vi "PVCamApp.vi"() -> ()   [LabVIEW 2019]
uses:
  <vilib>/Utility/miscctls.llb/LVMouseTypeDef.ctl
  Dependencies/PVCamNET.dll
  <vilib>/Analysis/coordinate.llb/2D Cartesian Coordinate Rotation (Scalar).vi
  SubVis/PVCamGlobalVariables.vi
  <vilib>/Instr/_visa.llb/VISA Configure Serial Port (Instr).vi
  Program Files/MetroCon-3.2/RepSend/R11CommLib-x64.dll
  <vilib>/Analysis/NI_AALPro.lvlib
panel:
  in  "FramesToCapture":u16=188
  in  "value":u16=700
  out "Map":picture
  out "Mouse":T1={"Mouse Position"={"X"=-1, "Y"=-1}, "Mouse Modifiers"={"Button Down"=FALSE, "Shift Mod"=FALSE, "Menu Mod"=FALSE, "Option Mod"=FALSE}}
  in  "ScreenMove":bool
  out "Angle":dbl=5.764762550937391
  out "Ratio":dbl=0.06396544799868786
  out "Shift2":dbl=-46.0
  out "Shift1":dbl=3014.0
  in  "Match":bool
  in  "map2":bool
  in  "map1":bool
  in  "Get2":bool
  in  "Get1":bool
  out "StageY2":i32=-305
  out "StageX2":i32=3018
  out "StageY1":i32=287
  out "StageX1":i32=-2846
  out "MapY2":i32=226
  out "MapX2":i32=590
  out "MapY1":i32=226
  out "MapX1":i32=213
  out "new picture":picture
  in  "StopX":bool
  in  "Path":path=path "C:/Users/Dell/Desktop/Map1.jpg"
  in  "LoadMap":bool
  in  "Stop":bool=TRUE
  out "Current PositionY":string="-2147431906" caption="Current PositionY:"
  out "Current PositionX":string="2147391745" caption="Current PositionX:"
  out "Choice 2":i32
  out "Choice":i32
  in  "Delete":bool
  in  "homeZ":bool
  in  "Goto":bool
  in  "Update":bool
  in  "ADDItem":bool
  in  "Multicolumn Listbox":i32[](listbox)=[0]
  in  "JogX-":bool
  in  "JogX+":bool
  out "Z motor connect":bool=TRUE
  out "XY motors connect":bool=TRUE
  out "appended path":path=path "C:/Users/Dell/Desktop/SIMImaging -电动平移台 -V4/PVCamNET_Collection1621317453_1973.tiff"
  in  "Numeric 2":i32=100
  out "Current PositionZ:":string="5661"
  in  "GoZ":bool
  in  "Relative MoveZ":string="3" caption="Relative Move:"
  in  "GoZ 2":bool
  in  "ZeroZ":bool
  out "Laser":bool[](array[boolean])=[FALSE, FALSE, TRUE]
  out "XBinning 3":u16
  out "YBinning 3":u16
  out "Exposure 2":u32
  out "millisecond timer value 3":u32=21169637
  out "XBinning 2":u16=1
  out "YBinning 2":u16=1
  in  "Camera Control":T2(tab)=enum."SIM Imaging"
  out "Dropped Frame":dbl
  out "Buffer Index":dbl
  in  "Scrollbar":i32(c297)=32
  in  "Exposure Time":dbl
  in  "Binning":string(combo)
  in  "X":u16
  in  "Width":u16
  in  "Y":u16
  in  "Height":u16
  in  "Full CCD":bool
  in  "Single Capture":bool
  in  "Live start":bool
  in  "Live stop":bool
  in  "Live status":bool
  in  "Get ROI":bool
  in  "Save Image to TIFF":bool
  out "Capturing":bool
  in  "Exposure Resolution":string(combo)
  out "8 Bit Histogram":i32[](graph)
  in  "Histogram On/Off":bool=TRUE
  out "?":string
  in  "Readout ports and speed":string(combo)
  in  "Gain":string(combo)
  in  "Sensor clearing mode":string(combo)
  in  "Clear Cycles":dbl
  in  "Trigger Out Behaviour":string(combo)
  in  "Trigger In Behaviour":string(combo)
  out "SLM connected":bool
  out "Order Count":u16=15
  out "Laser":bool=TRUE
  in  "L405nm":bool
  in  "L561nm":bool
  in  "Slide561":dbl(slide)=6.046511627906977 scale=0.0..100.0
  in  "Slide488":dbl(slide)=6.511627906976744 scale=0.0..100.0
  in  "Slide405":dbl(slide)=46.51162790697674 scale=0.0..100.0
  in  "VISA resource name":refnum<visa-resource-name>="COM5"
  in  "baud rate (9600)":u32=57600
  in  "L488nm":bool
  in  "GoY":bool
  in  "Relative MoveY":string="300" caption="Relative Move:"
  in  "GoX":bool
  in  "Relative MoveX":string="300" caption="Relative Move:"
  in  "GoX 2":bool
  in  "GoY 2":bool
  in  "VISA resource":refnum<visa-resource-name>="COM3"
  in  "baud rate (115200)":u32=115200
  out "LaserStage":bool=TRUE
  in  "ZeroX":bool
  in  "homeX":bool
  in  "homeY":bool
  in  "ZeroY":bool
  in  "ImagingMode":enum32{"WideField", "SIM"}(radio)=enum."SIM"
  in  "561nm":bool=TRUE
  in  "488nm":bool
  in  "405nm":bool
  in  "Delay time(ms)":i16=200
  in  "Z number":i16=2
  in  "Z step(counts)":string="0"
  out "time":dbl=7265.0
  in  "Laser Channel":u16(ring)=2 items=["405nm", "488nm", "561nm"]
  in  "AutoImaging":bool
  in  "milliseconds to wait":u32
  out "millisecond timer value":u32=21169637
  out "millisecond timer value 2":u32=21176902
  in  "Single Capture SLM":bool
  in  "after wait time":dbl=150.0 format="%#_13g"
  in  "before wait time":u32
  in  "folder":string="13"
  out "Numeric":i32
  out "Current Z":i32=2
  in  "Batch":enum32{"Single", "Batch"}(radio)
  out "LabVIEW app version":string
  out "PVCamNET version":string
  out "Trigger Mode":i32=1792
  out "Exposure":u32
  out "YBinning":u16
  out "XBinning":u16
  out "CC Min":u32
  out "CC Max":u32=65535
  out "Exp. out":i32
  out "Clearing modes":i32
  out "Full CCD Y":i32
  out "Full CCD Height":i32
  out "Full CCD Width":i32
  out "Full CCD X":i32
  out "Y Binning":u32=1
  out "X Binning":u32=1
  in  "Init":bool
  in  "Camera status":bool
  in  "Close Camera":bool
  in  "Open Camera":bool
  in  "Select Camera":string(combo)
  in  "Uninit":bool
  in  "PVCam indicator":bool
  out "PVCam version":string
  # "Z motor"
  # "Power(%)"
  # "Channel"
  # "X motor"
  # "Y motor"
  # "Laser Channel"
  # "250nm/step"
types:
  T1 = typedef "LVMouseTypeDef.ctl" = cluster{"Mouse Position":cluster{"X":i32, "Y":i32}, "Mouse Modifiers":cluster{"Button Down":bool, "Shift Mod":bool, "Menu Mod":bool, "Option Mod":bool}}
  T2 = enum32{"Basic", "Advanced", "SLM Control", "Laser Control", "Stage", "SIM Imaging"}
  T3 = typedef "LVPoint32TypeDef.ctl" = cluster{"Horizontal":i32, "Vertical":i32}
  T4 = typedef "LVRowAndColumnTypeDef.ctl" = cluster{"Row":i32, "Column":i32}
  T5 = typedef "imagedata.ctl" = cluster{"image type":i32, "image depth":i32, "image":u8[], "mask":u8[], "colors":u32[], "Rectangle":cluster{"left":i16, "top":i16, "right":i16, "bottom":i16}}
  T6 = cluster{"Buffer Index":refnum<vi>, "Dropped Frame":refnum<vi>, "Scrollbar":refnum<vi>}
  T7 = cluster{"Width":i16, "Style":enum32{"Solid", "Dash", "Dot", "DashDot", "DashDotDot"}}
  T8 = typedef "LVBoundsTypeDef.ctl" = cluster{"Width":u32, "Height":u32}
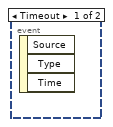
[diagram p2: hidden frame]
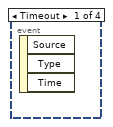
[diagram p3: hidden frame]
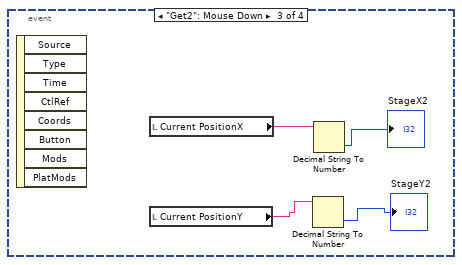
[diagram p4: hidden frame]
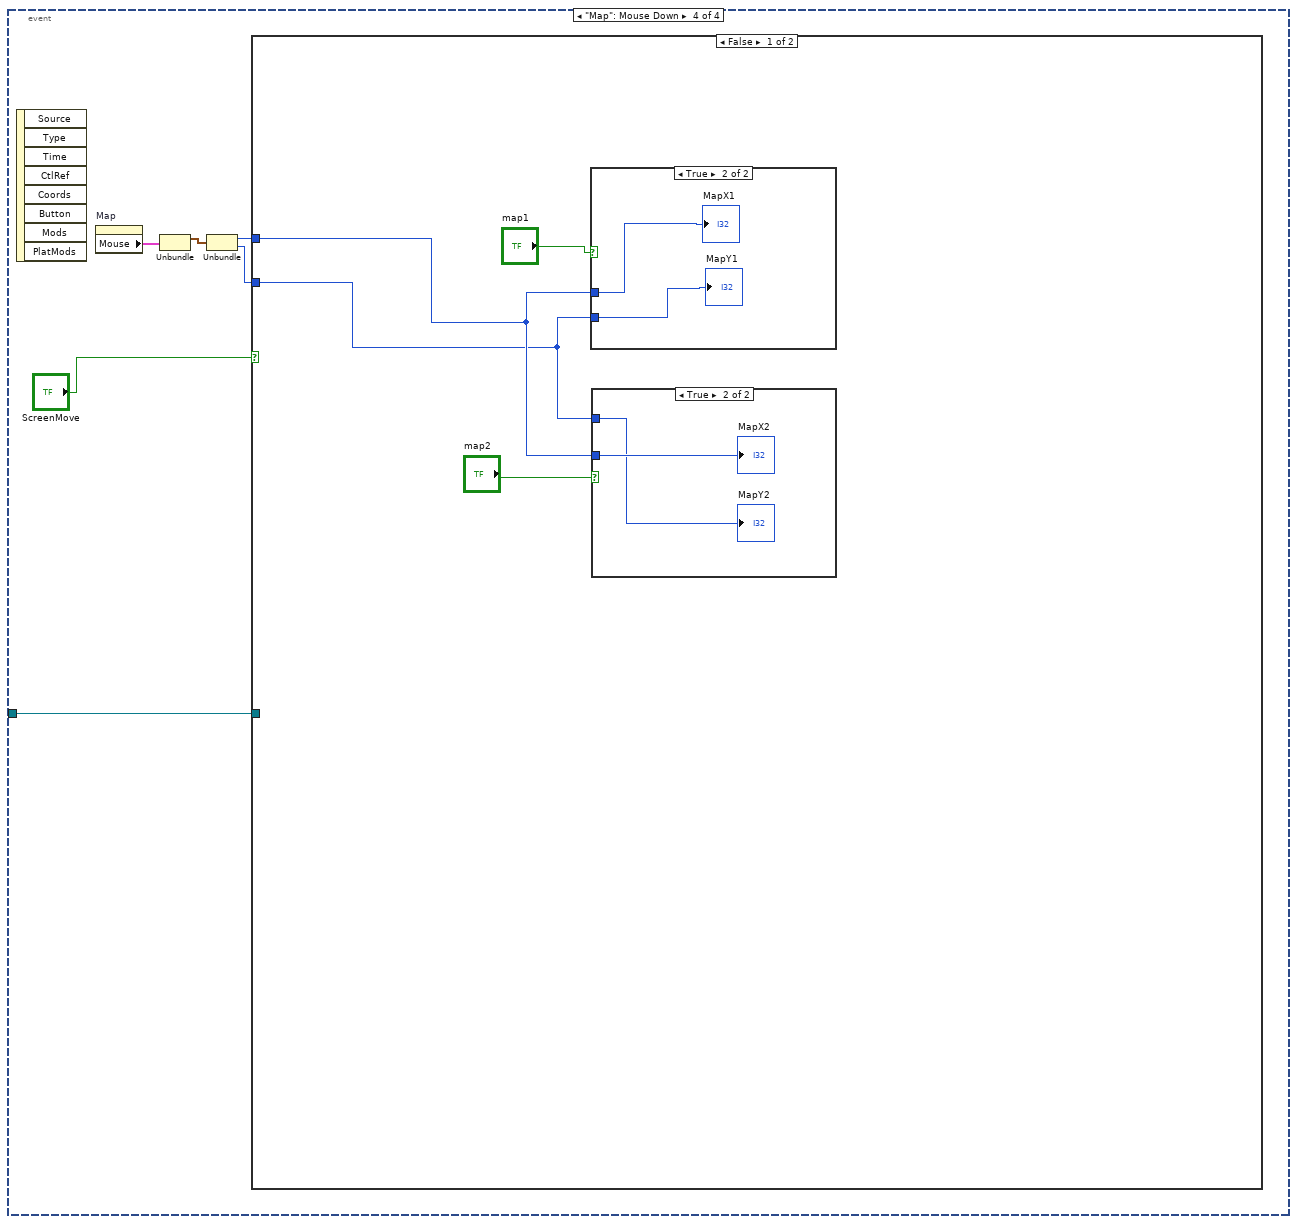
[diagram p5: hidden frame]
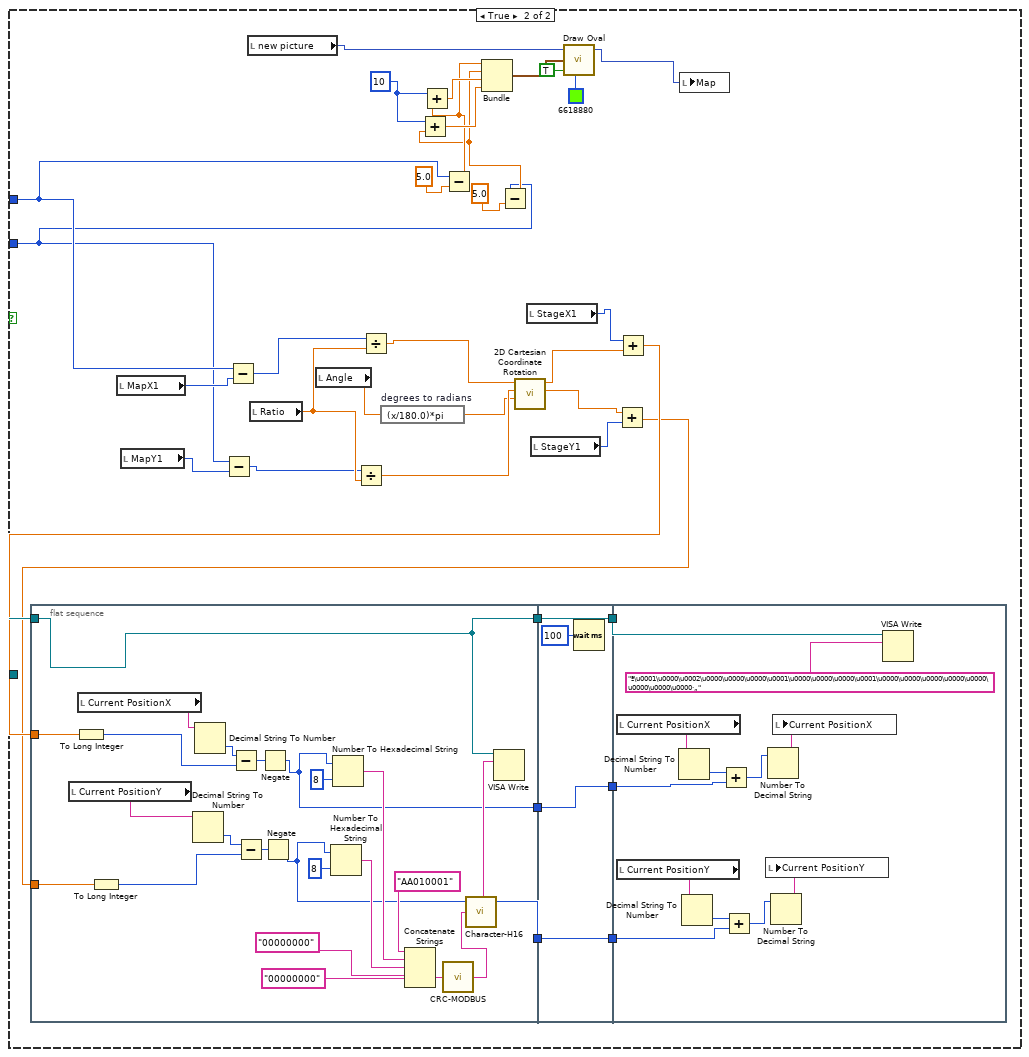
[diagram p8: hidden frame]
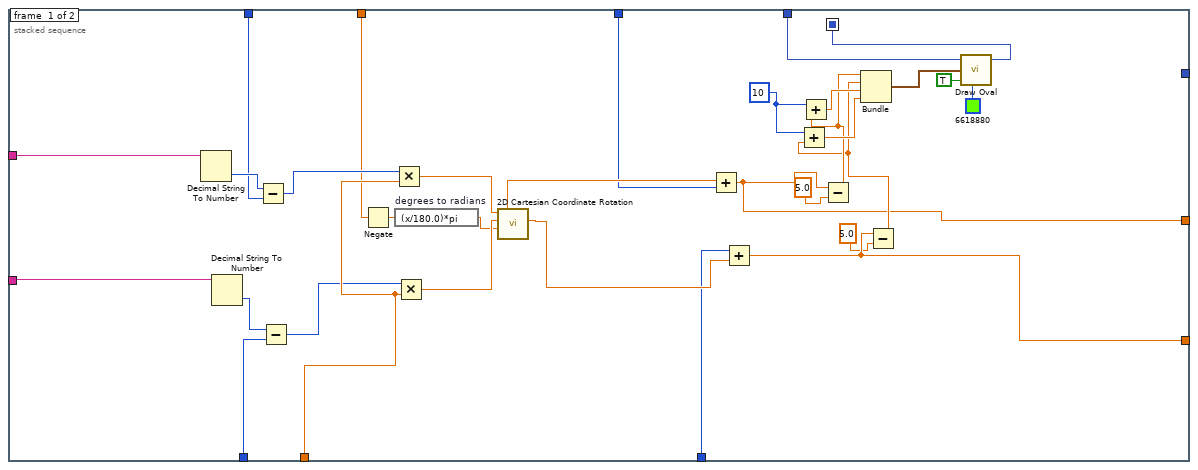
[diagram p9: hidden frame]
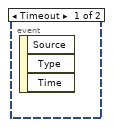
[diagram p10: hidden frame]
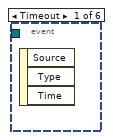
[diagram p11: hidden frame]
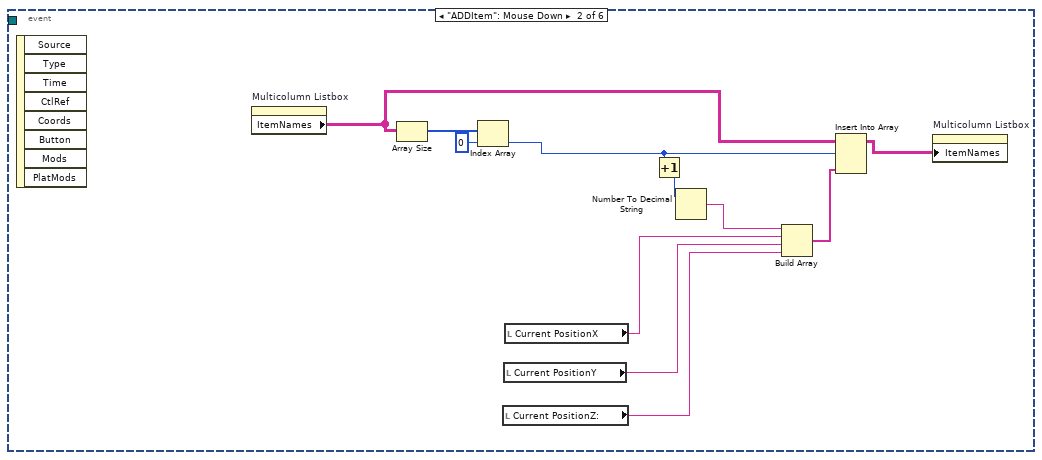
[diagram p12: hidden frame]
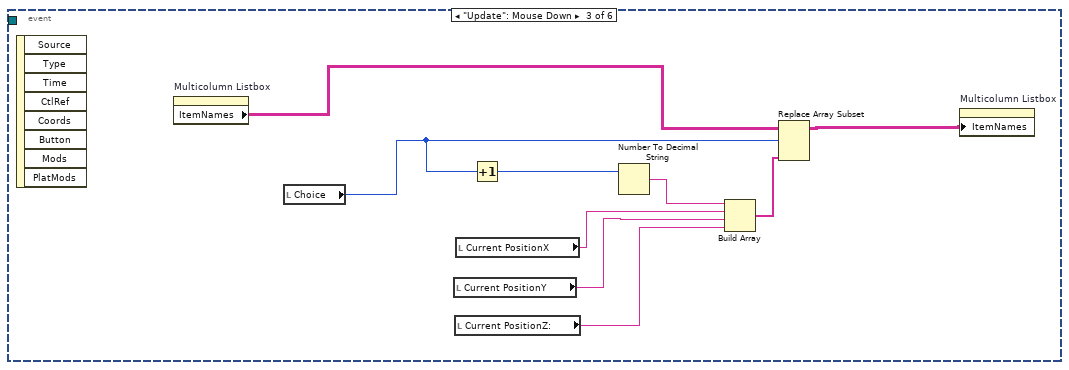
[diagram p13: hidden frame]
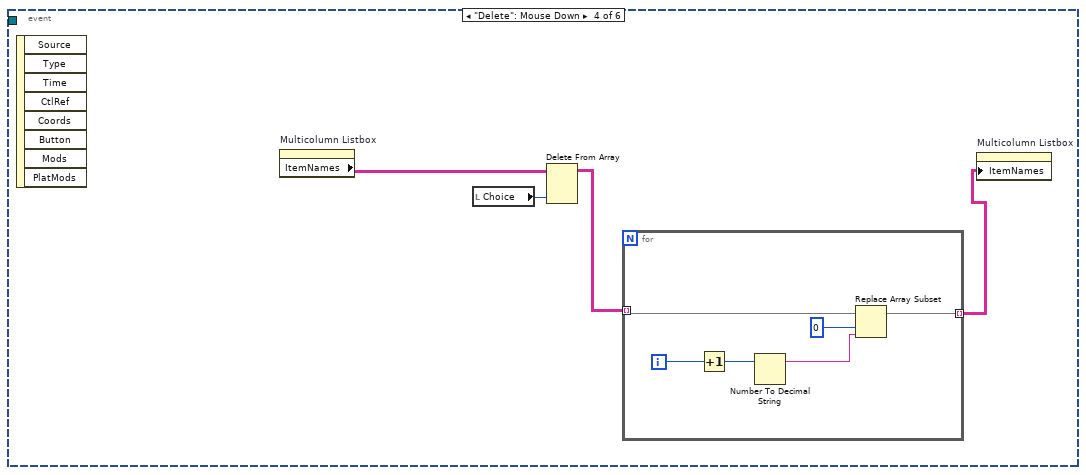
[diagram p14: hidden frame]
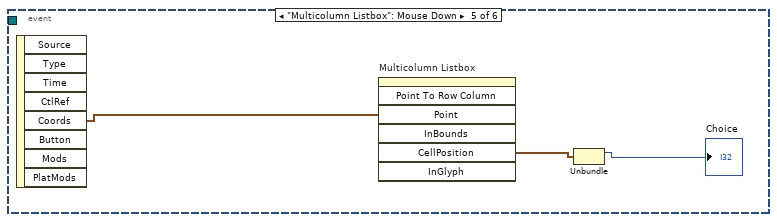
[diagram p15: hidden frame]
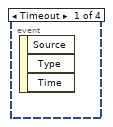
[diagram p16: hidden frame]
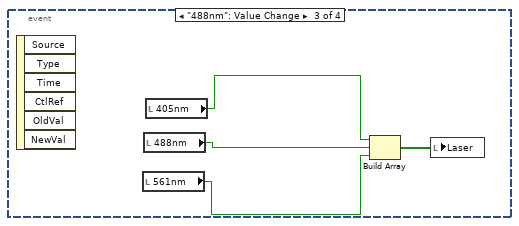
[diagram p17: hidden frame]
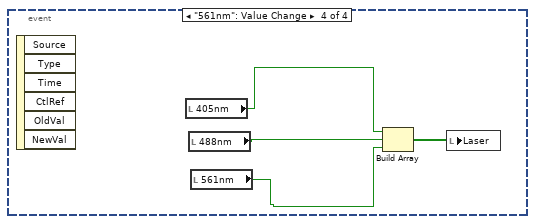
[diagram p18: hidden frame]
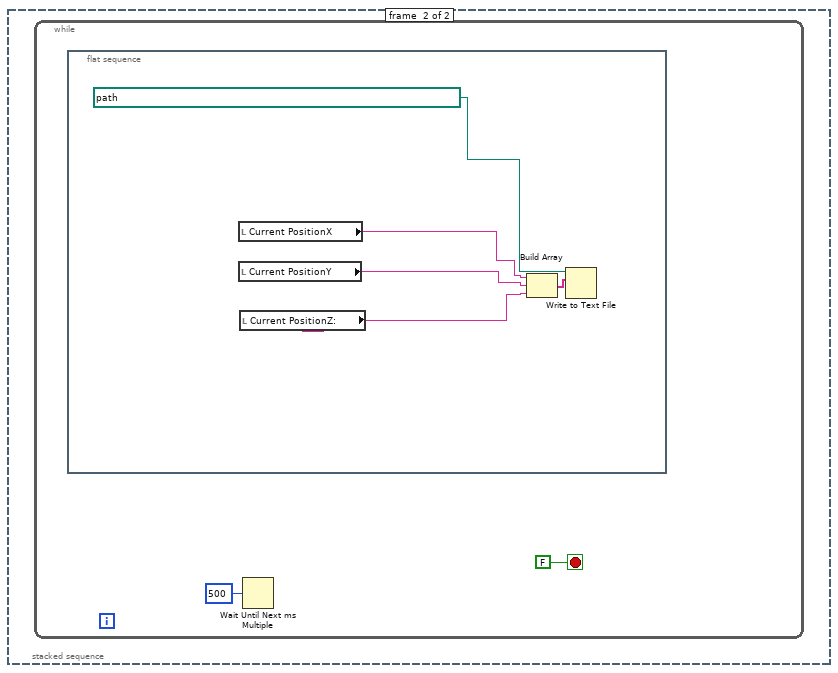
[diagram p19: hidden frame]
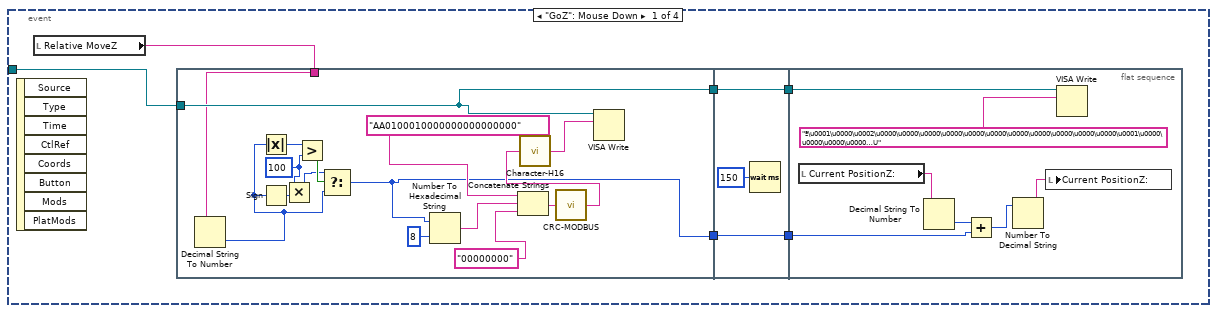
[diagram p20: hidden frame]
diagram:
  w23 = FALSE ("Histogram On/Off")
  w27 = FALSE ("Visible")
  # "camera"
  # "PVCamApp version"
  # "Debug"
  n1 = property class="Library"() -> ("Instance"=w14:refnum<k24>)  [unwired: 2 in, 2 out]
  n2 = invoke class="Library" method="LoadCameras"(reference=w14) -> (reference out=w13:refnum<k24>)  [unwired: 2 in, 2 out]
  n3 = call-poly "VISA Configure Serial Port"("VISA resource name"="VISA resource name", "baud rate (9600)"="baud rate (9600)", "data bits (8)"=u16 8) -> ("VISA resource name out"=w12:refnum<visa-resource-name>, "error out"=w18:errorcluster)  [unwired: 11 in]
  n4 = call <vilib>:"Simple Error Handler.vi"("error in (no error)"=w18) -> ("error?"=w19:bool)  [unwired: 4 in, 4 out]
  n5 = Not(x=w19) -> (.not. x?=→"Laser":bool)
  n6 = call-poly "VISA Configure Serial Port"("VISA resource name"="VISA resource", "baud rate (9600)"="baud rate (115200)", "data bits (8)"=u16 8) -> ("VISA resource name out"=w1:refnum<visa-resource-name>, "error out"=w5:errorcluster)  [unwired: 11 in]
  n7 = call <vilib>:"Simple Error Handler.vi"("error in (no error)"=w5) -> ("error?"=w6:bool)  [unwired: 4 in, 4 out]
  n8 = Not(x=w6) -> (.not. x?=→"LaserStage":bool)
  n9 = flat-sequence {
    tunnel: w12 -> [w30]
    frame #0 {
      n10 = while {
        tunnel: w30 -> [w32]
        stop <- FALSE stop-if-true
        n11 = event shown="[1] \"L488nm\": Value Change" {
          selector: _ -> [_ _ _ _ _ _]
          dyn-events: _ -> [_ _ _ _ _ _]
          timeout: _ -> [_ _ _ _ _ _]
          tunnel: w32 -> [w34 w42 w56 w69 w84 w99]
          event "L405nm": Value Change {
            n12 = event-data() -> ()  [unwired: 1 in, 6 out]
            n13 = local read "L405nm"() -> (w33:bool)
            n14 = Boolean To (0,1)(Boolean=w33) -> (0, 1=w40:i16)
            n15 = Number To Decimal String(number=w40) -> (decimal integer string=w38:string)  [unwired: 1 in]
            n16 = Concatenate Strings("L1O" ("write buffer"), w38, "E" ("write buffer"), "\r") -> (w35:string)
            n17 = VISA Write(VISA resource name=w34, write buffer=w35) -> ()  [unwired: 1 in, 3 out]
          }
          event "L488nm": Value Change {
            n18 = event-data() -> ()  [unwired: 1 in, 6 out]
            n19 = local read "L488nm"() -> (w41:bool)
            n20 = Boolean To (0,1)(Boolean=w41) -> (0, 1=w48:i16)
            n21 = Number To Decimal String(number=w48) -> (decimal integer string=w46:string)  [unwired: 1 in]
            n22 = Concatenate Strings("L2O" ("write buffer"), w46, "E" ("write buffer"), "\r") -> (w43:string)
            n23 = VISA Write(VISA resource name=w42, write buffer=w43) -> ()  [unwired: 1 in, 3 out]
          }
          event "L561nm": Value Change {
            n24 = event-data() -> ()  [unwired: 1 in, 6 out]
            n25 = local read "L561nm"() -> (w49:bool)
            n26 = Boolean To (0,1)(Boolean=w49) -> (0, 1=w55:i16)
            n27 = Number To Decimal String(number=w55) -> (decimal integer string=w53:string)  [unwired: 1 in]
            n28 = Concatenate Strings("L3O" ("write buffer"), w53, "E" ("write buffer"), "\r") -> (w50:string)
            n29 = VISA Write(VISA resource name=w56, write buffer=w50) -> ()  [unwired: 1 in, 3 out]
          }
          event "Slide405": Value Change {
            w63 = -14.0
            n30 = event-data() -> ()  [unwired: 1 in, 6 out]
            n31 = Subtract(x=16.2, y=w63) -> (x-y=w65:dbl)
            n32 = Multiply(x="Slide405", y=w65) -> (x*y=w60:dbl)
            n33 = Divide(x=w60, y=100.0) -> (x/y=w58:dbl)
            n34 = Add(x=w58, y=w63) -> (x+y=w61:dbl)
            n35 = Number To Fractional String(number=w61, precision (6)=i16 2) -> (F-format string=w66:string)  [unwired: 2 in]
            n36 = Concatenate Strings("L1D" ("write buffer"), w66, "E" ("write buffer"), "\r") -> (w71:string)
            n37 = VISA Write(VISA resource name=w69, write buffer=w71) -> ()  [unwired: 1 in, 3 out]
          }
          event "Slide488": Value Change {
            w79 = -15.0
            n38 = event-data() -> ()  [unwired: 1 in, 6 out]
            n39 = Subtract(x=17.3, y=w79) -> (x-y=w80:dbl)
            n40 = Multiply(x="Slide488", y=w80) -> (x*y=w76:dbl)
            n41 = Divide(x=w76, y=100.0) -> (x/y=w74:dbl)
            n42 = Add(x=w74, y=w79) -> (x+y=w77:dbl)
            n43 = Number To Fractional String(number=w77, precision (6)=i16 2) -> (F-format string=w81:string)  [unwired: 2 in]
            n44 = Concatenate Strings("L2D" ("write buffer"), w81, "E" ("write buffer"), "\r") -> (w86:string)
            n45 = VISA Write(VISA resource name=w84, write buffer=w86) -> ()  [unwired: 1 in, 3 out]
          }
          event "Slide561": Value Change {
            w94 = -15.0
            n46 = event-data() -> ()  [unwired: 1 in, 6 out]
            n47 = Subtract(x=19.3, y=w94) -> (x-y=w95:dbl)
            n48 = Multiply(x="Slide561", y=w95) -> (x*y=w91:dbl)
            n49 = Divide(x=w91, y=100.0) -> (x/y=w89:dbl)
            n50 = Add(x=w89, y=w94) -> (x+y=w92:dbl)
            n51 = Number To Fractional String(number=w92, precision (6)=i16 2) -> (F-format string=w96:string)  [unwired: 2 in]
            n52 = Concatenate Strings("L3D" ("write buffer"), w96, "E" ("write buffer"), "\r") -> (w101:string)
            n53 = VISA Write(VISA resource name=w99, write buffer=w101) -> ()  [unwired: 1 in, 3 out]
          }
        }
      }
    }
  }
  n54 = control-ref of="Clear Cycles"() -> ()  [unwired: 1 out]
  n55 = while {
    tunnel: w1 -> [w102]
    stop <- FALSE stop-if-true
    n56 = stacked-sequence {
      tunnel: w102 -> [w104]
      frame #0 {
        n57 = event shown="[3] \"homeX\": Mouse Down" {
          selector: _ -> [_ _ _ _]
          dyn-events: _ -> [_ _ _ _]
          timeout: _ -> [_ _ _ _]
          tunnel: w104 -> [w109 w142 _ w187]
          event "GoX": Mouse Down {
            n58 = event-data() -> ()  [unwired: 1 in, 8 out]
            n59 = local read "Relative MoveX"() -> (w110:string)
            n60 = flat-sequence {
              tunnel: w109 -> [w122]
              tunnel: [w122] -> w108
              tunnel: w110 -> [w121]
              tunnel: [w111] -> w105
              tunnel: w108 -> [w130]
              tunnel: [w130] -> w107
              tunnel: [w128] -> w106
              tunnel: w105 -> [w128]
              tunnel: w107 -> [w137]
              tunnel: w106 -> [w131]
              frame #0 {
                w115 = i16 800 ("width (-)")
                n61 = Decimal String To Number(string=w121) -> (number=w113:i32)  [unwired: 2 in, 1 out]
                n62 = Absolute Value(x=w113) -> (abs(x)=w118:i32)
                n63 = Sign(1:w113) -> (0:w114:i32)
                n64 = Multiply(x=w115, y=w114) -> (x*y=w116:i32)
                n65 = Greater?(x=w118, y=w115) -> (0:w117:bool)
                n66 = Select(t=w116, s=w117, f=w113) -> (s? t:f=w112:i32)
                n67 = Negate(x=w112) -> (-x=w111:i32)
                n68 = Number To Hexadecimal String(1:i16 8 ("width (-)"), 2:w111) -> (0:w125:string)
                n69 = Concatenate Strings("AA010001" ("write buffer"), w125, "000000000000000000000000" ("write buffer")) -> (w123:string)
                n70 = call "CRC-MODBUS.vi"("数据"=w123) -> ("数据+CRC"=w120:string)
                n71 = call "Character-H16.vi"("string"=w120) -> ("string 2"=w119:string)
                n72 = VISA Write(VISA resource name=w122, write buffer=w119) -> ()  [unwired: 1 in, 3 out]
              }
              frame #1 {
                n73 = Wait (ms)(milliseconds to wait=u32 150) -> ()  [unwired: 1 out]
              }
              frame #2 {
                n74 = local read "Current PositionX"() -> (w132:string)
                n75 = Decimal String To Number(string=w132) -> (number=w133:i32)  [unwired: 2 in, 1 out]
                n76 = Add(x=w133, y=w131) -> (x+y=w135:i32)
                n77 = VISA Write(VISA resource name=w137, write buffer="ª\u0001\u0000\u0002\u0000\u0000\u0000\u0001\u0000\u0000\u0000\u0000\u0000\u0000\u0000\u0000\u0000\u0000\u0000\u0000º\u0014") -> ()  [unwired: 1 in, 3 out]
                n78 = Number To Decimal String(number=w135) -> (decimal integer string=w134:string)  [unwired: 1 in]
                n79 = local write "Current PositionX"(w134) -> ()
              }
              frame #3 {
              }
            }
          }
          event "GoX 2": Mouse Down {
            n80 = event-data() -> ()  [unwired: 1 in, 8 out]
            n81 = local read "Relative MoveX"() -> (w143:string)
            n82 = flat-sequence {
              tunnel: w142 -> [w154]
              tunnel: [w154] -> w141
              tunnel: w143 -> [w153]
              tunnel: [w144] -> w139
              tunnel: w141 -> [w162]
              tunnel: [w162] -> w140
              tunnel: w139 -> [w160]
              tunnel: [w160] -> w138
              tunnel: w140 -> [w169]
              tunnel: w138 -> [w163]
              frame #0 {
                w147 = i16 800 ("width (-)")
                n83 = Decimal String To Number(string=w153) -> (number=w145:i32)  [unwired: 2 in, 1 out]
                n84 = Absolute Value(x=w145) -> (abs(x)=w150:i32)
                n85 = Sign(1:w145) -> (0:w146:i32)
                n86 = Multiply(x=w147, y=w146) -> (x*y=w148:i32)
                n87 = Greater?(x=w150, y=w147) -> (0:w149:bool)
                n88 = Select(t=w148, s=w149, f=w145) -> (s? t:f=w144:i32)
                n89 = Number To Hexadecimal String(1:i16 8 ("width (-)"), 2:w144) -> (0:w157:string)
                n90 = Concatenate Strings("AA010001" ("write buffer"), w157, "000000000000000000000000" ("write buffer")) -> (w155:string)
                n91 = call "CRC-MODBUS.vi"("数据"=w155) -> ("数据+CRC"=w152:string)
                n92 = call "Character-H16.vi"("string"=w152) -> ("string 2"=w151:string)
                n93 = VISA Write(VISA resource name=w154, write buffer=w151) -> ()  [unwired: 1 in, 3 out]
              }
              frame #1 {
                n94 = Wait (ms)(milliseconds to wait=u32 150) -> ()  [unwired: 1 out]
              }
              frame #2 {
                n95 = local read "Current PositionX"() -> (w166:string)
                n96 = Decimal String To Number(string=w166) -> (number=w165:i32)  [unwired: 2 in, 1 out]
                n97 = Add(x=w165, y=w163) -> (x+y=w164:i32)
                n98 = VISA Write(VISA resource name=w169, write buffer="ª\u0001\u0000\u0002\u0000\u0000\u0000\u0001\u0000\u0000\u0000\u0000\u0000\u0000\u0000\u0000\u0000\u0000\u0000\u0000º\u0014") -> ()  [unwired: 1 in, 3 out]
                n99 = Number To Decimal String(number=w164) -> (decimal integer string=w167:string)  [unwired: 1 in]
                n100 = local write "Current PositionX"(w167) -> ()
              }
            }
          }
          event "ZeroX": Mouse Down {
            n101 = event-data() -> ()  [unwired: 1 in, 8 out]
            n102 = flat-sequence {
              tunnel: [w184] -> w183
              frame #0 {
                n103 = local read "Current PositionX"() -> (w184:string)
              }
              frame #1 {
                n104 = Wait (ms)(milliseconds to wait=u32 150) -> ()  [unwired: 1 out]
              }
              frame #2 {
                n105 = local write "Current PositionX"("0") -> ()
              }
            }
            n106 = property on="Multicolumn Listbox" class="MCListbox (strict)"() -> ("ItemNames"=w174:string[][])  [unwired: 2 in, 2 out]
            n107 = Index Array(array=w174, index (col)=1 ("index")) -> (element=w178:string[])  [unwired: 1 in]
            n108 = Decimal String To Number(string=w178) -> (number=w177:i32[])  [unwired: 2 in, 1 out]
            n109 = Decimal String To Number(string=w183) -> (number=w176:i32)  [unwired: 2 in, 1 out]
            n110 = Subtract(x=w177, y=w176) -> (x-y=w175:i32[])
            n111 = local read "StageX2"() -> (w180:i32)
            n112 = local read "StageX1"() -> (w182:i32)
            n113 = Number To Decimal String(number=w175) -> (decimal integer string=w172:string[])  [unwired: 1 in]
            n114 = Subtract(x=w180, y=w176) -> (x-y=w179:i32)
            n115 = Subtract(x=w182, y=w176) -> (x-y=w181:i32)
            n116 = Replace Array Subset(array=w174, new element=w172, index (col)=1 ("index")) -> (w170:string[][])  [unwired: 1 in]
            n117 = local write "StageX1"(w181) -> ()
            n118 = local write "StageX2"(w179) -> ()
            n119 = property on="Multicolumn Listbox" class="MCListbox (strict)"("ItemNames"=w170) -> ()  [unwired: 2 in, 2 out]
          }
          event "homeX": Mouse Down {
            n120 = event-data() -> ()  [unwired: 1 in, 8 out]
            n121 = local read "Current PositionX"() -> (w188:string)
            n122 = flat-sequence {
              tunnel: w187 -> [w198]
              tunnel: [w198] -> w192
              tunnel: [w193] -> w191
              tunnel: w188 -> [w195]
              tunnel: w192 -> [w206]
              tunnel: [w206] -> w190
              tunnel: w191 -> [w204]
              tunnel: [w204] -> w189
              tunnel: w190 -> [w213]
              tunnel: w189 -> [w208]
              frame #0 {
                n123 = Decimal String To Number(string=w195) -> (number=w194:i32)  [unwired: 2 in, 1 out]
                n124 = Negate(x=w194) -> (-x=w193:i32)
                n125 = Number To Hexadecimal String(1:i16 8 ("width (-)"), 2:w193) -> (0:w201:string)
                n126 = Concatenate Strings("AA010001" ("write buffer"), w201, "000000000000000000000000" ("write buffer")) -> (w199:string)
                n127 = call "CRC-MODBUS.vi"("数据"=w199) -> ("数据+CRC"=w197:string)
                n128 = call "Character-H16.vi"("string"=w197) -> ("string 2"=w196:string)
                n129 = VISA Write(VISA resource name=w198, write buffer=w196) -> ()  [unwired: 1 in, 3 out]
              }
              frame #1 {
                n130 = Wait (ms)(milliseconds to wait=u32 150) -> ()  [unwired: 1 out]
              }
              frame #2 {
                n131 = local read "Current PositionX"() -> (w207:string)
                n132 = Decimal String To Number(string=w207) -> (number=w210:i32)  [unwired: 2 in, 1 out]
                n133 = Add(x=w210, y=w208) -> (x+y=w209:i32)
                n134 = VISA Write(VISA resource name=w213, write buffer="ª\u0001\u0000\u0002\u0000\u0000\u0000\u0001\u0000\u0000\u0000\u0000\u0000\u0000\u0000\u0000\u0000\u0000\u0000\u0000º\u0014") -> ()  [unwired: 1 in, 3 out]
                n135 = Number To Decimal String(number=w209) -> (decimal integer string=w211:string)  [unwired: 1 in]
                n136 = local write "Current PositionX"(w211) -> ()
              }
            }
          }
        }
      }
    }
  }
  n137 = while {
    tunnel: w1 -> [w214]
    stop <- FALSE stop-if-true
    n138 = stacked-sequence {
      tunnel: w214 -> [w216]
      frame #0 {
        n139 = event shown="[2] \"ZeroY\": Mouse Down" {
          selector: _ -> [_ _ _ _]
          dyn-events: _ -> [_ _ _ _]
          timeout: _ -> [_ _ _ _]
          tunnel: w216 -> [w222 w254 _ w300]
          event "GoY": Mouse Down {
            n140 = event-data() -> ()  [unwired: 1 in, 8 out]
            n141 = local read "Relative MoveY"() -> (w221:string)
            n142 = flat-sequence {
              tunnel: w222 -> [w233]
              tunnel: [w233] -> w220
              tunnel: w221 -> [w232]
              tunnel: [w223] -> w217
              tunnel: w220 -> [w241]
              tunnel: [w241] -> w219
              tunnel: [w239] -> w218
              tunnel: w217 -> [w239]
              tunnel: w219 -> [w248]
              tunnel: w218 -> [w242]
              frame #0 {
                w226 = i16 800 ("width (-)")
                n143 = Decimal String To Number(string=w232) -> (number=w224:i32)  [unwired: 2 in, 1 out]
                n144 = Absolute Value(x=w224) -> (abs(x)=w229:i32)
                n145 = Sign(1:w224) -> (0:w225:i32)
                n146 = Multiply(x=w226, y=w225) -> (x*y=w227:i32)
                n147 = Greater?(x=w229, y=w226) -> (0:w228:bool)
                n148 = Select(t=w227, s=w228, f=w224) -> (s? t:f=w223:i32)
                n149 = Number To Hexadecimal String(1:i16 8 ("width (-)"), 2:w223) -> (0:w236:string)
                n150 = Concatenate Strings("AA01000100000000" ("write buffer"), w236, "0000000000000000" ("write buffer")) -> (w234:string)
                n151 = call "CRC-MODBUS.vi"("数据"=w234) -> ("数据+CRC"=w231:string)
                n152 = call "Character-H16.vi"("string"=w231) -> ("string 2"=w230:string)
                n153 = VISA Write(VISA resource name=w233, write buffer=w230) -> ()  [unwired: 1 in, 3 out]
              }
              frame #1 {
                n154 = Wait (ms)(milliseconds to wait=u32 150) -> ()  [unwired: 1 out]
              }
              frame #2 {
                n155 = local read "Current PositionY"() -> (w244:string)
                n156 = Decimal String To Number(string=w244) -> (number=w245:i32)  [unwired: 2 in, 1 out]
                n157 = Add(x=w245, y=w242) -> (x+y=w246:i32)
                n158 = VISA Write(VISA resource name=w248, write buffer="ª\u0001\u0000\u0002\u0000\u0000\u0000\u0000\u0000\u0000\u0000\u0001\u0000\u0000\u0000\u0000\u0000\u0000\u0000\u0000µ\u0005") -> ()  [unwired: 1 in, 3 out]
                n159 = Number To Decimal String(number=w246) -> (decimal integer string=w243:string)  [unwired: 1 in]
                n160 = local write "Current PositionY"(w243) -> ()
              }
            }
          }
          event "GoY 2": Mouse Down {
            n161 = local read "Relative MoveY"() -> (w253:string)
            n162 = event-data() -> ()  [unwired: 1 in, 8 out]
            n163 = flat-sequence {
              tunnel: w254 -> [w271]
              tunnel: [w271] -> w252
              tunnel: w253 -> [w270]
              tunnel: [w255] -> w249
              tunnel: w252 -> [w276]
              tunnel: [w276] -> w251
              tunnel: [w274] -> w250
              tunnel: w249 -> [w274]
              tunnel: w251 -> [w283]
              tunnel: w250 -> [w277]
              frame #0 {
                w258 = i16 800 ("width (-)")
                n164 = Decimal String To Number(string=w270) -> (number=w256:i32)  [unwired: 2 in, 1 out]
                n165 = Absolute Value(x=w256) -> (abs(x)=w262:i32)
                n166 = Sign(1:w256) -> (0:w257:i32)
                n167 = Multiply(x=w258, y=w257) -> (x*y=w259:i32)
                n168 = Greater?(x=w262, y=w258) -> (0:w261:bool)
                n169 = Select(t=w259, s=w261, f=w256) -> (s? t:f=w260:i32)
                n170 = Negate(x=w260) -> (-x=w255:i32)
                n171 = Number To Hexadecimal String(1:i16 8 ("width (-)"), 2:w255) -> (0:w267:string)
                n172 = Concatenate Strings("AA010001" ("write buffer"), "00000000" ("write buffer"), w267, "00000000" ("write buffer"), "00000000" ("write buffer")) -> (w272:string)
                n173 = call "CRC-MODBUS.vi"("数据"=w272) -> ("数据+CRC"=w264:string)
                n174 = call "Character-H16.vi"("string"=w264) -> ("string 2"=w263:string)
                n175 = VISA Write(VISA resource name=w271, write buffer=w263) -> ()  [unwired: 1 in, 3 out]
              }
              frame #1 {
                n176 = Wait (ms)(milliseconds to wait=u32 150) -> ()  [unwired: 1 out]
              }
              frame #2 {
                n177 = local read "Current PositionY"() -> (w278:string)
                n178 = Decimal String To Number(string=w278) -> (number=w280:i32)  [unwired: 2 in, 1 out]
                n179 = Add(x=w280, y=w277) -> (x+y=w281:i32)
                n180 = Number To Decimal String(number=w281) -> (decimal integer string=w279:string)  [unwired: 1 in]
                n181 = VISA Write(VISA resource name=w283, write buffer="ª\u0001\u0000\u0002\u0000\u0000\u0000\u0000\u0000\u0000\u0000\u0001\u0000\u0000\u0000\u0000\u0000\u0000\u0000\u0000µ\u0005") -> ()  [unwired: 1 in, 3 out]
                n182 = local write "Current PositionY"(w279) -> ()
              }
            }
          }
          event "ZeroY": Mouse Down {
            n183 = event-data() -> ()  [unwired: 1 in, 8 out]
            n184 = flat-sequence {
              tunnel: [w298] -> w297
              frame #0 {
                n185 = local read "Current PositionY"() -> (w298:string)
              }
              frame #1 {
                n186 = local write "Current PositionY"("0") -> ()
              }
            }
            n187 = property on="Multicolumn Listbox" class="MCListbox (strict)"() -> ("ItemNames"=w287:string[][])  [unwired: 2 in, 2 out]
            n188 = Index Array(array=w287, index (col)=2 ("index")) -> (element=w292:string[])  [unwired: 1 in]
            n189 = Decimal String To Number(string=w292) -> (number=w291:i32[])  [unwired: 2 in, 1 out]
            n190 = Decimal String To Number(string=w297) -> (number=w286:i32)  [unwired: 2 in, 1 out]
            n191 = Subtract(x=w291, y=w286) -> (x-y=w290:i32[])
            n192 = Number To Decimal String(number=w290) -> (decimal integer string=w288:string[])  [unwired: 1 in]
            n193 = local read "StageY2"() -> (w295:i32)
            n194 = local read "StageY1"() -> (w296:i32)
            n195 = Replace Array Subset(array=w287, new element=w288, index (col)=2 ("index")) -> (w284:string[][])  [unwired: 1 in]
            n196 = Subtract(x=w295, y=w286) -> (x-y=w294:i32)
            n197 = Subtract(x=w296, y=w286) -> (x-y=w293:i32)
            n198 = local write "StageY1"(w293) -> ()
            n199 = property on="Multicolumn Listbox" class="MCListbox (strict)"("ItemNames"=w284) -> ()  [unwired: 2 in, 2 out]
            n200 = local write "StageY2"(w294) -> ()
          }
          event "homeY": Mouse Down {
            n201 = event-data() -> ()  [unwired: 1 in, 8 out]
            n202 = local read "Current PositionY"() -> (w301:string)
            n203 = flat-sequence {
              tunnel: w300 -> [w311]
              tunnel: [w311] -> w305
              tunnel: [w306] -> w304
              tunnel: w301 -> [w308]
              tunnel: w305 -> [w319]
              tunnel: [w319] -> w303
              tunnel: [w317] -> w302
              tunnel: w304 -> [w317]
              tunnel: w303 -> [w326]
              tunnel: w302 -> [w320]
              frame #0 {
                n204 = Decimal String To Number(string=w308) -> (number=w307:i32)  [unwired: 2 in, 1 out]
                n205 = Negate(x=w307) -> (-x=w306:i32)
                n206 = Number To Hexadecimal String(1:i16 8 ("width (-)"), 2:w306) -> (0:w314:string)
                n207 = Concatenate Strings("AA01000100000000" ("write buffer"), w314, "0000000000000000" ("write buffer")) -> (w312:string)
                n208 = call "CRC-MODBUS.vi"("数据"=w312) -> ("数据+CRC"=w310:string)
                n209 = call "Character-H16.vi"("string"=w310) -> ("string 2"=w309:string)
                n210 = VISA Write(VISA resource name=w311, write buffer=w309) -> ()  [unwired: 1 in, 3 out]
              }
              frame #1 {
                n211 = Wait (ms)(milliseconds to wait=u32 100) -> ()  [unwired: 1 out]
              }
              frame #2 {
                n212 = local read "Current PositionY"() -> (w322:string)
                n213 = Decimal String To Number(string=w322) -> (number=w323:i32)  [unwired: 2 in, 1 out]
                n214 = Add(x=w323, y=w320) -> (x+y=w324:i32)
                n215 = VISA Write(VISA resource name=w326, write buffer="ª\u0001\u0000\u0002\u0000\u0000\u0000\u0000\u0000\u0000\u0000\u0001\u0000\u0000\u0000\u0000\u0000\u0000\u0000\u0000µ\u0005") -> ()  [unwired: 1 in, 3 out]
                n216 = Number To Decimal String(number=w324) -> (decimal integer string=w321:string)  [unwired: 1 in]
                n217 = local write "Current PositionY"(w321) -> ()
              }
            }
          }
        }
      }
    }
  }
  n218 = while {
    tunnel: w1 -> [w327]
    stop <- FALSE stop-if-true
    n219 = event shown="[5] \"Goto\": Mouse Down" {
      selector: _ -> [_ _ _ _ _ _]
      dyn-events: _ -> [_ _ _ _ _ _]
      timeout: _ -> [_ _ _ _ _ _]
      tunnel: w327 -> [_ _ _ _ _ w368]
      event Timeout {
        n220 = event-data() -> ()  [unwired: 1 in, 3 out]
      }
      event "ADDItem": Mouse Down {
        n221 = event-data() -> ()  [unwired: 1 in, 8 out]
        n222 = property on="Multicolumn Listbox" class="MCListbox (strict)"() -> ("ItemNames"=w338:string[][])  [unwired: 2 in, 2 out]
        n223 = Array Size(array=w338) -> (size(s)=w339:i32[])
        n224 = Index Array(array=w339, index=0) -> (element=w330:i32)
        n225 = local read "Current PositionZ:"() -> (w334:string)
        n226 = local read "Current PositionY"() -> (w335:string)
        n227 = local read "Current PositionX"() -> (w336:string)
        n228 = Increment(x=w330) -> (x+1=w329:i32)
        n229 = Number To Decimal String(number=w329) -> (decimal integer string=w337:string)  [unwired: 1 in]
        n230 = Build Array(w337, w336, w335, w334) -> (w333:string[])
        n231 = Insert Into Array(array=w338, index (row)=w330, new element=w333) -> (w332:string[][])  [unwired: 1 in]
        n232 = property on="Multicolumn Listbox" class="MCListbox (strict)"("ItemNames"=w332) -> ()  [unwired: 2 in, 2 out]
      }
      event "Update": Mouse Down {
        n233 = event-data() -> ()  [unwired: 1 in, 8 out]
        n234 = property on="Multicolumn Listbox" class="MCListbox (strict)"() -> ("ItemNames"=w346:string[][])  [unwired: 2 in, 2 out]
        n235 = local read "Choice"() -> (w344:i32)
        n236 = local read "Current PositionY"() -> (w342:string)
        n237 = local read "Current PositionZ:"() -> (w341:string)
        n238 = local read "Current PositionX"() -> (w343:string)
        n239 = Increment(x=w344) -> (x+1=w340:i32)
        n240 = Number To Decimal String(number=w340) -> (decimal integer string=w348:string)  [unwired: 1 in]
        n241 = Build Array(w348, w343, w342, w341) -> (w347:string[])
        n242 = Replace Array Subset(array=w346, new element=w347, index (row)=w344) -> (w345:string[][])  [unwired: 1 in]
        n243 = property on="Multicolumn Listbox" class="MCListbox (strict)"("ItemNames"=w345) -> ()  [unwired: 2 in, 2 out]
      }
      event "Delete": Mouse Down {
        n244 = event-data() -> ()  [unwired: 1 in, 8 out]
        n245 = property on="Multicolumn Listbox" class="MCListbox (strict)"() -> ("ItemNames"=w352:string[][])  [unwired: 2 in, 2 out]
        n246 = local read "Choice"() -> (w351:i32)
        n247 = Delete From Array(array=w352, index (row)=w351) -> (array with subset deleted=w350:string[][])  [unwired: 2 in, 1 out]
        n248 = for {
          tunnel: w350 -> [w358] mode=indexing
          tunnel: [w355] -> w349 mode=indexing
          i -> [w356]
          n249 = Increment(x=w356) -> (x+1=w354:i32)
          n250 = Number To Decimal String(number=w354) -> (decimal integer string=w353:string)  [unwired: 1 in]
          n251 = Replace Array Subset(array=w358, new element=w353, index=i16 0 ("width (-)")) -> (w355:string[])
        }
        n252 = property on="Multicolumn Listbox" class="MCListbox (strict)"("ItemNames"=w349) -> ()  [unwired: 2 in, 2 out]
      }
      event "Multicolumn Listbox": Mouse Down {
        n253 = event-data() -> ("Coords"=w360:T3)  [unwired: 1 in, 7 out]
        n254 = invoke on="Multicolumn Listbox" class="MCListbox (strict)" method="Point To Row Column"("Point"=w360) -> ("CellPosition"=w361:T4)  [unwired: 6 in, 6 out]
        n255 = Unbundle(w361) -> ("Row"=→"Choice":i32)  [unwired: 1 out]
      }
      event "Goto": Mouse Down {
        n256 = event-data() -> ()  [unwired: 1 in, 8 out]
        n257 = property on="Multicolumn Listbox" class="MCListbox (strict)"() -> ("ItemNames"=w379:string[][])  [unwired: 2 in, 2 out]
        n258 = local read "Choice"() -> (w378:i32)
        n259 = Index Array(array=w379, index (row)=w378) -> (element=w377:string[])  [unwired: 1 in]
        n260 = Index Array(array=w377, index #1=i16 1 ("width (-)"), index #2=i16 2 ("width (-)"), index #3=i16 3 ("width (-)")) -> (element #1=w366:string, element #2=w367:string, element #3=w369:string)
        n261 = flat-sequence {
          tunnel: [w402] -> _
          tunnel: [w402] -> w373
          tunnel: [w380] -> w372
          tunnel: w369 -> [w403]
          tunnel: w368 -> [w402]
          tunnel: w367 -> [w390]
          tunnel: w366 -> [w389]
          tunnel: [w381] -> w364
          tunnel: [w382] -> w362
          tunnel: w373 -> [w414]
          tunnel: [w414] -> w371
          tunnel: [w412] -> w370
          tunnel: w372 -> [w412]
          tunnel: [w411] -> w365
          tunnel: w364 -> [w411]
          tunnel: [w410] -> w363
          tunnel: w362 -> [w410]
          tunnel: w371 -> [w431]
          tunnel: w370 -> [w425]
          tunnel: w365 -> [w420]
          tunnel: w363 -> [w419]
          frame #0 {
            n262 = local read "Current PositionZ:"() -> (w400:string)
            n263 = local read "Current PositionY"() -> (w383:string)
            n264 = local read "Current PositionX"() -> (w384:string)
            n265 = Decimal String To Number(string=w403) -> (number=w398:i32)  [unwired: 2 in, 1 out]
            n266 = Decimal String To Number(string=w400) -> (number=w399:i32)  [unwired: 2 in, 1 out]
            n267 = Decimal String To Number(string=w390) -> (number=w394:i32)  [unwired: 2 in, 1 out]
            n268 = Decimal String To Number(string=w389) -> (number=w391:i32)  [unwired: 2 in, 1 out]
            n269 = Subtract(x=w399, y=w398) -> (x-y=w397:i32)
            n270 = Decimal String To Number(string=w383) -> (number=w395:i32)  [unwired: 2 in, 1 out]
            n271 = Decimal String To Number(string=w384) -> (number=w392:i32)  [unwired: 2 in, 1 out]
            n272 = Negate(x=w397) -> (-x=w380:i32)
            n273 = Subtract(x=w392, y=w391) -> (x-y=w385:i32)
            n274 = Subtract(x=w395, y=w394) -> (x-y=w386:i32)
            n275 = Negate(x=w385) -> (-x=w382:i32)
            n276 = Negate(x=w386) -> (-x=w381:i32)
            n277 = Number To Hexadecimal String(1:i16 8 ("width (-)"), 2:w380) -> (0:w404:string)
            n278 = Number To Hexadecimal String(1:i16 8 ("width (-)"), 2:w381) -> (0:w388:string)
            n279 = Number To Hexadecimal String(1:i16 8 ("width (-)"), 2:w382) -> (0:w387:string)
            n280 = Concatenate Strings("AA010001" ("write buffer"), w387, w388, w404, "00000000" ("write buffer")) -> (w407:string)
            n281 = call "CRC-MODBUS.vi"("数据"=w407) -> ("数据+CRC"=w406:string)
            n282 = call "Character-H16.vi"("string"=w406) -> ("string 2"=w405:string)
            n283 = VISA Write(VISA resource name=w402, write buffer=w405) -> ()  [unwired: 1 in, 3 out]
          }
          frame #1 {
            n284 = Wait (ms)(milliseconds to wait=u32 100) -> ()  [unwired: 1 out]
          }
          frame #2 {
            n285 = local read "Current PositionX"() -> (w416:string)
            n286 = local read "Current PositionY"() -> (w417:string)
            n287 = local read "Current PositionZ:"() -> (w427:string)
            n288 = Decimal String To Number(string=w416) -> (number=w421:i32)  [unwired: 2 in, 1 out]
            n289 = Decimal String To Number(string=w417) -> (number=w423:i32)  [unwired: 2 in, 1 out]
            n290 = Decimal String To Number(string=w427) -> (number=w428:i32)  [unwired: 2 in, 1 out]
            n291 = Add(x=w421, y=w419) -> (x+y=w422:i32)
            n292 = Add(x=w423, y=w420) -> (x+y=w424:i32)
            n293 = Add(x=w428, y=w425) -> (x+y=w429:i32)
            n294 = Number To Decimal String(number=w422) -> (decimal integer string=w415:string)  [unwired: 1 in]
            n295 = local write "Current PositionX"(w415) -> ()
            n296 = Number To Decimal String(number=w424) -> (decimal integer string=w418:string)  [unwired: 1 in]
            n297 = local write "Current PositionY"(w418) -> ()
            n298 = Number To Decimal String(number=w429) -> (decimal integer string=w426:string)  [unwired: 1 in]
            n299 = local write "Current PositionZ:"(w426) -> ()
            n300 = VISA Write(VISA resource name=w431, write buffer="ª\u0001\u0000\u0002\u0000\u0000\u0000\u0001\u0000\u0000\u0000\u0001\u0000\u0000\u0000\u0001\u0000\u0000\u0000\u0000ŠD") -> ()  [unwired: 1 in, 3 out]
          }
        }
      }
    }
  }
  n301 = while {
    stop <- FALSE stop-if-true
    n302 = event shown="[1] \"405nm\": Value Change" {
      selector: _ -> [_ _ _ _]
      dyn-events: _ -> [_ _ _ _]
      timeout: _ -> [_ _ _ _]
      event Timeout {
        n303 = event-data() -> ()  [unwired: 1 in, 3 out]
      }
      event "405nm": Value Change {
        n304 = event-data() -> ()  [unwired: 1 in, 6 out]
        n305 = Build Array("405nm", "488nm", "561nm") -> (→"Laser":bool[])
      }
      event "488nm": Value Change {
        n306 = event-data() -> ()  [unwired: 1 in, 6 out]
        n307 = local read "561nm"() -> (w438:bool)
        n308 = local read "488nm"() -> (w439:bool)
        n309 = local read "405nm"() -> (w440:bool)
        n310 = Build Array(w440, w439, w438) -> (w437:bool[])
        n311 = local write "Laser"(w437) -> ()
      }
      event "561nm": Value Change {
        n312 = event-data() -> ()  [unwired: 1 in, 6 out]
        n313 = local read "405nm"() -> (w444:bool)
        n314 = local read "488nm"() -> (w443:bool)
        n315 = local read "561nm"() -> (w442:bool)
        n316 = Build Array(w444, w443, w442) -> (w441:bool[])
        n317 = local write "Laser"(w441) -> ()
      }
    }
  }
  n318 = while {
    tunnel: w1 -> [w445]
    stop <- FALSE stop-if-true
    n319 = stacked-sequence {
      tunnel: w445 -> [w447]
      frame #0 {
        n320 = event shown="[1] \"ZeroZ\": Mouse Down" {
          selector: _ -> [_ _ _ _]
          dyn-events: _ -> [_ _ _ _]
          timeout: _ -> [_ _ _ _]
          tunnel: w447 -> [w450 _ w494 w520]
          event "GoZ": Mouse Down {
            n321 = event-data() -> ()  [unwired: 1 in, 8 out]
            n322 = local read "Relative MoveZ"() -> (w451:string)
            n323 = flat-sequence {
              tunnel: w450 -> [w465]
              tunnel: [w465] -> w453
              tunnel: w451 -> [w464]
              tunnel: [w454] -> w448
              tunnel: w453 -> [w472]
              tunnel: [w472] -> w452
              tunnel: [w470] -> w449
              tunnel: w448 -> [w470]
              tunnel: w452 -> [w479]
              tunnel: w449 -> [w473]
              frame #0 {
                w457 = i16 100 ("width (-)")
                n324 = Decimal String To Number(string=w464) -> (number=w455:i32)  [unwired: 2 in, 1 out]
                n325 = Absolute Value(x=w455) -> (abs(x)=w460:i32)
                n326 = Sign(1:w455) -> (0:w456:i32)
                n327 = Multiply(x=w457, y=w456) -> (x*y=w458:i32)
                n328 = Greater?(x=w460, y=w457) -> (0:w459:bool)
                n329 = Select(t=w458, s=w459, f=w455) -> (s? t:f=w454:i32)
                n330 = Number To Hexadecimal String(1:i16 8 ("width (-)"), 2:w454) -> (0:w461:string)
                n331 = Concatenate Strings("AA0100010000000000000000" ("write buffer"), w461, "00000000" ("write buffer")) -> (w466:string)
                n332 = call "CRC-MODBUS.vi"("数据"=w466) -> ("数据+CRC"=w463:string)
                n333 = call "Character-H16.vi"("string"=w463) -> ("string 2"=w462:string)
                n334 = VISA Write(VISA resource name=w465, write buffer=w462) -> ()  [unwired: 1 in, 3 out]
              }
              frame #1 {
                n335 = Wait (ms)(milliseconds to wait=u32 150) -> ()  [unwired: 1 out]
              }
              frame #2 {
                n336 = local read "Current PositionZ:"() -> (w475:string)
                n337 = Decimal String To Number(string=w475) -> (number=w476:i32)  [unwired: 2 in, 1 out]
                n338 = Add(x=w476, y=w473) -> (x+y=w477:i32)
                n339 = Number To Decimal String(number=w477) -> (decimal integer string=w474:string)  [unwired: 1 in]
                n340 = local write "Current PositionZ:"(w474) -> ()
                n341 = VISA Write(VISA resource name=w479, write buffer="ª\u0001\u0000\u0002\u0000\u0000\u0000\u0000\u0000\u0000\u0000\u0000\u0000\u0000\u0000\u0001\u0000\u0000\u0000\u0000…U") -> ()  [unwired: 1 in, 3 out]
              }
            }
          }
          event "ZeroZ": Mouse Down {
            n342 = event-data() -> ()  [unwired: 1 in, 8 out]
            n343 = flat-sequence {
              frame #0 {
                n344 = local read "Current PositionZ:"() -> (w484:string)
                n345 = property on="Multicolumn Listbox" class="MCListbox (strict)"() -> ("ItemNames"=w482:string[][])  [unwired: 2 in, 2 out]
                n346 = Decimal String To Number(string=w484) -> (number=w483:i32)  [unwired: 2 in, 1 out]
                n347 = Index Array(array=w482, index (col)=3 ("index")) -> (element=w486:string[])  [unwired: 1 in]
                n348 = Decimal String To Number(string=w486) -> (number=w487:i32[])  [unwired: 2 in, 1 out]
                n349 = Subtract(x=w487, y=w483) -> (x-y=w488:i32[])
                n350 = Number To Decimal String(number=w488) -> (decimal integer string=w489:string[])  [unwired: 1 in]
                n351 = Replace Array Subset(array=w482, new element=w489, index (col)=3 ("index")) -> (w480:string[][])  [unwired: 1 in]
                n352 = property on="Multicolumn Listbox" class="MCListbox (strict)"("ItemNames"=w480) -> ()  [unwired: 2 in, 2 out]
              }
              frame #1 {
                n353 = local write "Current PositionZ:"("0") -> ()
              }
            }
          }
          event "homeZ": Mouse Down {
            n354 = event-data() -> ()  [unwired: 1 in, 8 out]
            n355 = local read "Current PositionZ:"() -> (w493:string)
            n356 = flat-sequence {
              tunnel: w494 -> [w502]
              tunnel: [w502] -> w496
              tunnel: w493 -> [w499]
              tunnel: [w497] -> w491
              tunnel: w496 -> [w510]
              tunnel: [w510] -> w495
              tunnel: [w508] -> w492
              tunnel: w491 -> [w508]
              tunnel: w495 -> [w517]
              tunnel: w492 -> [w511]
              frame #0 {
                n357 = Decimal String To Number(string=w499) -> (number=w498:i32)  [unwired: 2 in, 1 out]
                n358 = Negate(x=w498) -> (-x=w497:i32)
                n359 = Number To Hexadecimal String(1:i16 8 ("width (-)"), 2:w497) -> (0:w505:string)
                n360 = Concatenate Strings("AA0100010000000000000000" ("write buffer"), w505, "00000000" ("write buffer")) -> (w503:string)
                n361 = call "CRC-MODBUS.vi"("数据"=w503) -> ("数据+CRC"=w501:string)
                n362 = call "Character-H16.vi"("string"=w501) -> ("string 2"=w500:string)
                n363 = VISA Write(VISA resource name=w502, write buffer=w500) -> ()  [unwired: 1 in, 3 out]
              }
              frame #1 {
                n364 = Wait (ms)(milliseconds to wait=u32 100) -> ()  [unwired: 1 out]
              }
              frame #2 {
                n365 = local read "Current PositionZ:"() -> (w513:string)
                n366 = Decimal String To Number(string=w513) -> (number=w515:i32)  [unwired: 2 in, 1 out]
                n367 = Add(x=w515, y=w511) -> (x+y=w514:i32)
                n368 = Number To Decimal String(number=w514) -> (decimal integer string=w512:string)  [unwired: 1 in]
                n369 = local write "Current PositionZ:"(w512) -> ()
                n370 = VISA Write(VISA resource name=w517, write buffer="ª\u0001\u0000\u0002\u0000\u0000\u0000\u0000\u0000\u0000\u0000\u0000\u0000\u0000\u0000\u0001\u0000\u0000\u0000\u0000…U") -> ()  [unwired: 1 in, 3 out]
              }
            }
          }
          event "GoZ 2": Mouse Down {
            n371 = event-data() -> ()  [unwired: 1 in, 8 out]
            n372 = local read "Relative MoveZ"() -> (w521:string)
            n373 = flat-sequence {
              tunnel: w520 -> [w535]
              tunnel: [w535] -> w523
              tunnel: w521 -> [w534]
              tunnel: [w524] -> w518
              tunnel: w523 -> [w543]
              tunnel: [w543] -> w522
              tunnel: [w541] -> w519
              tunnel: w518 -> [w541]
              tunnel: w522 -> [w550]
              tunnel: w519 -> [w544]
              frame #0 {
                w528 = i16 100 ("width (-)")
                n374 = Decimal String To Number(string=w534) -> (number=w526:i32)  [unwired: 2 in, 1 out]
                n375 = Absolute Value(x=w526) -> (abs(x)=w531:i32)
                n376 = Sign(1:w526) -> (0:w527:i32)
                n377 = Multiply(x=w528, y=w527) -> (x*y=w529:i32)
                n378 = Greater?(x=w531, y=w528) -> (0:w530:bool)
                n379 = Select(t=w529, s=w530, f=w526) -> (s? t:f=w525:i32)
                n380 = Negate(x=w525) -> (-x=w524:i32)
                n381 = Number To Hexadecimal String(1:i16 8 ("width (-)"), 2:w524) -> (0:w538:string)
                n382 = Concatenate Strings("AA0100010000000000000000" ("write buffer"), w538, "00000000" ("write buffer")) -> (w536:string)
                n383 = call "CRC-MODBUS.vi"("数据"=w536) -> ("数据+CRC"=w533:string)
                n384 = call "Character-H16.vi"("string"=w533) -> ("string 2"=w532:string)
                n385 = VISA Write(VISA resource name=w535, write buffer=w532) -> ()  [unwired: 1 in, 3 out]
              }
              frame #1 {
                n386 = Wait (ms)(milliseconds to wait=u32 100) -> ()  [unwired: 1 out]
              }
              frame #2 {
                n387 = local read "Current PositionZ:"() -> (w546:string)
                n388 = Decimal String To Number(string=w546) -> (number=w547:i32)  [unwired: 2 in, 1 out]
                n389 = Add(x=w547, y=w544) -> (x+y=w548:i32)
                n390 = Number To Decimal String(number=w548) -> (decimal integer string=w545:string)  [unwired: 1 in]
                n391 = VISA Write(VISA resource name=w550, write buffer="ª\u0001\u0000\u0002\u0000\u0000\u0000\u0000\u0000\u0000\u0000\u0000\u0000\u0000\u0000\u0001\u0000\u0000\u0000\u0000…U") -> ()  [unwired: 1 in, 3 out]
                n392 = local write "Current PositionZ:"(w545) -> ()
              }
            }
          }
        }
      }
    }
  }
  n393 = local read "488nm"() -> (w11:bool)
  n394 = local read "405nm"() -> (w10:bool)
  n395 = local read "561nm"() -> (w9:bool)
  n396 = Build Array(w10, w11, w9) -> (w8:bool[])
  n397 = flat-sequence {
    tunnel: [w551] -> w29
    tunnel: w13 -> [w551]
    tunnel: w29 -> [w556]
    tunnel: [w557] -> w28
    tunnel: w12 -> [w555]
    tunnel: w1 -> [w554]
    tunnel: w1 -> [w553]
    tunnel: w28 -> [w1890]
    frame #0 {
      # "library"
    }
    frame #1 {
      # "Library"
      # "camera SR"
      # "Buffer Index SR"
      # "camera status SR"
      # "histogram SR"
      n398 = while {
        shift-right: [w570] -> _
        shift-left: _ -> [w571]
        tunnel: w556 -> [w572]
        tunnel: [w573] -> w557
        shift-right: [w569] -> _
        shift-left: _ -> [w568]
        shift-right: [w566] -> _
        shift-left: _ -> [w567]
        shift-right: [w564] -> _
        shift-left: _ -> [w565]
        tunnel: w555 -> [w563]
        tunnel: w554 -> [w562]
        tunnel: w553 -> [w561]
        shift-right: [w559] -> _
        shift-left: 0 -> [w560]
        stop <- FALSE stop-if-true
        n399 = event shown="[16] \"Live start\": Value Change" {
          selector: _ -> [_ _ _ _ _ _ _ _ _ _ _ _ _ _ _ _ _ _ _]
          dyn-events: _ -> [_ _ _ _ _ _ _ _ _ _ _ _ _ _ _ _ _ _ _]
          timeout: _ -> [_ _ _ _ _ _ _ _ _ _ _ _ _ _ _ _ _ _ _]
          tunnel: [w578 w585 w616 _ _ _ _ w1320 _ _ _ _ _ _ _ _ _ _ _] -> w573
          tunnel: w572 -> [w578 w584 w615 _ _ _ _ w1322 _ _ _ _ _ _ _ _ _ _ _]
          tunnel: [_ _ w617 _ _ _ _ _ _ _ _ _ _ _ _ _ _ _ _] -> _
          tunnel: w571 -> [w577 w582 w614 w671 w708 w790 w1310 w1321 w1424 w1528 w1566 w1615 w1644 w1670 w1693 w1773 w1818 w1849 w1874]
          tunnel: [w577 w582 w614 w674 w711 w788 w1310 w1319 w1425 w1527 w1568 w1614 w1643 w1669 w1689 w1772 w1817 w1848 w1873] -> w570
          tunnel: [w576 w581 w612 w670 w707 w793 w1311 w1318 w1422 w1526 w1565 w1613 w1641 w1668 w1691 w1770 w1816 w1847 w1877] -> w569
          tunnel: w568 -> [w576 w581 w612 w670 w707 w793 w1311 w1317 w1423 w1526 w1565 w1613 w1641 w1668 w1691 w1770 w1816 w1847 w1877]
          tunnel: [w575 w579 w613 w673 w710 w792 w1309 w1313 w1418 w1525 w1564 w1612 w1640 w1667 w1690 w1769 w1815 w1846 w1876] -> w566
          tunnel: w567 -> [w575 w579 w613 w673 w710 w792 w1309 w1316 w1421 w1525 w1564 w1612 w1640 w1667 w1690 w1769 w1815 w1846 w1876]
          tunnel: w565 -> [w574 w580 w611 w672 w709 w791 w1308 w1315 w1420 w1524 w1563 w1611 w1642 w1666 w1688 w1768 w1814 w1845 w1875]
          tunnel: [w574 w580 w611 w672 w709 w791 w1308 w1314 w1419 w1524 w1563 w1611 w1642 w1666 w1688 w1768 w1814 w1845 w1875] -> w564
          tunnel: w563 -> [_ _ _ _ w706 w789 _ _ _ _ _ _ _ _ _ _ _ _ _]
          tunnel: w562 -> [_ _ _ _ _ w787 _ _ _ _ _ _ _ _ _ _ _ _ _]
          tunnel: w561 -> [_ _ _ _ _ _ _ _ _ _ _ _ _ _ _ _ _ _ _]
          tunnel: w560 -> [_ _ _ _ _ w786 _ _ _ _ _ _ _ _ _ _ _ _ _]
          tunnel: [_ _ _ _ _ w785 _ _ _ _ _ _ _ _ _ _ _ _ _] -> w559
          event Timeout {
            n400 = event-data() -> ()  [unwired: 1 in, 3 out]
          }
          event "Init": Value Change {
            n401 = event-data() -> ()  [unwired: 1 in, 6 out]
            n402 = case shown="True" "Init" {
              tunnel: [w586 w589] -> w585
              tunnel: w584 -> [w586 w590]
              frame False {
              }
              frame True {
                n403 = local read "PVCam indicator"() -> (w588:bool)
                n404 = Not(x=w588) -> (.not. x?=w587:bool)
                n405 = case shown="True" w587 {
                  tunnel: w590 -> [w592 w594]
                  tunnel: [w592 w593] -> w589
                  frame False {
                    n406 = One Button Dialog(message="PVCam is initialized") -> ()  [unwired: 1 in, 1 out]
                  }
                  frame True {
                    n407 = flat-sequence {
                      tunnel: w594 -> [w604]
                      tunnel: [w597] -> w595
                      tunnel: [w610] -> w593
                      tunnel: w595 -> [w610]
                      frame #0 {
                        n408 = property class="Library"(reference=w604) -> (reference out=w597:refnum<k24>, "PVCamVersion"=w603:string, "Cameras"=w602:refnum<k24>, "Version"=w596:string)  [unwired: 1 in, 1 out]
                        n409 = local write "PVCamNET version"(w596) -> ()
                        n410 = property class="PmReadOnlyObservableCollection`"(reference=w602) -> (reference out=w600:refnum<k24>, "Count"=w601:i32)  [unwired: 1 in, 1 out]
                        n411 = local write "PVCam version"(w603) -> ()
                        n412 = for {
                          N: w601 -> [_]
                          tunnel: w600 -> [w608]
                          tunnel: [w605] -> w598 mode=indexing
                          i -> [w607]
                          n413 = invoke class="PmReadOnlyObservableCollection`" method="get_Item"(reference=w608, "index"=w607) -> ("get_Item"=w606:refnum<k24>)  [unwired: 2 in, 3 out]
                          n414 = property class="Camera"(reference=w606) -> ("Name"=w605:string)  [unwired: 1 in, 2 out]
                        }
                        n415 = control-ref of="Select Camera"() -> (w599:refnum<vi>)
                        n416 = property class="CmbBox"(reference=w599, "Strings[]"=w598) -> ()  [unwired: 1 in, 2 out]
                      }
                      frame #1 {
                        n417 = local write "PVCam indicator"(TRUE ("PVCam status")) -> ()
                      }
                    }
                  }
                }
              }
            }
          }
          event "Uninit": Value Change {
            n418 = event-data() -> ()  [unwired: 1 in, 6 out]
            n419 = case shown="True" "Uninit" {
              tunnel: [FALSE ("PVCam status") w624] -> w617
              tunnel: [w619 w623] -> w616
              tunnel: w615 -> [w619 w622]
              frame False {
              }
              frame True {
                n420 = local read "PVCam indicator"() -> (w621:bool)
                n421 = case shown="True" w621 {
                  tunnel: [FALSE ("PVCam status") w630] -> w624
                  tunnel: [w627 w628] -> w623
                  tunnel: w622 -> [w627 w629]
                  frame False {
                    n422 = One Button Dialog(message="PVCam is not initialized") -> ()  [unwired: 1 in, 1 out]
                  }
                  frame True {
                    n423 = flat-sequence {
                      tunnel: [w661] -> w628
                      tunnel: w629 -> [w661]
                      tunnel: [TRUE ("PVCam status")] -> w630
                      frame #0 {
                        w651 = u32 1 ("Y Binning")
                        w650 = 0.0 ("Clear Cycle")
                        w649 = FALSE ("Camera Status")
                        w648 = 0 ("Full CCD Y")
                        n424 = control-ref of="Select Camera"() -> (w665:refnum<vi>)
                        n425 = control-ref of="Sensor clearing mode"() -> (w659:refnum<vi>)
                        n426 = control-ref of="Readout ports and speed"() -> (w642:refnum<vi>)
                        n427 = control-ref of="8 Bit Histogram"() -> (w635:refnum<vi>)
                        n428 = local write "PVCam indicator"(FALSE ("PVCam status")) -> ()
                        n429 = local write "PVCam version"("" ("PVCam version")) -> ()
                        n430 = local write "Y Binning"(w651) -> ()
                        n431 = local write "X Binning"(w651) -> ()
                        n432 = property class="CmbBox"(reference=w665, "Value"="", "Strings[]"=string[] [] ("Strings []")) -> ()  [unwired: 1 in, 2 out]
                        n433 = local write "Height"(w648) -> ()
                        n434 = local write "Width"(w648) -> ()
                        n435 = local write "X"(w648) -> ()
                        n436 = local write "Y"(w648) -> ()
                        n437 = property class="CmbBox"(reference=w642, "Value"="", "Strings[]"=string[] [] ("Strings []")) -> ()  [unwired: 1 in, 2 out]
                        n438 = property class="CmbBox"(reference=w659, "Strings[]"=string[] [] ("Strings []"), "Value"="") -> ()  [unwired: 1 in, 2 out]
                        n439 = local write "Full CCD Height"(w648) -> ()
                        n440 = local write "Full CCD Width"(w648) -> ()
                        n441 = local write "Full CCD X"(w648) -> ()
                        n442 = local write "Full CCD Y"(w648) -> ()
                        n443 = property class="WFGraph (strict)"(reference=w635, "Value"=i32[] []) -> ()  [unwired: 1 in, 2 out]
                        n444 = local write "Live status"(FALSE ("Live")) -> ()
                        n445 = local write "LabVIEW app version"("" ("LabVIEW app version")) -> ()
                        n446 = local write "PVCamNET version"("" ("PVCamNET version")) -> ()
                        n447 = control-ref of="Trigger Out Behaviour"() -> (w660:refnum<vi>)
                        n448 = control-ref of="Gain"() -> (w641:refnum<vi>)
                        n449 = control-ref of="Trigger In Behaviour"() -> (w640:refnum<vi>)
                        n450 = local write item#7("" ("PVCam version")) -> ()
                        n451 = control-ref of="Binning"() -> (w658:refnum<vi>)
                        n452 = property class="CmbBox"(reference=w641, "Value"="", "Strings[]"=string[] [] ("Strings []")) -> ()  [unwired: 1 in, 2 out]
                        n453 = property class="CmbBox"(reference=w640, "Value"="", "Strings[]"=string[] [] ("Strings []")) -> ()  [unwired: 1 in, 2 out]
                        n454 = control-ref of="Exposure Resolution"() -> (w631:refnum<vi>)
                        n455 = property class="CmbBox"(reference=w660, "Strings[]"=string[] [] ("Strings []"), "Value"="") -> ()  [unwired: 1 in, 2 out]
                        n456 = local write "PVCam indicator"(w649) -> ()
                        n457 = local write "Clear Cycles"(w650) -> ()
                        n458 = local write "Exposure Time"(w650) -> ()
                        n459 = local write "Camera status"(w649) -> ()
                        n460 = property class="CmbBox"(reference=w658, "Strings[]"=string[] [] ("Strings []"), "Value"="") -> ()  [unwired: 1 in, 2 out]
                        n461 = property class="CmbBox"(reference=w631, "Value"="", "Strings[]"=string[] [] ("Strings []")) -> ()  [unwired: 1 in, 2 out]
                      }
                      frame #1 {
                        n462 = One Button Dialog(message="PVCam closed") -> ()  [unwired: 1 in, 1 out]
                      }
                    }
                  }
                }
              }
            }
          }
          event "Single Capture": Value Change {
            n463 = event-data() -> ()  [unwired: 1 in, 6 out]
            n464 = case shown="True" "Single Capture" {
              tunnel: w671 -> [w676 w678]
              tunnel: [w676 w679] -> w674
              frame False {
              }
              frame True {
                n465 = local read "Camera status"() -> (w677:bool)
                n466 = case shown="True" w677 {
                  tunnel: [w681 w691] -> w679
                  tunnel: w678 -> [w681 w690]
                  frame False {
                    n467 = One Button Dialog(message="Camera is not open") -> ()  [unwired: 1 in, 1 out]
                  }
                  frame True {
                    w688 = 0 items=["Idle", "Capturing"] ("Status")
                    n468 = property class="Camera"(reference=w690) -> (reference out=w682:refnum<k24>, "IsOpen"=w687:bool, "Status"=w689:i32)  [unwired: 1 in, 1 out]
                    n469 = Equal?(x=w687, y=TRUE) -> (x = y?=w685:bool)
                    n470 = Equal?(x=w689, y=w688) -> (x = y?=w684:bool)
                    n471 = Equal?(x=w685, y=w684) -> (x = y?=w683:bool)
                    n472 = case shown="True" w683 {
                      tunnel: [w692 w698] -> w691
                      tunnel: w682 -> [w692 w704]
                      frame False {
                      }
                      frame True {
                        n473 = control-ref of="Exposure Time"() -> (w694:refnum<vi>)
                        n474 = property class="DigNum (strict)"(reference=w694) -> ("Value"=w693:dbl)  [unwired: 1 in, 2 out]
                        n475 = property class="Camera"(reference=w704) -> (reference out=w699:refnum<k24>, "Settings"=w696:refnum<k24>)  [unwired: 1 in, 1 out]
                        n476 = property class="CameraSettings"(reference=w696, "Exposure"=w693) -> (reference out=w695:refnum<k24>)  [unwired: 1 in, 1 out]
                        n477 = property class="CameraSettings"(reference=w695, "FramesToCapture"=u16 1) -> (error out=w697:errorcluster, "XBinning"=→"XBinning":u16, "YBinning"=→"YBinning":u16, "Exposure"=→"Exposure":u32)  [unwired: 1 in, 1 out]
                        n478 = invoke class="Camera" method="StartSequence"(reference=w699, error in=w697) -> (reference out=w698:refnum<k24>)  [unwired: 1 in, 2 out]
                      }
                    }
                  }
                }
              }
            }
          }
          event "Single Capture SLM": Value Change {
            n479 = event-data() -> ()  [unwired: 1 in, 6 out]
            n480 = for {
              N: "Numeric 2" -> [_]
              tunnel: [w716] -> w711
              tunnel: w708 -> [w715]
              tunnel: w706 -> [w714]
              i -> [w713]
              n481 = Wait (ms)(milliseconds to wait=u32 500) -> ()  [unwired: 1 out]
              n482 = stacked-sequence {
                tunnel: [_ w727 _ _] -> w716
                tunnel: w715 -> [_ w726 w757 _]
                tunnel: w714 -> [w718 _ _ w777]
                frame #0 {
                  n483 = local read "Laser Channel"() -> (w717:u16)
                  n484 = Increment(x=w717) -> (x+1=w723:u16)
                  n485 = Number To Decimal String(number=w723) -> (decimal integer string=w722:string)  [unwired: 1 in]
                  n486 = Concatenate Strings("L" ("write buffer"), w722, "O1E" ("write buffer"), "\r") -> (w724:string)
                  n487 = VISA Write(VISA resource name=w718, write buffer=w724) -> ()  [unwired: 1 in, 3 out]
                }
                frame #1 {
                  n488 = case shown="True" "Single Capture SLM" {
                    tunnel: w726 -> [w728 w730]
                    tunnel: [w728 w731] -> w727
                    frame False {
                    }
                    frame True {
                      n489 = local read "Camera status"() -> (w729:bool)
                      n490 = case shown="True" w729 {
                        tunnel: [w733 w743] -> w731
                        tunnel: w730 -> [w733 w742]
                        frame False {
                          n491 = One Button Dialog(message="Camera is not open") -> ()  [unwired: 1 in, 1 out]
                        }
                        frame True {
                          w740 = 0 items=["Idle", "Capturing"] ("Status")
                          n492 = property class="Camera"(reference=w742) -> (reference out=w734:refnum<k24>, "IsOpen"=w739:bool, "Status"=w741:i32)  [unwired: 1 in, 1 out]
                          n493 = Equal?(x=w739, y=TRUE) -> (x = y?=w737:bool)
                          n494 = Equal?(x=w741, y=w740) -> (x = y?=w736:bool)
                          n495 = Equal?(x=w737, y=w736) -> (x = y?=w735:bool)
                          n496 = case shown="True" w735 {
                            tunnel: [w744 w750] -> w743
                            tunnel: w734 -> [w744 w756]
                            frame False {
                            }
                            frame True {
                              n497 = control-ref of="Exposure Time"() -> (w746:refnum<vi>)
                              n498 = property class="DigNum (strict)"(reference=w746) -> ("Value"=w745:dbl)  [unwired: 1 in, 2 out]
                              n499 = property class="Camera"(reference=w756) -> (reference out=w751:refnum<k24>, "Settings"=w748:refnum<k24>)  [unwired: 1 in, 1 out]
                              n500 = property class="CameraSettings"(reference=w748, "Exposure"=w745) -> (reference out=w747:refnum<k24>)  [unwired: 1 in, 1 out]
                              n501 = property class="CameraSettings"(reference=w747, "FramesToCapture"=u16 1) -> (error out=w749:errorcluster, "XBinning"=→"XBinning 3":u16, "YBinning"=→"YBinning 3":u16, "Exposure"=→"Exposure 2":u32)  [unwired: 1 in, 1 out]
                              n502 = invoke class="Camera" method="StartSequence"(reference=w751, error in=w749) -> (reference out=w750:refnum<k24>)  [unwired: 1 in, 2 out]
                            }
                          }
                        }
                      }
                    }
                  }
                }
                frame #2 {
                  n503 = while {
                    tunnel: [w764] -> w763
                    tunnel: [w769] -> w761
                    tunnel: w757 -> [w768]
                    tunnel: [w767] -> w758
                    stop <- w764 stop-if-true
                    w765 = 0 items=["Idle", "Capturing"] ("Status")
                    n504 = property class="Camera"(reference=w768) -> (reference out=w767:refnum<k24>, "IsOpen"=w769:bool, "Status"=w766:i32)  [unwired: 1 in, 1 out]
                    n505 = Equal?(x=w766, y=w765) -> (x = y?=w764:bool)
                  }
                  n506 = Equal?(x=w761, y=TRUE) -> (x = y?=w762:bool)
                  n507 = Equal?(x=w762, y=w763) -> (x = y?=w759:bool)
                  n508 = case shown="True" w759 {
                    tunnel: w758 -> [w771 w776]
                    tunnel: [w771 w774] -> _
                    frame False {
                      n509 = One Button Dialog(message="Camera must be idle") -> ()  [unwired: 1 in, 1 out]
                    }
                    frame True {
                      (unwired) TRUE ("Boolean 3")
                      n510 = property class="Camera"(reference=w776) -> (reference out=w774:refnum<k24>, "AcquisitionBuffer"=w775:refnum<k24>)  [unwired: 1 in, 1 out]
                      n511 = property class="AcqBuffer"(reference=w775) -> (reference out=w773:refnum<k24>, "BufferIndex"=w772:i32)  [unwired: 1 in, 1 out]
                      n512 = invoke class="AcqBuffer" method="SaveAsTiff"(reference=w773, "nth"=w772) -> ()  [unwired: 2 in, 4 out]
                    }
                  }
                }
                frame #3 {
                  n513 = local read "Laser Channel"() -> (w778:u16)
                  n514 = Increment(x=w778) -> (x+1=w783:u16)
                  n515 = Number To Decimal String(number=w783) -> (decimal integer string=w782:string)  [unwired: 1 in]
                  n516 = Concatenate Strings("L" ("write buffer"), w782, "O0E" ("write buffer"), "\r") -> (w784:string)
                  n517 = VISA Write(VISA resource name=w777, write buffer=w784) -> ()  [unwired: 1 in, 3 out]
                }
              }
              "Numeric" <- w713
            }
          }
          event "AutoImaging": Mouse Down {
            n518 = event-data() -> ()  [unwired: 1 in, 8 out]
            n519 = flat-sequence {
              tunnel: w790 -> [w800]
              tunnel: w789 -> [w799]
              tunnel: [w798] -> w788
              tunnel: w787 -> [w797]
              tunnel: w786 -> [w796]
              tunnel: [w795] -> w785
              frame #0 {
                n520 = while {
                  tunnel: w800 -> [w822]
                  tunnel: w799 -> [w821]
                  tunnel: [w820] -> w798
                  tunnel: w797 -> [w815]
                  shift-right: [w818] -> w795
                  shift-left: w796 -> [w819]
                  shift-right: [w805] -> _
                  shift-left: 0 -> [w806]
                  i -> [w807]
                  stop <- w801 continue-if-true
                  n521 = flat-sequence {
                    tunnel: w821 -> [w830]
                    tunnel: w822 -> [w831]
                    tunnel: [w831] -> w817
                    tunnel: [w830] -> w816
                    tunnel: w815 -> [w828]
                    tunnel: w806 -> [w827]
                    tunnel: [w938] -> w826
                    tunnel: [w924] -> w825
                    tunnel: [w931] -> w824
                    tunnel: [w913] -> w823
                    tunnel: w817 -> [w938]
                    tunnel: w816 -> [w924]
                    tunnel: w805 -> [w920]
                    tunnel: [w980] -> w820
                    tunnel: w826 -> [w982]
                    tunnel: w825 -> [w981]
                    tunnel: w824 -> [w979]
                    tunnel: w823 -> [w978]
                    tunnel: w818 -> [_]
                    tunnel: w818 -> [w977]
                    tunnel: w815 -> [w976]
                    frame #0 {
                      n522 = local read "Batch"() -> (w829:enum32{"Single", "Batch"})
                      n523 = case shown="\"Single\", Default" w829 {
                        tunnel: w828 -> [_ w833]
                        tunnel: w827 -> [_ w832]
                        frame "Single", Default {
                        }
                        frame "Batch" {
                          n524 = property on="Multicolumn Listbox" class="MCListbox (strict)"() -> ("ItemNames"=w834:string[][])  [unwired: 2 in, 2 out]
                          n525 = Index Array(array=w834, index (row)=w832) -> (element=w838:string[])  [unwired: 1 in]
                          n526 = Index Array(array=w838, index #1=i16 1 ("width (-)"), index #2=i16 2 ("width (-)"), index #3=i16 3 ("width (-)")) -> (element #1=w841:string, element #2=w840:string, element #3=w839:string)
                          n527 = flat-sequence {
                            tunnel: w833 -> [w850]
                            tunnel: [w850] -> w849
                            tunnel: [w851] -> w848
                            tunnel: w839 -> [w873]
                            tunnel: w840 -> [w861]
                            tunnel: w841 -> [w860]
                            tunnel: [w852] -> w847
                            tunnel: [w853] -> w846
                            tunnel: w849 -> [w884]
                            tunnel: [w884] -> w845
                            tunnel: [w882] -> w844
                            tunnel: w848 -> [w882]
                            tunnel: [w881] -> w843
                            tunnel: w847 -> [w881]
                            tunnel: [w880] -> w842
                            tunnel: w846 -> [w880]
                            tunnel: w845 -> [w901]
                            tunnel: w844 -> [w895]
                            tunnel: w843 -> [w890]
                            tunnel: w842 -> [w889]
                            frame #0 {
                              n528 = local read "Current PositionZ:"() -> (w871:string)
                              n529 = local read "Current PositionY"() -> (w854:string)
                              n530 = local read "Current PositionX"() -> (w855:string)
                              n531 = Decimal String To Number(string=w873) -> (number=w869:i32)  [unwired: 2 in, 1 out]
                              n532 = Decimal String To Number(string=w871) -> (number=w870:i32)  [unwired: 2 in, 1 out]
                              n533 = Decimal String To Number(string=w861) -> (number=w865:i32)  [unwired: 2 in, 1 out]
                              n534 = Decimal String To Number(string=w860) -> (number=w862:i32)  [unwired: 2 in, 1 out]
                              n535 = Subtract(x=w870, y=w869) -> (x-y=w868:i32)
                              n536 = Decimal String To Number(string=w854) -> (number=w866:i32)  [unwired: 2 in, 1 out]
                              n537 = Decimal String To Number(string=w855) -> (number=w863:i32)  [unwired: 2 in, 1 out]
                              n538 = Negate(x=w868) -> (-x=w851:i32)
                              n539 = Subtract(x=w863, y=w862) -> (x-y=w856:i32)
                              n540 = Subtract(x=w866, y=w865) -> (x-y=w857:i32)
                              n541 = Negate(x=w856) -> (-x=w853:i32)
                              n542 = Negate(x=w857) -> (-x=w852:i32)
                              n543 = Number To Hexadecimal String(1:i16 8 ("width (-)"), 2:w851) -> (0:w874:string)
                              n544 = Number To Hexadecimal String(1:i16 8 ("width (-)"), 2:w852) -> (0:w859:string)
                              n545 = Number To Hexadecimal String(1:i16 8 ("width (-)"), 2:w853) -> (0:w858:string)
                              n546 = Concatenate Strings("AA010001" ("write buffer"), w858, w859, w874, "00000000" ("write buffer")) -> (w877:string)
                              n547 = call "CRC-MODBUS.vi"("数据"=w877) -> ("数据+CRC"=w876:string)
                              n548 = call "Character-H16.vi"("string"=w876) -> ("string 2"=w875:string)
                              n549 = VISA Write(VISA resource name=w850, write buffer=w875) -> ()  [unwired: 1 in, 3 out]
                            }
                            frame #1 {
                              n550 = Wait (ms)(milliseconds to wait=u32 100) -> ()  [unwired: 1 out]
                            }
                            frame #2 {
                              n551 = local read "Current PositionX"() -> (w886:string)
                              n552 = local read "Current PositionY"() -> (w887:string)
                              n553 = local read "Current PositionZ:"() -> (w897:string)
                              n554 = Decimal String To Number(string=w886) -> (number=w891:i32)  [unwired: 2 in, 1 out]
                              n555 = Decimal String To Number(string=w887) -> (number=w893:i32)  [unwired: 2 in, 1 out]
                              n556 = Decimal String To Number(string=w897) -> (number=w898:i32)  [unwired: 2 in, 1 out]
                              n557 = Add(x=w891, y=w889) -> (x+y=w892:i32)
                              n558 = Add(x=w893, y=w890) -> (x+y=w894:i32)
                              n559 = Add(x=w898, y=w895) -> (x+y=w899:i32)
                              n560 = Number To Decimal String(number=w892) -> (decimal integer string=w885:string)  [unwired: 1 in]
                              n561 = local write "Current PositionX"(w885) -> ()
                              n562 = Number To Decimal String(number=w894) -> (decimal integer string=w888:string)  [unwired: 1 in]
                              n563 = local write "Current PositionY"(w888) -> ()
                              n564 = Number To Decimal String(number=w899) -> (decimal integer string=w896:string)  [unwired: 1 in]
                              n565 = local write "Current PositionZ:"(w896) -> ()
                              n566 = VISA Write(VISA resource name=w901, write buffer="ª\u0001\u0000\u0002\u0000\u0000\u0000\u0001\u0000\u0000\u0000\u0001\u0000\u0000\u0000\u0001\u0000\u0000\u0000\u0000ŠD") -> ()  [unwired: 1 in, 3 out]
                            }
                            frame #3 {
                              n567 = Wait (ms)(milliseconds to wait=u32 5000) -> ()  [unwired: 1 out]
                            }
                          }
                        }
                      }
                    }
                    frame #1 {
                      w925 = path "C:/Users/Dell/Desktop/SIMImaging -电动平移台 -V4/Temp"
                      w931 = path "C:/Users/Dell/Desktop/SIMImaging -电动平移台 -V4"
                      w933 = ""
                      w932 = "\\"
                      # "其他图像文件移至temp"
                      n568 = call <vilib>:"Check if File or Folder Exists.vi"("path"=w925) -> ("file or folder exists?"=w928:bool)  [unwired: 8 in, 2 out]
                      n569 = Less?(x=w920, y=i16 10 ("width (-)")) -> (x < y?=w919:bool)
                      n570 = Number To Decimal String(number=w920, width (-)=i16 2) -> (decimal integer string=w917:string)
                      n571 = flat-sequence {
                        tunnel: w924 -> [w944]
                        frame #0 {
                          n572 = for {
                            N: 3 -> [_]
                            tunnel: w944 -> [w949]
                            i -> [w948]
                            w946 = FALSE ("L405nm")
                            n573 = Increment(x=w948) -> (x+1=w947:i32)
                            n574 = Number To Decimal String(number=w947) -> (decimal integer string=w953:string)  [unwired: 1 in]
                            n575 = Concatenate Strings("L" ("write buffer"), w953, "O0E" ("write buffer"), "\r") -> (w954:string)
                            n576 = VISA Write(VISA resource name=w949, write buffer=w954) -> ()  [unwired: 1 in, 3 out]
                            n577 = local write "L488nm"(w946) -> ()
                            n578 = local write "L561nm"(w946) -> ()
                            n579 = local write "L405nm"(w946) -> ()
                            n580 = Wait (ms)(milliseconds to wait=u32 200) -> ()  [unwired: 1 out]
                          }
                        }
                      }
                      n581 = List Folder(path=w931) -> (filenames=w927:string[])  [unwired: 3 in, 3 out]
                      n582 = Number To Decimal String(number=w920, width (-)=i16 1) -> (decimal integer string=w918:string)
                      n583 = case shown="False" w928 {
                        tunnel: w927 -> [w955 w957]
                        tunnel: [w955 w957] -> w926
                        tunnel: w925 -> [w956 _]
                        frame False {
                          n584 = Create Folder(path (use dialog)=w956) -> ()  [unwired: 2 in, 3 out]
                        }
                        frame True {
                        }
                      }
                      n585 = Select(t=w918, s=w919, f=w917) -> (s? t:f=w905:string)
                      n586 = case shown="\"Single\", Default" "Batch" {
                        tunnel: w905 -> [_ w941]
                        tunnel: ["" w940] -> w904
                        frame "Single", Default {
                        }
                        frame "Batch" {
                          n587 = Concatenate Strings("-", w941) -> (w940:string)
                        }
                      }
                      n588 = Array Size(array=w927) -> (size(s)=w937:i32)
                      n589 = Equal?(x="folder", y=w933) -> (x = y?=w934:bool)
                      n590 = for {
                        N: w937 -> [_]
                        tunnel: w926 -> [w968]
                        tunnel: w931 -> [w961]
                        i -> [w967]
                        n591 = Index Array(array=w968, index=w967) -> (element=w963:string)
                        n592 = Match Pattern(string=w963, regular expression=".tif") -> (offset past match=w964:i32)  [unwired: 1 in, 3 out]
                        n593 = Equal?(x=w964, y=-1) -> (x = y?=w962:bool)
                        n594 = case shown="False" w962 {
                          tunnel: w963 -> [w970 _]
                          tunnel: w961 -> [w969 _]
                          frame False {
                            n595 = Build Path(base path=w969, name or relative path=w970) -> (appended path=w975:path)
                            n596 = Path To String(path=w969) -> (string=w974:string)
                            n597 = Concatenate Strings(w974, "\\temp\\", w970) -> (w972:string)
                            n598 = String To Path(string=w972) -> (path=w971:path)
                            n599 = Move(source path=w975, 10:w971) -> ()  [unwired: 3 in, 3 out]
                          }
                          frame True {
                          }
                        }
                      }
                      n600 = Path To String(path=w931) -> (string=w936:string)
                      n601 = Select(t=w933, s=w934, f=w932) -> (s? t:f=w903:string)
                      n602 = Concatenate Strings(w936, w932, "folder", w904, w903) -> (w913:string)
                      n603 = String To Path(string=w913) -> (path=w930:path)
                      n604 = Concatenate Strings(w913, "c1\\") -> (w912:string)
                      n605 = Concatenate Strings(w913, "c2\\") -> (w911:string)
                      n606 = call <vilib>:"Check if File or Folder Exists.vi"("path"=w930) -> ("file or folder exists?"=w929:bool)  [unwired: 8 in, 2 out]
                      n607 = Concatenate Strings(w913, "c3\\") -> (w910:string)
                      n608 = String To Path(string=w912) -> (path=w909:path)
                      n609 = String To Path(string=w911) -> (path=w908:path)
                      n610 = String To Path(string=w910) -> (path=w907:path)
                      n611 = case shown="False" w929 {
                        tunnel: w909 -> [w960 _]
                        tunnel: w908 -> [w959 _]
                        tunnel: w907 -> [w958 _]
                        frame False {
                          n612 = Create Folder(path (use dialog)=w960) -> ()  [unwired: 2 in, 3 out]
                          n613 = Create Folder(path (use dialog)=w959) -> ()  [unwired: 2 in, 3 out]
                          n614 = Create Folder(path (use dialog)=w958) -> ()  [unwired: 2 in, 3 out]
                        }
                        frame True {
                        }
                      }
                    }
                    frame #2 {
                      n615 = while {
                        tunnel: w982 -> [w1000]
                        tunnel: w981 -> [w999]
                        tunnel: [w998] -> w980
                        tunnel: w979 -> [w997]
                        tunnel: w978 -> [w996]
                        tunnel: w977 -> [w993]
                        tunnel: w976 -> [w989]
                        i -> [w985]
                        stop <- w986 continue-if-true
                        n616 = local read "Z number"() -> (w984:i16)
                        n617 = flat-sequence {
                          tunnel: w1000 -> [w1002]
                          tunnel: w999 -> [w1007]
                          tunnel: w997 -> [w1005]
                          tunnel: w996 -> [w1004]
                          tunnel: w992 -> [w1003]
                          tunnel: [w1006] -> w991
                          tunnel: w991 -> [w1278]
                          tunnel: [w1278] -> w990
                          tunnel: w989 -> [w1275]
                          tunnel: [w1307] -> w998
                          tunnel: w990 -> [w1307]
                          frame #0 {
                            n618 = while {
                              tunnel: w1002 -> [w1021]
                              tunnel: w1007 -> [w1016]
                              tunnel: [w1020] -> w1006
                              tunnel: w1005 -> [w1019]
                              tunnel: w1004 -> [w1018]
                              tunnel: w1003 -> [w1017]
                              i -> [w1012]
                              stop <- w1009 continue-if-true
                              n619 = local read "Laser"() -> (w1015:bool[])
                              n620 = Index Array(array=w1015, index=w1012) -> (element=w1014:bool)
                              n621 = Increment(x=w1012) -> (x+1=w1008:i32)
                              n622 = case shown="True" w1014 {
                                tunnel: w1021 -> [w1022 w1039]
                                tunnel: w1016 -> [_ w1038]
                                tunnel: [w1022 w1037] -> w1020
                                tunnel: w1019 -> [_ w1036]
                                tunnel: w1018 -> [_ w1035]
                                tunnel: w1017 -> [_ w1034]
                                tunnel: w1012 -> [_ w1033]
                                tunnel: w1008 -> [_ w1024]
                                tunnel: w1016 -> [_ w1023]
                                frame False {
                                }
                                frame True {
                                n623 = flat-sequence {
                                tunnel: w1033 -> [w1042]
                                tunnel: w1035 -> [w1048]
                                tunnel: w1036 -> [w1049]
                                tunnel: w1038 -> [w1040]
                                tunnel: w1039 -> [w1050]
                                tunnel: [w1050] -> w1028
                                tunnel: [w1049] -> w1027
                                tunnel: [w1048] -> w1026
                                tunnel: [w1042] -> w1025
                                tunnel: [w1055] -> w1032
                                tunnel: [w1054] -> w1031
                                tunnel: [w1053] -> w1030
                                tunnel: [w1052] -> w1029
                                tunnel: w1028 -> [w1055]
                                tunnel: w1027 -> [w1054]
                                tunnel: w1026 -> [w1053]
                                tunnel: w1025 -> [w1052]
                                tunnel: [w1067] -> w1037
                                tunnel: w1034 -> [w1062]
                                tunnel: w1032 -> [w1068]
                                tunnel: w1031 -> [w1066]
                                tunnel: w1030 -> [w1065]
                                tunnel: w1029 -> [w1058]
                                tunnel: w1024 -> [w1262]
                                tunnel: w1023 -> [w1261]
                                frame #0 {
                                n624 = Increment(x=w1042) -> (x+1=w1041:i32)
                                n625 = Number To Decimal String(number=w1041) -> (decimal integer string=w1047:string)  [unwired: 1 in]
                                n626 = Concatenate Strings("L" ("write buffer"), w1047, "O1E" ("write buffer"), "\r") -> (w1046:string)
                                n627 = VISA Write(VISA resource name=w1040, write buffer=w1046) -> ()  [unwired: 1 in, 3 out]
                                }
                                frame #1 {
                                n628 = local read "before wait time"() -> (w1051:u32)
                                n629 = Wait (ms)(milliseconds to wait=w1051) -> ()  [unwired: 1 out]
                                }
                                frame #2 {
                                # "take image"
                                n630 = Increment(x=w1058) -> (x+1=w1057:i32)
                                n631 = Number To Decimal String(number=w1057) -> (decimal integer string=w1056:string)  [unwired: 1 in]
                                n632 = Number To Decimal String(number=w1062, width (-)=i16 2) -> (decimal integer string=w1064:string)
                                n633 = Search and Replace String(input string=w1064, search string=" ", replace string="0") -> (result string=w1059:string)  [unwired: 5 in, 3 out]
                                n634 = stacked-sequence {
                                tunnel: w1068 -> [_ w1081 w1149 _]
                                tunnel: [_ w1080 _ _] -> w1067
                                tunnel: [_ _ w1149 _] -> _
                                tunnel: w1066 -> [_ _ _ w1213]
                                tunnel: w1065 -> [_ _ w1140 w1212]
                                tunnel: w1058 -> [_ _ _ w1211]
                                tunnel: w1059 -> [_ _ w1139 w1209]
                                tunnel: w1057 -> [_ _ w1141 w1208]
                                tunnel: w1056 -> [_ _ w1142 w1207]
                                frame #0 {
                                n635 = flat-sequence {
                                frame #0 {
                                n636 = local read "ImagingMode"() -> (w1069:enum32{"WideField", "SIM"})
                                n637 = case shown="\"WideField\", Default" w1069 {
                                frame "WideField", Default {
                                # "set SLM"
                                n638 = dll-call lib="C:/Program Files/MetroCon-3.2/RepSend/R11CommLib-x64.dll" fn="R11_RpcRoSetSelected"("roIndex"=u16 15) -> ()  [unwired: 5 in, 2 out]
                                }
                                frame "SIM" {
                                }
                                }
                                }
                                frame #1 {
                                }
                                }
                                }
                                frame #1 {
                                # "set Laser On"
                                n639 = flat-sequence {
                                tunnel: w1081 -> [w1083]
                                tunnel: w1081 -> [w1092]
                                tunnel: [w1091] -> w1079
                                tunnel: [w1090] -> w1077
                                tunnel: [w1088] -> w1071
                                tunnel: w1079 -> [w1105]
                                tunnel: [w1105] -> w1078
                                tunnel: w1077 -> [w1104]
                                tunnel: [w1104] -> w1076
                                tunnel: [w1103] -> w1075
                                tunnel: [w1102] -> w1072
                                tunnel: w1071 -> [w1102]
                                tunnel: w1078 -> [w1110]
                                tunnel: w1076 -> [w1109]
                                tunnel: [w1108] -> w1080
                                tunnel: [w1107] -> w1074
                                tunnel: w1075 -> [w1107]
                                tunnel: [w1106] -> w1073
                                tunnel: w1072 -> [w1106]
                                tunnel: w1074 -> [w1112]
                                tunnel: w1073 -> [w1111]
                                frame #0 {
                                n640 = case shown="True" TRUE {
                                tunnel: w1083 -> [_ w1086]
                                frame False {
                                }
                                frame True {
                                w1084 = 0 items=["Idle", "Capturing"] ("Status")
                                n641 = property class="Camera" props=["IsOpen", "Status"](reference=w1086) -> ("Status"=w1085:i32)  [unwired: 1 in, 3 out]
                                n642 = Equal?(x=w1085, y=w1084) -> ()  [unwired: 1 out]
                                }
                                }
                                }
                                frame #1 {
                                }
                                frame #2 {
                                }
                                frame #3 {
                                n643 = Tick Count (ms)() -> (millisecond timer value=→"millisecond timer value":u32)
                                }
                                frame #4 {
                                n644 = control-ref of="Exposure Time"() -> (w1095:refnum<vi>)
                                n645 = local read "ImagingMode"() -> (w1088:enum32{"WideField", "SIM"})
                                n646 = property class="DigNum (strict)"(reference=w1095) -> ("Value"=w1089:dbl)  [unwired: 1 in, 2 out]
                                n647 = property class="Camera"(reference=w1092) -> (reference out=w1091:refnum<k24>, "Settings"=w1097:refnum<k24>)  [unwired: 1 in, 1 out]
                                n648 = case shown="\"WideField\", Default" w1088 {
                                tunnel: [u16 1 ("FramesToCapture") u16 33 ("FramesToCapture")] -> w1093
                                frame "WideField", Default {
                                }
                                frame "SIM" {
                                }
                                }
                                n649 = property class="CameraSettings"(reference=w1097, "Exposure"=w1089) -> (reference out=w1096:refnum<k24>)  [unwired: 1 in, 1 out]
                                n650 = Tick Count (ms)() -> (millisecond timer value=→"millisecond timer value 3":u32)
                                n651 = property class="CameraSettings" props=["XBinning", "FramesToCapture", "YBinning", "Exposure"](reference=w1096, "FramesToCapture"=w1093) -> (error out=w1090:errorcluster, "XBinning"=→"XBinning 2":u16, "YBinning"=→"YBinning 2":u16)  [unwired: 1 in, 2 out]
                                }
                                frame #5 {
                                n652 = Tick Count (ms)() -> (millisecond timer value=w1103:u32)
                                }
                                frame #6 {
                                n653 = invoke class="Camera" method="StartSequence"(reference=w1110, error in=w1109) -> (reference out=w1108:refnum<k24>)  [unwired: 1 in, 2 out]
                                }
                                frame #7 {
                                n654 = case shown="\"SIM\"" w1111 {
                                tunnel: w1112 -> [_ w1114]
                                frame "WideField", Default {
                                }
                                frame "SIM" {
                                n655 = for {
                                N: u16 15 ("FramesToCapture") -> [_]
                                tunnel: w1114 -> [w1122]
                                i -> [w1121]
                                n656 = Compound Arithmetic op=MULTIPLY("FramesToCapture", w1121, u16 2 ("FramesToCapture")) -> (w1118:i32)
                                n657 = Compound Arithmetic op=ADD("value", u16 10 ("FramesToCapture"), w1118) -> (w1117:i32)
                                n658 = flat-sequence {
                                tunnel: w1122 -> [w1124]
                                tunnel: w1117 -> [w1123]
                                tunnel: w1121 -> [w1130]
                                frame #0 {
                                n659 = while {
                                tunnel: w1124 -> [w1128]
                                tunnel: w1123 -> [w1127]
                                stop <- w1126 continue-if-true
                                n660 = Tick Count (ms)() -> (millisecond timer value=w1129:u32)
                                n661 = Subtract(x=w1129, y=w1128) -> (x-y=w1125:u32)
                                n662 = Less?(x=w1125, y=w1127) -> (x < y?=w1126:bool)
                                }
                                }
                                frame #1 {
                                # "set SLM"
                                n663 = dll-call lib="C:/Program Files/MetroCon-3.2/RepSend/R11CommLib-x64.dll" fn="R11_RpcRoSetSelected"("roIndex"=w1130) -> ()  [unwired: 5 in, 2 out]
                                }
                                }
                                }
                                }
                                }
                                }
                                frame #8 {
                                n664 = case shown="True" TRUE {
                                frame False {
                                }
                                frame True {
                                n665 = while {
                                stop <- w1134 stop-if-true
                                n666 = local read "millisecond timer value"() -> (w1137:u32)
                                n667 = local read "Exposure Time"() -> (w1135:dbl)
                                n668 = Tick Count (ms)() -> (millisecond timer value=w1138:u32)
                                n669 = Subtract(x=w1138, y=w1137) -> (x-y=w1136:u32)
                                n670 = Add(x="after wait time", y=w1135) -> (x+y=w1133:dbl)
                                n671 = Greater Or Equal?(x=w1136, y=w1133) -> (x >= y?=w1134:bool)
                                }
                                }
                                }
                                }
                                frame #9 {
                                # "blank laser"
                                }
                                }
                                }
                                frame #2 {
                                (unwired) TRUE
                                # "save image"
                                n672 = while {
                                tunnel: w1149 -> [w1206]
                                tunnel: [w1203] -> w1144
                                tunnel: [w1205] -> w1143
                                tunnel: [w1201] -> w1145
                                stop <- w1203 stop-if-true
                                w1204 = 0 items=["Idle", "Capturing"] ("Status")
                                n673 = property class="Camera"(reference=w1206) -> (reference out=w1205:refnum<k24>, "IsOpen"=w1201:bool, "Status"=w1202:i32)  [unwired: 1 in, 1 out]
                                n674 = Equal?(x=w1202, y=w1204) -> (x = y?=w1203:bool)
                                }
                                n675 = Equal?(x=w1145, y=TRUE) -> (x = y?=w1146:bool)
                                n676 = Equal?(x=w1146, y=w1144) -> (x = y?=w1148:bool)
                                n677 = case shown="True" w1148 {
                                tunnel: w1143 -> [w1150 w1160]
                                tunnel: [w1150 w1159] -> _
                                tunnel: w1142 -> [_ w1155]
                                tunnel: w1141 -> [_ w1154]
                                tunnel: w1140 -> [_ w1153]
                                tunnel: w1139 -> [_ w1152]
                                frame False {
                                n678 = One Button Dialog(message="Camera must be idle") -> ()  [unwired: 1 in, 1 out]
                                }
                                frame True {
                                (unwired) TRUE ("Boolean 3")
                                n679 = property class="Camera"(reference=w1160) -> (reference out=w1159:refnum<k24>, "AcquisitionBuffer"=w1158:refnum<k24>)  [unwired: 1 in, 1 out]
                                n680 = property class="AcqBuffer"(reference=w1158) -> ("BufferIndex"=w1157:i32)  [unwired: 1 in, 2 out]
                                n681 = local read "ImagingMode"() -> (w1156:enum32{"WideField", "SIM"})
                                n682 = case shown="\"WideField\", Default" w1156 {
                                tunnel: w1158 -> [w1187 w1200]
                                tunnel: w1157 -> [_ _]
                                tunnel: w1155 -> [w1173 _]
                                tunnel: w1154 -> [w1172 _]
                                tunnel: w1153 -> [w1171 _]
                                tunnel: w1152 -> [w1169 _]
                                frame "WideField", Default {
                                n683 = property class="AcqBuffer"(reference=w1187) -> ("FrameToDisplay"=w1186:refnum<k24>)  [unwired: 1 in, 2 out]
                                n684 = property class="Frame"(reference=w1186) -> ("RawImageData"=w1163:i16[])  [unwired: 1 in, 2 out]
                                n685 = Divide(x=w1163, y=16 ("Numeric 3")) -> (x/y=w1166:dbl[])
                                n686 = To Unsigned Word Integer(number=w1166) -> (unsigned 16bit integer=w1164:u16[])
                                n687 = In Range and Coerce(upper limit=255, x=w1164, lower limit=0) -> (coerced(x)=w1162:i32[])  [unwired: 1 out]
                                n688 = Array Size(array=w1162) -> (size(s)=w1185:i32)
                                n689 = Square Root(x=w1185) -> (sqrt(x)=w1184:dbl)
                                n690 = Concatenate Strings(w1173, "\\") -> (w1176:string)
                                n691 = To Unsigned Long Integer(number=w1184) -> (unsigned 32bit integer=w1183:u32)
                                n692 = for {
                                N: w1183 -> [_]
                                tunnel: w1162 -> [w1197]
                                tunnel: w1183 -> [w1194]
                                tunnel: [w1195] -> w1161 mode=indexing
                                i -> [w1193]
                                n693 = Subtract(x=w1194, y=w1193) -> (x-y=w1192:u32)
                                n694 = Decrement(x=w1192) -> (x-1=w1191:u32)
                                n695 = Multiply(x=w1194, y=w1191) -> (x*y=w1196:u32)
                                n696 = Array Subset(array=w1197, index=w1196, length=w1194) -> (w1195:i32[])
                                }
                                n697 = case shown="1, Default" w1172 {
                                tunnel: ["beads-" "signal1-" "virus-"] -> w1175
                                frame 1, Default {
                                }
                                frame 2 {
                                }
                                frame 3 {
                                }
                                }
                                n698 = Concatenate Strings(w1171, "c", w1176, w1175, w1169, ".bmp") -> (w1179:string)
                                n699 = String To Path(string=w1179) -> (path=w1170:path)
                                n700 = Multiply(x=w1161, y=65793) -> (x*y=w1181:i32[][])
                                n701 = call <vilib>:"Flatten Pixmap.vi"("24-bit pixmap"=w1181) -> ("image data"=w1180:T5)  [unwired: 10 in]
                                n702 = call <vilib>:"Write BMP File.vi"("image data"=w1180, "path to BMP file"=w1170) -> ()  [unwired: 8 in, 2 out]
                                }
                                frame "SIM" {
                                n703 = invoke class="AcqBuffer" method="SaveAsTiff"(reference=w1200, "startIndex"=u32 3, "endIndex"=u32 32 ("startIndex")) -> ()  [unwired: 2 in, 5 out]
                                }
                                }
                                }
                                }
                                }
                                frame #3 {
                                n704 = local read "ImagingMode"() -> (w1210:enum32{"WideField", "SIM"})
                                n705 = case shown="\"WideField\", Default" w1210 {
                                tunnel: w1213 -> [_ w1220]
                                tunnel: w1212 -> [_ w1219]
                                tunnel: w1209 -> [_ w1218]
                                tunnel: w1211 -> [_ _]
                                tunnel: w1208 -> [_ w1215]
                                tunnel: w1207 -> [_ w1214]
                                frame "WideField", Default {
                                }
                                frame "SIM" {
                                n706 = flat-sequence {
                                tunnel: [w1222] -> w1217
                                tunnel: [w1221] -> w1216
                                tunnel: w1220 -> [w1222]
                                tunnel: w1217 -> [w1257]
                                tunnel: w1216 -> [w1256]
                                tunnel: w1219 -> [w1246]
                                tunnel: w1218 -> [w1252]
                                tunnel: w1214 -> [w1251]
                                tunnel: w1215 -> [w1248]
                                frame #0 {
                                n707 = while {
                                tunnel: w1222 -> [w1229]
                                tunnel: [w1223] -> w1221
                                stop <- w1226 stop-if-true
                                n708 = List Folder(path=w1229) -> (filenames=w1228:string[])  [unwired: 3 in, 3 out]
                                n709 = Array Size(array=w1228) -> (size(s)=w1224:i32)
                                n710 = while {
                                tunnel: w1228 -> [w1239]
                                shift-right: [w1238] -> w1226
                                shift-left: FALSE -> [w1237]
                                tunnel: w1224 -> [w1235]
                                tunnel: [w1230] -> w1223
                                i -> [w1236]
                                stop <- w1231 stop-if-true
                                n711 = Index Array(array=w1239, index=w1236) -> (element=w1230:string)
                                n712 = Equal?(x=w1235, y=w1236) -> (x = y?=w1234:bool)
                                n713 = Match Pattern(string=w1230, regular expression=".tif") -> (offset past match=w1240:i32)  [unwired: 1 in, 3 out]
                                n714 = Equal?(x=w1240, y=-1) -> (x = y?=w1233:bool)
                                n715 = Not(x=w1233) -> (.not. x?=w1232:bool)
                                n716 = Or(x=w1234, y=w1232) -> (x .or. y?=w1231:bool)
                                n717 = Or(x=w1233, y=w1237) -> (x .or. y?=w1238:bool)
                                }
                                n718 = Wait (ms)(milliseconds to wait=u32 2) -> ()  [unwired: 1 out]
                                }
                                }
                                frame #1 {
                                n719 = Concatenate Strings(w1251, "\\") -> (w1249:string)
                                n720 = case shown="1, Default" w1248 {
                                tunnel: ["beads-" "signal1-" "virus-"] -> w1247
                                frame 1, Default {
                                }
                                frame 2 {
                                }
                                frame 3 {
                                }
                                }
                                n721 = Build Path(base path=w1257, name or relative path=w1256) -> (appended path=w1244:path)
                                "appended path" <- w1244
                                n722 = Concatenate Strings(w1246, "c", w1249, w1247, w1252, ".tif") -> (w1255:string)
                                n723 = String To Path(string=w1255) -> (path=w1254:path)
                                n724 = Move(source path=w1244, 9:TRUE ("overwrite (F)"), 10:w1254) -> ()  [unwired: 2 in, 3 out]
                                }
                                }
                                }
                                }
                                }
                                }
                                }
                                frame #3 {
                                n725 = local read "millisecond timer value"() -> (w1270:u32)
                                n726 = Tick Count (ms)() -> (millisecond timer value=w1269:u32)
                                "millisecond timer value 2" <- w1269
                                n727 = Number To Decimal String(number=w1262) -> (decimal integer string=w1266:string)  [unwired: 1 in]
                                n728 = Subtract(x=w1269, y=w1270) -> (x-y=→"time":u32)
                                n729 = Concatenate Strings("L" ("write buffer"), w1266, "O0E" ("write buffer"), "\r") -> (w1267:string)
                                n730 = VISA Write(VISA resource name=w1261, write buffer=w1267) -> ()  [unwired: 1 in, 3 out]
                                }
                                frame #4 {
                                n731 = Wait (ms)(milliseconds to wait=u32 100) -> ()  [unwired: 1 out]
                                }
                                }
                                }
                              }
                              n732 = Less?(x=w1008, y=3) -> (x < y?=w1010:bool)
                              n733 = local read "Stop"() -> (w1011:bool)
                              n734 = And(x=w1011, y=w1010) -> (x .and. y?=w1009:bool)
                            }
                            n735 = Wait (ms)(milliseconds to wait="milliseconds to wait") -> ()  [unwired: 1 out]
                          }
                          frame #1 {
                            n736 = flat-sequence {
                              tunnel: w1275 -> [w1290]
                              tunnel: [w1290] -> w1277
                              tunnel: w1274 -> [w1287]
                              tunnel: [w1279] -> w1272
                              tunnel: w1277 -> [w1298]
                              tunnel: [w1298] -> w1276
                              tunnel: [w1296] -> w1273
                              tunnel: w1272 -> [w1296]
                              tunnel: w1276 -> [w1305]
                              tunnel: w1273 -> [w1299]
                              frame #0 {
                                w1283 = i16 100 ("width (-)")
                                n737 = Decimal String To Number(string=w1287) -> (number=w1281:i32)  [unwired: 2 in, 1 out]
                                n738 = Absolute Value(x=w1281) -> (abs(x)=w1286:i32)
                                n739 = Sign(1:w1281) -> (0:w1282:i32)
                                n740 = Multiply(x=w1283, y=w1282) -> (x*y=w1284:i32)
                                n741 = Greater?(x=w1286, y=w1283) -> (0:w1285:bool)
                                n742 = Select(t=w1284, s=w1285, f=w1281) -> (s? t:f=w1280:i32)
                                n743 = Negate(x=w1280) -> (-x=w1279:i32)
                                n744 = Number To Hexadecimal String(1:i16 8 ("width (-)"), 2:w1279) -> (0:w1293:string)
                                n745 = Concatenate Strings("AA0100010000000000000000" ("write buffer"), w1293, "00000000" ("write buffer")) -> (w1291:string)
                                n746 = call "CRC-MODBUS.vi"("数据"=w1291) -> ("数据+CRC"=w1289:string)
                                n747 = call "Character-H16.vi"("string"=w1289) -> ("string 2"=w1288:string)
                                n748 = VISA Write(VISA resource name=w1290, write buffer=w1288) -> ()  [unwired: 1 in, 3 out]
                              }
                              frame #1 {
                                n749 = Wait (ms)(milliseconds to wait=u32 50) -> ()  [unwired: 1 out]
                              }
                              frame #2 {
                                n750 = local read "Current PositionZ:"() -> (w1301:string)
                                n751 = Decimal String To Number(string=w1301) -> (number=w1302:i32)  [unwired: 2 in, 1 out]
                                n752 = Add(x=w1302, y=w1299) -> (x+y=w1303:i32)
                                n753 = Number To Decimal String(number=w1303) -> (decimal integer string=w1300:string)  [unwired: 1 in]
                                n754 = local write "Current PositionZ:"(w1300) -> ()
                                n755 = VISA Write(VISA resource name=w1305, write buffer="ª\u0001\u0000\u0002\u0000\u0000\u0000\u0000\u0000\u0000\u0000\u0000\u0000\u0000\u0000\u0001\u0000\u0000\u0000\u0000…U") -> ()  [unwired: 1 in, 3 out]
                              }
                            }
                            n756 = local read "Z step(counts)"() -> (w1274:string)
                          }
                          frame #2 {
                            n757 = local read "Delay time(ms)"() -> (w1306:i16)
                            n758 = Wait (ms)(milliseconds to wait=w1306) -> ()  [unwired: 1 out]
                          }
                        }
                        n759 = Increment(x=w985) -> (x+1=w983:i32)
                        n760 = Equal?(x=w984, y=1) -> (x = y?=w994:bool)
                        n761 = Select(t=w993, s=w994, f=w983) -> (s? t:f=w992:i32)
                        "Current Z" <- w992
                        n762 = Less?(x=w983, y=w984) -> (x < y?=w987:bool)
                        n763 = local read "Stop"() -> (w988:bool)
                        n764 = And(x=w988, y=w987) -> (x .and. y?=w986:bool)
                      }
                    }
                  }
                  n765 = Increment(x=w806) -> (x+1=w805:i32)
                  n766 = Increment(x=w819) -> (x+1=w818:i32)
                  n767 = property on="Multicolumn Listbox" class="MCListbox (strict)"() -> ("ItemNames"=w812:string[][])  [unwired: 2 in, 2 out]
                  n768 = Array Size(array=w812) -> (size(s)=w811:i32[])
                  n769 = Index Array(array=w811, index=0) -> (element=w809:i32)
                  n770 = Increment(x=w807) -> (x+1=w808:i32)
                  n771 = Less?(x=w808, y=w809) -> (x < y?=w802:bool)
                  n772 = local read "Batch"() -> (w814:enum32{"Single", "Batch"})
                  n773 = Equal?(x=w814, y=enum32{"Single", "Batch"}."Batch") -> (x = y?=w803:bool)
                  n774 = local read "Stop"() -> (w804:bool)
                  n775 = Compound Arithmetic op=AND(w804, w803, w802) -> (w801:bool)
                }
              }
            }
          }
          event "Select Camera": Value Change {
            n776 = event-data() -> ()  [unwired: 1 in, 6 out]
            n777 = local read "Select Camera"() -> (w1312:string)
            n778 = local write item#7(w1312) -> ()
          }
          event "Open Camera": Value Change {
            n779 = event-data() -> ()  [unwired: 1 in, 6 out]
            n780 = case shown="True" "Open Camera" {
              tunnel: w1322 -> [w1328 w1343]
              tunnel: w1321 -> [w1327 w1341]
              tunnel: [w1327 w1329] -> w1319
              tunnel: [w1328 w1340] -> w1320
              tunnel: [w1326 w1335] -> w1318
              tunnel: w1317 -> [w1326 w1334]
              tunnel: [w1325 w1333] -> w1313
              tunnel: w1316 -> [w1325 w1332]
              tunnel: w1315 -> [w1324 w1330]
              tunnel: [w1324 w1331] -> w1314
              frame False {
              }
              frame True {
                # "check against null string"
                n781 = local read "Camera status"() -> (w1339:bool)
                n782 = local read item#7() -> (w1342:string)
                n783 = Not Equal?(x=w1342, y="") -> (x != y?=w1338:bool)
                n784 = Not(x=w1339) -> (.not. x?=w1337:bool)
                n785 = And(x=w1338, y=w1337) -> (x .and. y?=w1336:bool)
                n786 = case shown="True" w1336 {
                  tunnel: w1343 -> [w1345 w1360]
                  tunnel: w1342 -> [_ w1359]
                  tunnel: [w1349 w1358] -> w1329
                  tunnel: w1341 -> [w1349 _]
                  tunnel: [w1345 w1350] -> w1340
                  tunnel: [w1348 w1353] -> w1335
                  tunnel: w1334 -> [w1348 _]
                  tunnel: [w1347 w1352] -> w1333
                  tunnel: w1332 -> [w1347 _]
                  tunnel: [w1346 w1351] -> w1331
                  tunnel: w1330 -> [w1346 _]
                  frame False {
                  }
                  frame True {
                    n787 = flat-sequence {
                      tunnel: w1360 -> [w1369]
                      tunnel: w1359 -> [w1368]
                      tunnel: [w1366] -> w1357
                      tunnel: [w1365] -> w1356
                      tunnel: w1357 -> [w1413]
                      tunnel: w1356 -> [w1396]
                      tunnel: [w1413] -> w1355
                      tunnel: [w1370] -> w1354
                      tunnel: [w1397] -> w1353
                      tunnel: [w1386] -> w1352
                      tunnel: [w1379] -> w1351
                      tunnel: [w1416] -> w1358
                      tunnel: [w1417] -> w1350
                      tunnel: w1355 -> [w1417]
                      tunnel: w1354 -> [w1416]
                      frame #0 {
                        n788 = property class="Library"(reference=w1369) -> ("Instance"=w1363:refnum<k24>)  [unwired: 1 in, 2 out]
                        n789 = invoke class="Library" method="LoadCameras"(reference=w1363) -> (reference out=w1362:refnum<k24>)  [unwired: 2 in, 2 out]
                        n790 = invoke class="Library" method="GetCamera"(reference=w1362, "camName"=w1368) -> (reference out=w1367:refnum<k24>, "GetCamera"=w1361:refnum<k24>)  [unwired: 2 in, 2 out]
                        n791 = invoke class="Camera" method="Open"(reference=w1361) -> (reference out=w1365:refnum<k24>)  [unwired: 2 in, 2 out]
                        n792 = invoke class="Library" method="ShowImage"(reference=w1367, "cam"=w1365) -> (reference out=w1366:refnum<k24>)  [unwired: 2 in, 3 out]
                        n793 = Wait (ms)(milliseconds to wait=u32 500) -> ()  [unwired: 1 out]
                      }
                      frame #1 {
                        w1383 = 0.0 ("upper limit")
                        # "populate settings parameters"
                        n794 = property class="Camera"(reference=w1396) -> (reference out=w1370:refnum<k24>, "Settings"=w1412:refnum<k24>, "AcquisitionBuffer"=w1380:refnum<k24>)  [unwired: 1 in, 1 out]
                        n795 = control-ref of="8 Bit Histogram"() -> (w1399:refnum<vi>)
                        n796 = control-ref of="Capturing"() -> (w1395:refnum<vi>)
                        n797 = vi-ref "PVCamPropertyChangedCallbackForCameraState.vi"() -> ("vi reference"=w1394:refnum<vi>)
                        n798 = property class="CameraSettings"(reference=w1412) -> ("ExposureTime"=w1411:refnum<k24>, "SupportedBinning"=w1410:refnum<k24>, "ClearCycles"=w1409:refnum<k24>, "ClearingModes"=w1408:refnum<k24>, "ExposeOutMode"=w1407:refnum<k24>, "SpeedTable"=w1406:refnum<k24>, "SensorHeight"=w1404:refnum<k24>, "SensorWidth"=w1403:refnum<k24>, "ExposureMode"=w1400:refnum<k24>, "ExpRes"=w1385:refnum<k24>)  [unwired: 1 in, 2 out]
                        n799 = vi-ref "PVCamPropertyChangedCallbackForHistogram.vi"() -> ("vi reference"=w1398:refnum<vi>)
                        n800 = node(w1380, w1398, w1399) -> (w1397:refnum<k27>)  [unwired: 2 in, 1 out]
                        n801 = control-ref of="Exposure Time"() -> (w1391:refnum<vi>)
                        n802 = node(w1396, w1394, w1395) -> (w1386:refnum<k27>)  [unwired: 2 in, 1 out]
                        n803 = control-ref of="Trigger In Behaviour"() -> (w1388:refnum<vi>)
                        n804 = call "PopulateExposureTime.vi"("Exposure Time"=w1391, ".NET Refnum in"=w1411) -> ()  [unwired: 10 in]
                        n805 = control-ref of="Binning"() -> (w1393:refnum<vi>)
                        n806 = call "PopulateSupportedBinning.vi"("Binning"=w1393, ".NET Refnum in"=w1410) -> ()  [unwired: 10 in]
                        n807 = control-ref of="Sensor clearing mode"() -> (w1390:refnum<vi>)
                        n808 = call "PopulateClearModes.vi"("ClearingModes"=w1408, "ComboBox in"=w1390) -> ()  [unwired: 10 in]
                        n809 = control-ref of="Trigger Out Behaviour"() -> (w1389:refnum<vi>)
                        n810 = call "PopulateExpOut.vi"("ExposeOutMode"=w1407, "ComboBox in"=w1389) -> ()  [unwired: 10 in]
                        n811 = control-ref of="Clear Cycles"() -> (w1392:refnum<vi>)
                        n812 = call "PopulateClearCycles.vi"("ClearCycles"=w1409, "Digital in"=w1392) -> ()  [unwired: 10 in]
                        n813 = control-ref of="Dropped Frame"() -> (w1374:refnum<vi>)
                        n814 = control-ref of="Buffer Index"() -> (w1375:refnum<vi>)
                        n815 = call "PopulateTriggerModes.vi"("ExposureMode"=w1400, "ComboBox in"=w1388) -> ()  [unwired: 10 in]
                        n816 = control-ref of="Scrollbar"() -> (w1378:refnum<vi>)
                        n817 = control-ref of="Readout ports and speed"() -> (w1387:refnum<vi>)
                        n818 = control-ref of="Gain"() -> (w1405:refnum<vi>)
                        n819 = control-ref of="Exposure Resolution"() -> (w1384:refnum<vi>)
                        n820 = property class="PmNumericParam`1[[System.UInt32"(reference=w1404) -> ("Max"=w1401:u32)  [unwired: 1 in, 2 out]
                        n821 = property class="PmNumericParam`1[[System.UInt32"(reference=w1403) -> ("Max"=w1402:u32)  [unwired: 1 in, 2 out]
                        n822 = Bundle("Buffer Index"=w1375, "Dropped Frame"=w1374, "Scrollbar"=w1378) -> (w1377:T6)  [unwired: 1 in]
                        n823 = vi-ref "PVCamPropertyChangedEventCallbackForBufferIndexDroppedFrame.vi"() -> ("vi reference"=w1376:refnum<vi>)
                        n824 = call "PopulatePortsAndSpeedsGain.vi"("Ports and Speeds"=w1387, "Gain"=w1405, ".NET Refnum in"=w1406) -> ()  [unwired: 9 in]
                        n825 = call "PopulateExposureResolution.vi"("Exposure Resolution"=w1384, ".NET Refnum in"=w1385) -> ()  [unwired: 10 in]
                        n826 = node(w1380, w1376, w1377) -> (w1379:refnum<k27>)  [unwired: 2 in, 1 out]
                        n827 = local write "Height"(w1401) -> ()
                        n828 = local write "Full CCD Height"(w1401) -> ()
                        n829 = local write "Width"(w1402) -> ()
                        n830 = local write "Full CCD Width"(w1402) -> ()
                        n831 = property class="AcqBuffer"(reference=w1380) -> ("BufferSize"=w1373:i32)  [unwired: 1 in, 2 out]
                        n832 = control-ref of="Scrollbar"() -> (w1382:refnum<vi>)
                        n833 = In Range and Coerce(upper limit=w1373, x=w1383, lower limit=w1383) -> (coerced(x)=w1381:dbl)  [unwired: 1 out]
                        n834 = property class="Scroll (strict)"(reference=w1382, "Value"=w1381, "DocMax"=w1373, "DocMin"=0.0 ("Doc Min"), "PageSize"=1.0 ("Page Size")) -> ()  [unwired: 1 in, 2 out]
                      }
                      frame #2 {
                        n835 = local write "Camera status"(TRUE ("Camera Status")) -> ()
                        n836 = Wait (ms)(milliseconds to wait=u32 500) -> ()  [unwired: 1 out]
                      }
                    }
                  }
                }
              }
            }
          }
          event "Close Camera": Value Change {
            n837 = event-data() -> ()  [unwired: 1 in, 6 out]
            n838 = case shown="True" "Close Camera" {
              tunnel: w1424 -> [w1430 w1438]
              tunnel: [w1430 w1439] -> w1425
              tunnel: w1423 -> [w1429 w1436]
              tunnel: [w1429 w1435] -> w1422
              tunnel: w1421 -> [w1428 w1434]
              tunnel: [w1428 w1433] -> w1418
              tunnel: w1420 -> [w1427 w1432]
              tunnel: [w1427 w1431] -> w1419
              frame False {
              }
              frame True {
                n839 = local read "Camera status"() -> (w1437:bool)
                n840 = case shown="True" w1437 {
                  tunnel: [w1444 w1451] -> w1439
                  tunnel: w1438 -> [w1444 w1454]
                  tunnel: w1436 -> [w1442 w1450]
                  tunnel: [w1442 w1449] -> w1435
                  tunnel: w1434 -> [w1441 w1448]
                  tunnel: [w1441 w1447] -> w1433
                  tunnel: w1432 -> [w1440 w1446]
                  tunnel: [w1440 w1445] -> w1431
                  frame False {
                    n841 = One Button Dialog(message="Camera is not open") -> ()  [unwired: 1 in, 1 out]
                  }
                  frame True {
                    w1455 = 0 items=["Idle", "Capturing"] ("Status")
                    n842 = property class="Camera"(reference=w1454) -> (reference out=w1452:refnum<k24>, "IsOpen"=w1458:bool, "Status"=w1457:i32)  [unwired: 1 in, 1 out]
                    n843 = Equal?(x=w1458, y=TRUE) -> (x = y?=w1459:bool)
                    n844 = Equal?(x=w1457, y=w1455) -> (x = y?=w1460:bool)
                    n845 = Equal?(x=w1459, y=w1460) -> (x = y?=w1453:bool)
                    n846 = case shown="True" w1453 {
                      tunnel: w1452 -> [w1464 w1474]
                      tunnel: [w1464 w1472] -> w1451
                      tunnel: w1450 -> [w1463 w1470]
                      tunnel: [w1463 w1469] -> w1449
                      tunnel: w1448 -> [w1462 w1468]
                      tunnel: [w1462 w1467] -> w1447
                      tunnel: w1446 -> [w1461 w1466]
                      tunnel: [w1461 w1465] -> w1445
                      frame False {
                      }
                      frame True {
                        n847 = flat-sequence {
                          tunnel: w1474 -> [w1476]
                          tunnel: [w1480] -> w1473
                          tunnel: w1470 -> [w1478]
                          tunnel: w1468 -> [w1477]
                          tunnel: w1466 -> [w1475]
                          tunnel: w1473 -> [w1488]
                          tunnel: [w1487] -> w1471
                          tunnel: [w1523] -> w1472
                          tunnel: w1471 -> [w1523]
                          tunnel: [refnum<k27> refnum ("Event Callback")] -> w1469
                          tunnel: [refnum<k27> refnum ("Event Callback")] -> w1467
                          tunnel: [refnum<k27> refnum ("Event Callback")] -> w1465
                          tunnel: [refnum<k27> refnum ("Event Callback")] -> _
                          frame #0 {
                            n848 = Unregister For Events(event registration refnum=w1475) -> ()  [unwired: 1 in, 1 out]
                            n849 = property class="Camera"(reference=w1476) -> (reference out=w1480:refnum<k24>, "Settings"=w1484:refnum<k24>)  [unwired: 1 in, 1 out]
                            n850 = Unregister For Events(event registration refnum=w1478) -> ()  [unwired: 1 in, 1 out]
                            n851 = Unregister For Events(event registration refnum=w1477) -> ()  [unwired: 1 in, 1 out]
                            n852 = property class="CameraSettings"(reference=w1484) -> ("Regions"=w1483:refnum<k24>)  [unwired: 1 in, 2 out]
                            n853 = property class="PmObservableCollection`1[[PVCam"(reference=w1483) -> (reference out=w1481:refnum<k24>, "Count"=w1482:i32)  [unwired: 1 in, 1 out]
                            n854 = for {
                              N: w1482 -> [_]
                              tunnel: w1481 -> [w1486]
                              i -> [w1485]
                              n855 = invoke class="PmObservableCollection`1[[PVCam" method="RemoveAt"(reference=w1486, "index"=w1485) -> ()  [unwired: 2 in, 4 out]
                            }
                            n856 = Wait (ms)(milliseconds to wait=u32 500) -> ()  [unwired: 1 out]
                          }
                          frame #1 {
                            n857 = invoke class="Camera" method="Close"(reference=w1488) -> (reference out=w1487:refnum<k24>)  [unwired: 2 in, 2 out]
                          }
                          frame #2 {
                            w1489 = 0.0 ("Clear Cycle")
                            w1501 = 0 ("Full CCD Y")
                            w1502 = u32 1 ("Y Binning")
                            w1503 = 0.0 ("Clear Cycle")
                            # "Clear display"
                            n858 = control-ref of="Exposure Resolution"() -> (w1492:refnum<vi>)
                            n859 = control-ref of="Sensor clearing mode"() -> (w1517:refnum<vi>)
                            n860 = control-ref of="Trigger In Behaviour"() -> (w1521:refnum<vi>)
                            n861 = control-ref of="Trigger Out Behaviour"() -> (w1516:refnum<vi>)
                            n862 = local write "X Binning"(w1502) -> ()
                            n863 = local write "Y Binning"(w1502) -> ()
                            n864 = control-ref of="8 Bit Histogram"() -> (w1522:refnum<vi>)
                            n865 = control-ref of="Readout ports and speed"() -> (w1520:refnum<vi>)
                            n866 = property class="CmbBox"(reference=w1492, "Strings[]"=string[] [] ("Strings []"), "Value"="") -> ()  [unwired: 1 in, 2 out]
                            n867 = property class="CmbBox"(reference=w1517, "Strings[]"=string[] [] ("Strings []"), "Value"="") -> ()  [unwired: 1 in, 2 out]
                            n868 = property class="CmbBox"(reference=w1521, "Strings[]"=string[] [] ("Strings []"), "Value"="") -> ()  [unwired: 1 in, 2 out]
                            n869 = property class="CmbBox"(reference=w1516, "Strings[]"=string[] [] ("Strings []"), "Value"="") -> ()  [unwired: 1 in, 2 out]
                            n870 = property class="WFGraph (strict)"(reference=w1522, "Value"=i32[] []) -> ()  [unwired: 1 in, 2 out]
                            n871 = property class="CmbBox"(reference=w1520, "Strings[]"=string[] [] ("Strings []"), "Value"="") -> ()  [unwired: 1 in, 2 out]
                            n872 = control-ref of="Binning"() -> (w1518:refnum<vi>)
                            n873 = control-ref of="Gain"() -> (w1519:refnum<vi>)
                            n874 = local write "Camera status"(FALSE ("Camera Status")) -> ()
                            n875 = local write "Clear Cycles"(w1503) -> ()
                            n876 = local write "Exposure Time"(w1503) -> ()
                            n877 = local write "Full CCD Width"(w1501) -> ()
                            n878 = local write "Full CCD Height"(w1501) -> ()
                            n879 = local write "Full CCD X"(w1501) -> ()
                            n880 = local write "X"(w1501) -> ()
                            n881 = local write "Height"(w1501) -> ()
                            n882 = local write "Width"(w1501) -> ()
                            n883 = local write "Y"(w1501) -> ()
                            n884 = property class="CmbBox"(reference=w1518, "Strings[]"=string[] [] ("Strings []"), "Value"="") -> ()  [unwired: 1 in, 2 out]
                            n885 = property class="CmbBox"(reference=w1519, "Strings[]"=string[] [] ("Strings []"), "Value"="") -> ()  [unwired: 1 in, 2 out]
                            n886 = local write "Full CCD Y"(w1501) -> ()
                            n887 = local write "Dropped Frame"(w1489) -> ()
                            n888 = local write "Buffer Index"(w1489) -> ()
                            n889 = local write "Live status"(FALSE ("Live")) -> ()
                            n890 = Wait (ms)(milliseconds to wait=u32 500) -> ()  [unwired: 1 out]
                          }
                        }
                      }
                    }
                  }
                }
              }
            }
          }
          event "Get ROI": Value Change {
            n891 = event-data() -> ()  [unwired: 1 in, 6 out]
            n892 = case shown="True" "Get ROI" {
              tunnel: w1528 -> [w1530 w1533]
              tunnel: [w1530 w1532] -> w1527
              frame False {
              }
              frame True {
                n893 = local read "Camera status"() -> (w1531:bool)
                n894 = case shown="True" w1531 {
                  tunnel: w1533 -> [w1534 w1538]
                  tunnel: [w1534 w1536] -> w1532
                  frame False {
                    n895 = One Button Dialog(message="Camera is not open") -> ()  [unwired: 1 in, 1 out]
                  }
                  frame True {
                    w1544 = 0 items=["Idle", "Capturing"] ("Status")
                    n896 = property class="Camera"(reference=w1538) -> (reference out=w1537:refnum<k24>, "IsOpen"=w1543:bool, "Status"=w1545:i32)  [unwired: 1 in, 1 out]
                    n897 = Equal?(x=w1543, y=TRUE) -> (x = y?=w1541:bool)
                    n898 = Equal?(x=w1545, y=w1544) -> (x = y?=w1540:bool)
                    n899 = Equal?(x=w1541, y=w1540) -> (x = y?=w1539:bool)
                    n900 = case shown="True" w1539 {
                      tunnel: [w1546 w1552] -> w1536
                      tunnel: w1537 -> [w1546 w1554]
                      frame False {
                      }
                      frame True {
                        n901 = property class="Camera"(reference=w1554) -> (reference out=w1552:refnum<k24>, "Settings"=w1553:refnum<k24>)  [unwired: 1 in, 1 out]
                        n902 = property class="CameraSettings"(reference=w1553) -> ("Regions"=w1551:refnum<k24>)  [unwired: 1 in, 2 out]
                        n903 = property class="PmObservableCollection`1[[PVCam"(reference=w1551) -> (reference out=w1547:refnum<k24>, "Count"=w1550:i32)  [unwired: 1 in, 1 out]
                        n904 = Greater?(x=w1550, y=0) -> (0:w1548:bool)
                        n905 = case shown="True" w1548 {
                          tunnel: w1547 -> [_ w1556]
                          frame False {
                            n906 = One Button Dialog(message="ROI isn't created yet") -> ()  [unwired: 1 in, 1 out]
                          }
                          frame True {
                            n907 = invoke class="PmObservableCollection`1[[PVCam" method="get_Item"(reference=w1556, "index"=0) -> ("get_Item"=w1561:refnum<k24>)  [unwired: 2 in, 3 out]
                            n908 = property class="PmRegion"(reference=w1561) -> ("Height"=w1560:u16, "Y"=w1559:u16, "Width"=w1558:u16, "X"=w1557:u16)  [unwired: 1 in, 2 out]
                            n909 = local write "Height"(w1560) -> ()
                            n910 = local write "Width"(w1558) -> ()
                            n911 = local write "X"(w1557) -> ()
                            n912 = local write "Y"(w1559) -> ()
                          }
                        }
                      }
                    }
                  }
                }
              }
            }
          }
          event "Exposure Time", "Binning", "Sensor clearing mode", "Clear Cycles", "Readout ports and speed", "Trigger In Behaviour", "Exposure Resolution": Value Change {
            n913 = event-data() -> ()  [unwired: 1 in, 6 out]
            n914 = local read "Camera status"() -> (w1567:bool)
            n915 = case shown="True" w1567 {
              tunnel: [w1570 w1572] -> w1568
              tunnel: w1566 -> [w1570 w1571]
              frame False {
                n916 = One Button Dialog(message="Camera is not open") -> ()  [unwired: 1 in, 1 out]
              }
              frame True {
                w1579 = 0 items=["Idle", "Capturing"] ("Status")
                n917 = property class="Camera"(reference=w1571) -> (reference out=w1573:refnum<k24>, "IsOpen"=w1578:bool, "Status"=w1580:i32)  [unwired: 1 in, 1 out]
                n918 = Equal?(x=w1578, y=TRUE) -> (x = y?=w1576:bool)
                n919 = Equal?(x=w1580, y=w1579) -> (x = y?=w1575:bool)
                n920 = Equal?(x=w1576, y=w1575) -> (x = y?=w1574:bool)
                n921 = case shown="True" w1574 {
                  tunnel: w1573 -> [w1581 w1610]
                  tunnel: [w1581 w1609] -> w1572
                  frame False {
                  }
                  frame True {
                    n922 = property class="Camera"(reference=w1610) -> (reference out=w1609:refnum<k24>, "Settings"=w1608:refnum<k24>)  [unwired: 1 in, 1 out]
                    n923 = property class="CameraSettings"(reference=w1608) -> (reference out=w1603:refnum<k24>, "ExposureTime"=w1607:refnum<k24>, "SupportedBinning"=w1600:refnum<k24>, "ClearingModes"=w1606:refnum<k24>, "ClearCycles"=w1604:refnum<k24>, "ExposeOutMode"=w1605:refnum<k24>, "SpeedTable"=w1601:refnum<k24>, "ExposureMode"=w1602:refnum<k24>, "ExpRes"=w1585:refnum<k24>)  [unwired: 1 in, 1 out]
                    n924 = control-ref of="Clearing modes"() -> (w1595:refnum<vi>)
                    n925 = control-ref of="Exposure Time"() -> (w1599:refnum<vi>)
                    n926 = control-ref of="Binning"() -> (w1598:refnum<vi>)
                    n927 = control-ref of="Sensor clearing mode"() -> (w1593:refnum<vi>)
                    n928 = control-ref of="Trigger Out Behaviour"() -> (w1592:refnum<vi>)
                    n929 = control-ref of="Trigger In Behaviour"() -> (w1591:refnum<vi>)
                    n930 = control-ref of="Trigger Mode"() -> (w1594:refnum<vi>)
                    n931 = control-ref of="Clear Cycles"() -> (w1590:refnum<vi>)
                    n932 = call "SetExposureTime.vi"("ExposureTime"=w1607, "Settings"=w1603, "Digital in"=w1599) -> ()  [unwired: 9 in]
                    n933 = call "SetClearingMode.vi"("Clear mode"=w1593, "Clearing modes"=w1595, ".NET Refnum in"=w1606) -> ()  [unwired: 9 in]
                    n934 = call "SetTriggerMode.vi"("Trigger"=w1591, "ExposureMode"=w1602, "Digital in"=w1594) -> ()  [unwired: 9 in]
                    n935 = control-ref of="Readout ports and speed"() -> (w1586:refnum<vi>)
                    n936 = control-ref of="Gain"() -> (w1587:refnum<vi>)
                    n937 = control-ref of="Exp. out"() -> (w1583:refnum<vi>)
                    n938 = control-ref of="Y Binning"() -> (w1596:refnum<vi>)
                    n939 = control-ref of="X Binning"() -> (w1597:refnum<vi>)
                    n940 = control-ref of="CC Min"() -> (w1589:refnum<vi>)
                    n941 = control-ref of="CC Max"() -> (w1588:refnum<vi>)
                    n942 = call "SetBinning.vi"("SupportedBinning"=w1600, "Y Binning"=w1596, "Settings"=w1603, "X Binning"=w1597, "ComboBox in"=w1598) -> ()  [unwired: 7 in]
                    n943 = call "SetClearCycles.vi"("CC Max"=w1588, "CC Min"=w1589, "Clear Cycle"=w1590, ".NET Refnum in"=w1604) -> ()  [unwired: 8 in]
                    n944 = call "SetExpOut.vi"("Exp. in"=w1592, "ExposeOutMode"=w1605, "Digital in"=w1583) -> ()  [unwired: 9 in]
                    n945 = call "SetPortsAndSpeedsGain.vi"("Ports and Speeds"=w1586, "SpeedTable"=w1601, "ComboBox in"=w1587) -> ()  [unwired: 9 in]
                    n946 = control-ref of="Exposure Resolution"() -> (w1582:refnum<vi>)
                    n947 = control-ref of="Exposure Resolution"() -> (w1584:refnum<vi>)
                    n948 = call "SetExposureResolution.vi"("ExpRes"=w1585, "Exposure Resolution"=w1584, "ComboBox in"=w1582) -> ()  [unwired: 9 in]
                  }
                }
              }
            }
          }
          event "Save Image to TIFF": Value Change {
            n949 = event-data() -> ()  [unwired: 1 in, 6 out]
            n950 = case shown="True" "Save Image to TIFF" {
              tunnel: w1615 -> [w1617 w1619]
              tunnel: [w1617 w1618] -> w1614
              frame False {
              }
              frame True {
                n951 = local read "Camera status"() -> (w1620:bool)
                n952 = case shown="True" w1620 {
                  tunnel: w1619 -> [w1621 w1625]
                  tunnel: [w1621 w1622] -> w1618
                  frame False {
                  }
                  frame True {
                    w1626 = 0 items=["Idle", "Capturing"] ("Status")
                    n953 = property class="Camera"(reference=w1625) -> (reference out=w1623:refnum<k24>, "IsOpen"=w1629:bool, "Status"=w1628:i32)  [unwired: 1 in, 1 out]
                    n954 = Equal?(x=w1629, y=TRUE) -> (x = y?=w1630:bool)
                    n955 = Equal?(x=w1628, y=w1626) -> (x = y?=w1631:bool)
                    n956 = Equal?(x=w1630, y=w1631) -> (x = y?=w1624:bool)
                    n957 = case shown="True" w1624 {
                      tunnel: w1623 -> [w1633 w1638]
                      tunnel: [w1633 w1637] -> w1622
                      frame False {
                        n958 = One Button Dialog(message="Camera must be idle") -> ()  [unwired: 1 in, 1 out]
                      }
                      frame True {
                        n959 = property class="Camera"(reference=w1638) -> (reference out=w1637:refnum<k24>, "AcquisitionBuffer"=w1636:refnum<k24>)  [unwired: 1 in, 1 out]
                        n960 = property class="AcqBuffer"(reference=w1636) -> (reference out=w1634:refnum<k24>, "BufferIndex"=w1635:i32)  [unwired: 1 in, 1 out]
                        n961 = invoke class="AcqBuffer" method="SaveAsTiff"(reference=w1634, "nth"=w1635) -> ()  [unwired: 2 in, 4 out]
                      }
                    }
                  }
                }
              }
            }
          }
          event "Scrollbar": Value Change {
            n962 = event-data() -> ()  [unwired: 1 in, 6 out]
            n963 = local read "Camera status"() -> (w1639:bool)
            n964 = case shown="True" w1639 {
              tunnel: w1644 -> [w1645 w1650]
              tunnel: [w1645 w1648] -> w1643
              frame False {
                n965 = One Button Dialog(message="Camera is not open") -> ()  [unwired: 1 in, 1 out]
              }
              frame True {
                w1655 = 0 items=["Idle", "Capturing"] ("Status")
                n966 = property class="Camera"(reference=w1650) -> (reference out=w1649:refnum<k24>, "IsOpen"=w1654:bool, "Status"=w1656:i32)  [unwired: 1 in, 1 out]
                n967 = Equal?(x=w1654, y=TRUE) -> (x = y?=w1652:bool)
                n968 = Equal?(x=w1656, y=w1655) -> (x = y?=w1651:bool)
                n969 = Equal?(x=w1652, y=w1651) -> (x = y?=w1647:bool)
                n970 = case shown="True" w1647 {
                  tunnel: w1649 -> [w1657 w1665]
                  tunnel: [w1657 w1664] -> w1648
                  frame False {
                  }
                  frame True {
                    n971 = property class="Camera"(reference=w1665) -> (reference out=w1664:refnum<k24>, "AcquisitionBuffer"=w1660:refnum<k24>)  [unwired: 1 in, 1 out]
                    n972 = property class="AcqBuffer"(reference=w1660) -> (reference out=w1659:refnum<k24>, "BufferSize"=w1662:i32)  [unwired: 1 in, 1 out]
                    n973 = local read "Scrollbar"() -> (w1663:i32)
                    n974 = In Range and Coerce(upper limit=w1662, x=w1663, lower limit=0) -> (coerced(x)=w1658:i32)  [unwired: 1 out]
                    n975 = property class="AcqBuffer"(reference=w1659, "BufferIndex"=w1658) -> ()  [unwired: 1 in, 2 out]
                  }
                }
              }
            }
          }
          event "Gain": Value Change {
            n976 = event-data() -> ()  [unwired: 1 in, 6 out]
            n977 = local read "Camera status"() -> (w1671:bool)
            n978 = case shown="True" w1671 {
              tunnel: w1670 -> [w1673 w1676]
              tunnel: [w1673 w1674] -> w1669
              frame False {
                n979 = One Button Dialog(message="Camera is not open") -> ()  [unwired: 1 in, 1 out]
              }
              frame True {
                w1678 = 0 items=["Idle", "Capturing"] ("Status")
                n980 = property class="Camera"(reference=w1676) -> (reference out=w1675:refnum<k24>, "IsOpen"=w1681:bool, "Status"=w1680:i32)  [unwired: 1 in, 1 out]
                n981 = Equal?(x=w1681, y=TRUE) -> (x = y?=w1682:bool)
                n982 = Equal?(x=w1680, y=w1678) -> (x = y?=w1683:bool)
                n983 = Equal?(x=w1682, y=w1683) -> (x = y?=w1677:bool)
                n984 = case shown="True" w1677 {
                  tunnel: w1675 -> [w1684 w1687]
                  tunnel: [w1684 w1686] -> w1674
                  frame False {
                  }
                  frame True {
                    n985 = control-ref of="Gain"() -> (w1685:refnum<vi>)
                    n986 = call "SetGain.vi"("Gain"=w1685, ".NET Refnum in"=w1687) -> (".NET Refnum out"=w1686:refnum<k24>)  [unwired: 9 in]
                  }
                }
              }
            }
          }
          event "Y", "X", "Width", "Height": Value Change {
            n987 = event-data() -> ()  [unwired: 1 in, 6 out]
            n988 = local read "Camera status"() -> (w1692:bool)
            n989 = case shown="True" w1692 {
              tunnel: w1693 -> [w1694 w1699]
              tunnel: [w1694 w1696] -> w1689
              frame False {
                n990 = One Button Dialog(message="Camera is not open") -> ()  [unwired: 1 in, 1 out]
              }
              frame True {
                w1704 = 0 items=["Idle", "Capturing"] ("Status")
                n991 = property class="Camera"(reference=w1699) -> (reference out=w1697:refnum<k24>, "IsOpen"=w1703:bool, "Status"=w1705:i32)  [unwired: 1 in, 1 out]
                n992 = Equal?(x=w1703, y=TRUE) -> (x = y?=w1701:bool)
                n993 = Equal?(x=w1705, y=w1704) -> (x = y?=w1700:bool)
                n994 = Equal?(x=w1701, y=w1700) -> (x = y?=w1698:bool)
                n995 = case shown="True" w1698 {
                  tunnel: w1697 -> [w1706 w1709]
                  tunnel: [w1706 w1708] -> w1696
                  frame False {
                  }
                  frame True {
                    n996 = flat-sequence {
                      tunnel: w1709 -> [w1710]
                      tunnel: [w1710] -> w1707
                      tunnel: [w1752] -> w1708
                      tunnel: w1707 -> [w1759]
                      frame #0 {
                        # "if (!( x >= 0\n            && (x+width) <= full_width\n            &&  0 < width \n            && y >= 0\n            && (y+height) <= full_height\n            && 0 < height ))\n        {\n           printf(\"Incorrect range for a ROI. \\n\");\n        }"
                        # "1. Check ROI \n2. Set ROI"
                        n997 = local read "Width"() -> (w1738:u16)
                        n998 = local read "Full CCD Width"() -> (w1722:i32)
                        n999 = local read "X"() -> (w1739:u16)
                        n1000 = local read "Width"() -> (w1719:u16)
                        n1001 = Add(x=w1739, y=w1738) -> (x+y=w1721:u16)
                        n1002 = local read "Height"() -> (w1735:u16)
                        n1003 = Less Or Equal?(x=w1721, y=w1722) -> (x <= y?=w1732:bool)
                        n1004 = local read "Full CCD Height"() -> (w1718:i32)
                        n1005 = Less?(x=u16 0, y=w1719) -> (x < y?=w1731:bool)
                        n1006 = local read "X"() -> (w1741:u16)
                        n1007 = local read "Y"() -> (w1736:u16)
                        n1008 = local read "Y"() -> (w1734:u16)
                        n1009 = local read "Height"() -> (w1715:u16)
                        n1010 = Greater Or Equal?(x=w1741, y=u16 0) -> (x >= y?=w1733:bool)
                        n1011 = Greater Or Equal?(x=w1736, y=u16 0) -> (x >= y?=w1730:bool)
                        n1012 = Add(x=w1735, y=w1734) -> (x+y=w1717:u16)
                        n1013 = Less Or Equal?(x=w1717, y=w1718) -> (x <= y?=w1729:bool)
                        n1014 = And(x=w1733, y=w1732) -> (x .and. y?=w1727:bool)
                        n1015 = And(x=w1731, y=w1730) -> (x .and. y?=w1726:bool)
                        n1016 = Less?(x=u16 0, y=w1715) -> (x < y?=w1728:bool)
                        n1017 = And(x=w1727, y=w1726) -> (x .and. y?=w1725:bool)
                        n1018 = And(x=w1729, y=w1728) -> (x .and. y?=w1724:bool)
                        n1019 = And(x=w1725, y=w1724) -> (x .and. y?=w1723:bool)
                        n1020 = case shown="False" w1723 {
                          tunnel: [w1743 w1750] -> w1714
                          tunnel: [u16 0 ("X") w1749] -> w1712
                          tunnel: [u16 0 ("Y") w1748] -> w1713
                          tunnel: [w1744 w1747] -> w1711
                          frame False {
                            n1021 = local read "Full CCD Height"() -> (w1744:i32)
                            n1022 = local read "Full CCD Width"() -> (w1743:i32)
                            n1023 = One Button Dialog(message="Wrong ROI ! Resetting to full CCD") -> ()  [unwired: 1 in, 1 out]
                          }
                          frame True {
                            n1024 = local read "Height"() -> (w1747:u16)
                            n1025 = local read "Width"() -> (w1750:u16)
                            n1026 = local read "X"() -> (w1749:u16)
                            n1027 = local read "Y"() -> (w1748:u16)
                          }
                        }
                        n1028 = local write "X"(w1712) -> ()
                        n1029 = local write "Width"(w1714) -> ()
                        n1030 = local write "Height"(w1711) -> ()
                        n1031 = local write "Y"(w1713) -> ()
                      }
                      frame #1 {
                        n1032 = property class="Camera"(reference=w1759) -> (reference out=w1752:refnum<k24>, error out=w1758:errorcluster, "Settings"=w1757:refnum<k24>)  [unwired: 1 in]
                        n1033 = property class="CameraSettings"(reference=w1757, error in=w1758) -> ("Regions"=w1756:refnum<k24>)  [unwired: 2 out]
                        n1034 = property class="PmObservableCollection`1[[PVCam"(reference=w1756) -> (reference out=w1751:refnum<k24>, "Count"=w1754:i32)  [unwired: 1 in, 1 out]
                        n1035 = Greater?(x=w1754, y=0) -> (0:w1753:bool)
                        n1036 = case shown="True" w1753 {
                          tunnel: w1751 -> [_ w1761]
                          frame False {
                            n1037 = One Button Dialog(message="ROI is not created.") -> ()  [unwired: 1 in, 1 out]
                          }
                          frame True {
                            # "Display ROI"
                            n1038 = invoke class="PmObservableCollection`1[[PVCam" method="get_Item"(reference=w1761, "index"=0) -> ("get_Item"=w1763:refnum<k24>)  [unwired: 2 in, 3 out]
                            n1039 = local read "Height"() -> (w1764:u16)
                            n1040 = local read "Width"() -> (w1765:u16)
                            n1041 = local read "X"() -> (w1766:u16)
                            n1042 = local read "Y"() -> (w1767:u16)
                            n1043 = property class="PmRegion"(reference=w1763, "Height"=w1764, "Width"=w1765, "X"=w1766, "Y"=w1767) -> ()  [unwired: 1 in, 2 out]
                          }
                        }
                      }
                    }
                  }
                }
              }
            }
          }
          event "Full CCD": Value Change {
            n1044 = event-data() -> ()  [unwired: 1 in, 6 out]
            n1045 = case shown="True" "Full CCD" {
              tunnel: w1773 -> [w1774 w1777]
              tunnel: [w1774 w1776] -> w1772
              frame False {
              }
              frame True {
                n1046 = local read "Camera status"() -> (w1775:bool)
                n1047 = case shown="True" w1775 {
                  tunnel: w1777 -> [w1779 w1783]
                  tunnel: [w1779 w1781] -> w1776
                  frame False {
                    n1048 = One Button Dialog(message="Camera is not open") -> ()  [unwired: 1 in, 1 out]
                  }
                  frame True {
                    w1788 = 0 items=["Idle", "Capturing"] ("Status")
                    n1049 = property class="Camera"(reference=w1783) -> (reference out=w1780:refnum<k24>, "IsOpen"=w1787:bool, "Status"=w1789:i32)  [unwired: 1 in, 1 out]
                    n1050 = Equal?(x=w1787, y=TRUE) -> (x = y?=w1785:bool)
                    n1051 = Equal?(x=w1789, y=w1788) -> (x = y?=w1784:bool)
                    n1052 = Equal?(x=w1785, y=w1784) -> (x = y?=w1782:bool)
                    n1053 = case shown="True" w1782 {
                      tunnel: [w1790 w1797] -> w1781
                      tunnel: w1780 -> [w1790 w1798]
                      frame False {
                      }
                      frame True {
                        n1054 = property class="Camera"(reference=w1798) -> (reference out=w1797:refnum<k24>, "Settings"=w1796:refnum<k24>)  [unwired: 1 in, 1 out]
                        n1055 = property class="CameraSettings"(reference=w1796) -> ("Regions"=w1795:refnum<k24>)  [unwired: 1 in, 2 out]
                        n1056 = property class="PmObservableCollection`1[[PVCam"(reference=w1795) -> (reference out=w1791:refnum<k24>, "Count"=w1794:i32)  [unwired: 1 in, 1 out]
                        n1057 = Greater?(x=w1794, y=0) -> (0:w1792:bool)
                        n1058 = case shown="True" w1792 {
                          tunnel: w1791 -> [_ w1800]
                          frame False {
                            n1059 = One Button Dialog(message="ROI is not created.") -> ()  [unwired: 1 in, 1 out]
                          }
                          frame True {
                            w1808 = u16 0 ("X")
                            n1060 = invoke class="PmObservableCollection`1[[PVCam" method="get_Item"(reference=w1800, "index"=0) -> (reference out=w1813:refnum<k24>, "get_Item"=w1811:refnum<k24>)  [unwired: 2 in, 2 out]
                            n1061 = invoke class="PmObservableCollection`1[[PVCam" method="get_Item"(reference=w1813, "index"=0) -> ("get_Item"=w1801:refnum<k24>)  [unwired: 2 in, 3 out]
                            n1062 = local read "Full CCD Height"() -> (w1810:i32)
                            n1063 = local read "Full CCD Width"() -> (w1809:i32)
                            n1064 = property class="PmRegion"(reference=w1801) -> ("Height"=w1805:u16, "Width"=w1804:u16, "X"=w1803:u16, "Y"=w1802:u16)  [unwired: 1 in, 2 out]
                            n1065 = property class="PmRegion"(reference=w1811, "Height"=w1810, "Selected"=TRUE, "Width"=w1809, "X"=w1808, "Y"=w1808) -> ()  [unwired: 1 in, 2 out]
                            n1066 = local write "Width"(w1804) -> ()
                            n1067 = local write "X"(w1803) -> ()
                            n1068 = local write "Y"(w1802) -> ()
                            n1069 = local write "Height"(w1805) -> ()
                          }
                        }
                      }
                    }
                  }
                }
              }
            }
          }
          event "Live start": Value Change {
            n1070 = event-data() -> ()  [unwired: 1 in, 6 out]
            n1071 = case shown="True" "Live start" {
              tunnel: w1818 -> [w1820 w1823]
              tunnel: [w1820 w1822] -> w1817
              frame False {
              }
              frame True {
                n1072 = local read "Camera status"() -> (w1821:bool)
                n1073 = case shown="True" w1821 {
                  tunnel: w1823 -> [w1825 w1831]
                  tunnel: [w1825 w1828] -> w1822
                  frame False {
                    n1074 = One Button Dialog(message="Camera is not open") -> ()  [unwired: 1 in, 1 out]
                  }
                  frame True {
                    w1826 = 0 items=["Idle", "Capturing"] ("Status")
                    n1075 = property class="Camera"(reference=w1831) -> (reference out=w1829:refnum<k24>, "IsOpen"=w1835:bool, "Status"=w1827:i32)  [unwired: 1 in, 1 out]
                    n1076 = Equal?(x=w1827, y=w1826) -> (x = y?=w1832:bool)
                    n1077 = Equal?(x=w1835, y=TRUE) -> (x = y?=w1833:bool)
                    n1078 = Equal?(x=w1833, y=w1832) -> (x = y?=w1830:bool)
                    n1079 = case shown="True" w1830 {
                      tunnel: w1829 -> [w1836 w1842]
                      tunnel: [w1836 w1844] -> w1828
                      frame False {
                      }
                      frame True {
                        n1080 = control-ref of="Exposure Time"() -> (w1838:refnum<vi>)
                        n1081 = local write "Live status"(TRUE ("Live")) -> ()
                        n1082 = property class="DigNum (strict)"(reference=w1838) -> ("Value"=w1837:dbl)  [unwired: 1 in, 2 out]
                        n1083 = property class="Camera"(reference=w1842) -> (reference out=w1841:refnum<k24>, "Settings"=w1840:refnum<k24>)  [unwired: 1 in, 1 out]
                        n1084 = property class="CameraSettings"(reference=w1840, "Exposure"=w1837) -> (error out=w1839:errorcluster)  [unwired: 1 in, 1 out]
                        n1085 = invoke class="Camera" method="StartLive"(reference=w1841, error in=w1839) -> (reference out=w1844:refnum<k24>)  [unwired: 1 in, 2 out]
                      }
                    }
                  }
                }
              }
            }
          }
          event "Live stop": Value Change {
            n1086 = event-data() -> ()  [unwired: 1 in, 6 out]
            n1087 = case shown="True" "Live stop" {
              tunnel: w1849 -> [w1851 w1854]
              tunnel: [w1851 w1853] -> w1848
              frame False {
              }
              frame True {
                n1088 = local read "Camera status"() -> (w1852:bool)
                n1089 = case shown="True" w1852 {
                  tunnel: w1854 -> [w1855 w1860]
                  tunnel: [w1855 w1858] -> w1853
                  frame False {
                    n1090 = One Button Dialog(message="Camera is not open") -> ()  [unwired: 1 in, 1 out]
                  }
                  frame True {
                    w1865 = 1 items=["Idle", "Capturing"] ("Status")
                    n1091 = property class="Camera"(reference=w1860) -> (reference out=w1859:refnum<k24>, "IsOpen"=w1864:bool, "Status"=w1866:i32)  [unwired: 1 in, 1 out]
                    n1092 = Equal?(x=w1866, y=w1865) -> (x = y?=w1861:bool)
                    n1093 = Equal?(x=w1864, y=TRUE) -> (x = y?=w1862:bool)
                    n1094 = Equal?(x=w1862, y=w1861) -> (x = y?=w1857:bool)
                    n1095 = case shown="True" w1857 {
                      tunnel: w1859 -> [w1867 w1870]
                      tunnel: [w1867 w1869] -> w1858
                      frame False {
                      }
                      frame True {
                        n1096 = invoke class="Camera" method="Stop"(reference=w1870) -> (reference out=w1869:refnum<k24>)  [unwired: 2 in, 2 out]
                        n1097 = local write "Live status"(FALSE ("Live")) -> ()
                      }
                    }
                  }
                }
              }
            }
          }
          event "Histogram On/Off": Value Change {
            n1098 = event-data() -> ()  [unwired: 1 in, 6 out]
            n1099 = local read "Camera status"() -> (w1871:bool)
            n1100 = case shown="True" w1871 {
              tunnel: w1874 -> [w1879 w1881]
              tunnel: [w1879 w1884] -> w1873
              tunnel: "Histogram On/Off" -> [_ w1883]
              frame False {
                n1101 = One Button Dialog(message="Camera is not open") -> ()  [unwired: 1 in, 1 out]
              }
              frame True {
                n1102 = property class="Camera"(reference=w1881) -> (reference out=w1882:refnum<k24>, "IsOpen"=w1880:bool)  [unwired: 1 in, 1 out]
                n1103 = case shown="True" w1880 {
                  tunnel: w1882 -> [w1885 w1888]
                  tunnel: [w1885 w1887] -> w1884
                  tunnel: w1883 -> [_ w1886]
                  frame False {
                  }
                  frame True {
                    n1104 = global write "PVCamGlobalVariables.vi" "Histogram Enabled"(w1886) -> ()
                    n1105 = property class="Camera"(reference=w1888) -> (reference out=w1887:refnum<k24>, "AcquisitionBuffer"=w1889:refnum<k24>)  [unwired: 1 in, 1 out]
                    n1106 = property class="AcqBuffer"(reference=w1889, "UseScaling"=w1886) -> ()  [unwired: 1 in, 2 out]
                  }
                }
              }
            }
          }
        }
      }
    }
    frame #2 {
      # "Library"
      # "camera SR"
      # "camera status SR"
      # "histogram SR"
      # "Buffer Index SR"
      n1107 = invoke class="Library" method="Release"(reference=w1890) -> (reference out=w1891:refnum<k24>)  [unwired: 2 in, 2 out]
      n1108 = Close Reference(reference=w1891) -> ()  [unwired: 1 in, 1 out]
    }
    frame #3 {
      # "We must call GC::Collect() to remove all the references. This is a known issue.\nhttp://www.ni.com/product-documentation/53586/en/#468139_by_Category"
      n1109 = invoke class="GC" method="Collect"() -> ()  [unwired: 3 in, 3 out]
    }
  }
  n1110 = stacked-sequence {
    frame #0 {
      n1111 = Read from Text File(file (use dialog)=path "C:/Users/Dell/Desktop/SIMImaging -电动平移台 -V4/stage.txt", count=3 ("index")) -> (text=w1899:string[])  [unwired: 2 in, 3 out]
      n1112 = Index Array(array=w1899, index #1=0 ("index"), index #2=1 ("index"), index #3=2 ("index")) -> (element #1=w1894:string, element #2=w1893:string, element #3=w1892:string)
      n1113 = local write "Current PositionZ:"(w1892) -> ()
      n1114 = local write "Current PositionY"(w1893) -> ()
      n1115 = local write "Current PositionX"(w1894) -> ()
    }
    frame #1 {
      n1116 = while {
        stop <- FALSE stop-if-true
        n1117 = flat-sequence {
          frame #0 {
            n1118 = local read "Current PositionX"() -> (w1905:string)
            n1119 = local read "Current PositionY"() -> (w1904:string)
            n1120 = local read "Current PositionZ:"() -> (w1906:string)
            n1121 = Build Array(w1905, w1904, w1906) -> (w1907:string[])
            n1122 = Write to Text File(file (use dialog)=path "C:/Users/Dell/Desktop/SIMImaging -电动平移台 -V3/stage.txt", text=w1907) -> ()  [unwired: 2 in, 3 out]
          }
        }
        n1123 = Wait Until Next ms Multiple(millisecond multiple=500) -> ()  [unwired: 1 out]
      }
    }
  }
  n1124 = local write "Laser"(w8) -> ()
  n1125 = while {
    tunnel: w1 -> [w1908]
    stop <- FALSE stop-if-true
    n1126 = event shown="[0] \"StopX\": Value Change" {
      selector: _ -> [_]
      dyn-events: _ -> [_]
      timeout: _ -> [_]
      tunnel: w1908 -> [w1911]
      event "StopX": Value Change {
        n1127 = event-data() -> ()  [unwired: 1 in, 6 out]
        n1128 = VISA Write(VISA resource name=w1911, write buffer="ª\u0001\u0000\u0016\u0000\u0000\u0000\u0001\u0000\u0000\u0000\u0000\u0000\u0000\u0000\u0000\u0000\u0000\u0000\u0000õ\u0010") -> ()  [unwired: 1 in, 3 out]
      }
    }
  }
  n1129 = local write "Histogram On/Off"(w23) -> ()
  n1130 = while {
    stop <- FALSE stop-if-true
    n1131 = local read "Current PositionY"() -> (w1919:string)
    n1132 = local read "Current PositionX"() -> (w1920:string)
    n1133 = local read "StageY1"() -> (w1916:i32)
    n1134 = local read "StageX1"() -> (w1915:i32)
    n1135 = local read "Ratio"() -> (w1917:dbl)
    n1136 = local read "Angle"() -> (w1914:dbl)
    n1137 = local read "MapX1"() -> (w1913:i32)
    n1138 = local read "MapY1"() -> (w1912:i32)
    n1139 = local read "new picture"() -> (w1921:picture)
    n1140 = stacked-sequence {
      seq-local: [w1924 _] -> [_ w1957]
      tunnel: w1921 -> [w1955 _]
      tunnel: w1920 -> [w1954 _]
      tunnel: w1919 -> [w1953 _]
      tunnel: [_ w1964] -> w1918
      tunnel: w1917 -> [w1946 w1963]
      tunnel: w1916 -> [w1941 w1962]
      tunnel: w1915 -> [w1940 w1961]
      tunnel: w1914 -> [w1935 w1960]
      tunnel: w1913 -> [w1934 w1959]
      tunnel: w1912 -> [w1933 w1958]
      tunnel: [w1929 _] -> _
      tunnel: [w1927 _] -> _
      frame #0 {
        w1950 = 10 ("y")
        n1141 = Decimal String To Number(string=w1954) -> (number=w1944:i32)  [unwired: 2 in, 1 out]
        n1142 = Decimal String To Number(string=w1953) -> (number=w1945:i32)  [unwired: 2 in, 1 out]
        n1143 = Subtract(x=w1944, y=w1940) -> (x-y=w1943:i32)
        n1144 = Subtract(x=w1945, y=w1941) -> (x-y=w1942:i32)
        n1145 = Negate(x=w1935) -> (-x=w1925:dbl)
        n1146 = Multiply(x=w1943, y=w1946) -> (x*y=w1939:dbl)
        n1147 = expression code="(x/180.0)*pi" "degrees to radians"(w1925) -> (w1930:dbl)
        n1148 = Multiply(x=w1942, y=w1946) -> (x*y=w1938:dbl)
        n1149 = call-poly <vilib>:"2D Cartesian Coordinate Rotation.vi"("theta"=w1930, "y"=w1938, "x"=w1939) -> ("y out"=w1936:dbl, "x out"=w1937:dbl)  [unwired: 6 in, 1 out]
        n1150 = Add(x=w1937, y=w1934) -> (x+y=w1929:dbl)
        n1151 = Add(x=w1933, y=w1936) -> (x+y=w1927:dbl)
        n1152 = Subtract(x=w1929, y=5.0 ("x")) -> (x-y=w1932:dbl)
        n1153 = Add(x=w1950, y=w1932) -> (x+y=w1951:dbl)
        n1154 = Subtract(x=w1927, y=5.0 ("x")) -> (x-y=w1931:dbl)
        n1155 = Add(x=w1950, y=w1931) -> (x+y=w1949:dbl)
        n1156 = Bundle(w1932, w1931, w1951, w1949) -> (w1952:cluster{dbl, dbl, dbl, dbl})  [unwired: 1 in]
        n1157 = call <vilib>:"Draw Oval.vi"("picture"=w1955, "rect"=w1952, "fill?(F)"=TRUE, "color(black)"=u32 6618880) -> ("new picture"=w1924:picture)  [unwired: 5 in]
      }
      frame #1 {
        n1158 = property on="Multicolumn Listbox" class="MCListbox (strict)"() -> ("ItemNames"=w1956:string[][])  [unwired: 2 in, 2 out]
        n1159 = for {
          tunnel: w1963 -> [w2002]
          tunnel: w1962 -> [w1997]
          tunnel: w1961 -> [w1996]
          tunnel: w1960 -> [w1991]
          tunnel: w1959 -> [w1990]
          tunnel: w1958 -> [w1989]
          tunnel: [w1966] -> _
          tunnel: [w1965] -> _
          shift-right: [w1969] -> w1964
          shift-left: w1957 -> [w2004]
          tunnel: w1956 -> [w1984] mode=indexing
          w1975 = 30 ("y")
          n1160 = Index Array(array=w1984, index #1=1 ("y"), index #2=2 ("y"), index #3=0 ("y")) -> (element #1=w1981:string, element #2=w1980:string, element #3=w1978:string)
          n1161 = Decimal String To Number(string=w1981) -> (number=w2000:i32)  [unwired: 2 in, 1 out]
          n1162 = Decimal String To Number(string=w1980) -> (number=w2001:i32)  [unwired: 2 in, 1 out]
          n1163 = Subtract(x=w2000, y=w1996) -> (x-y=w1999:i32)
          n1164 = Subtract(x=w2001, y=w1997) -> (x-y=w1998:i32)
          n1165 = Negate(x=w1991) -> (-x=w1985:dbl)
          n1166 = Multiply(x=w1999, y=w2002) -> (x*y=w1995:dbl)
          n1167 = expression code="(x/180.0)*pi" "degrees to radians"(w1985) -> (w1988:dbl)
          n1168 = Multiply(x=w1998, y=w2002) -> (x*y=w1994:dbl)
          n1169 = call-poly <vilib>:"2D Cartesian Coordinate Rotation.vi"("theta"=w1988, "y"=w1994, "x"=w1995) -> ("y out"=w1992:dbl, "x out"=w1993:dbl)  [unwired: 6 in, 1 out]
          n1170 = Add(x=w1993, y=w1990) -> (x+y=w1966:dbl)
          n1171 = Add(x=w1989, y=w1992) -> (x+y=w1965:dbl)
          n1172 = Subtract(x=w1966, y=15.0 ("x")) -> (x-y=w1973:dbl)
          n1173 = Bundle(w1966, w1965) -> (w1977:cluster{dbl, dbl})  [unwired: 1 in]
          n1174 = Subtract(x=w1965, y=15.0 ("x")) -> (x-y=w1972:dbl)
          n1175 = call <vilib>:"Draw Text at Point.vi"("text color(black)"=u32 16711680 ("color(black)"), "text"=w1978, "origin"=w1977, "picture"=w2004) -> ("new picture"=w1970:picture)  [unwired: 6 in, 1 out]
          n1176 = Add(x=w1975, y=w1972) -> (x+y=w1974:dbl)
          n1177 = Add(x=w1975, y=w1973) -> (x+y=w1976:dbl)
          n1178 = Bundle(w1973, w1972, w1976, w1974) -> (w1971:cluster{dbl, dbl, dbl, dbl})  [unwired: 1 in]
          n1179 = call <vilib>:"Draw Rectangle.vi"("picture"=w1970, "rect"=w1971, "color(black)"=u32 9567230, "pen"=T7 {"Width"=2, "Style"=enum."Dash"}) -> ("new picture"=w1969:picture)  [unwired: 5 in]
        }
      }
    }
    n1180 = Wait (ms)(milliseconds to wait=u32 200) -> ()  [unwired: 1 out]
    n1181 = local write "Map"(w1918) -> ()
  }
  n1182 = flat-sequence {
    frame #0 {
      n1183 = dll-call lib="C:/Program Files/MetroCon-3.2/RepSend/R11CommLib-x64.dll" fn="FDD_DevOpenWinUSB"("devPath"="\\\\?\\usb#vid_19ec&pid_0503#0117000518#{54ED7AC9-CC23-4165-BE32-79016BAFB950}", "timeout"=u16 1024) -> ("FDD_RESULT"=w2006:u16)  [unwired: 5 in, 2 out]
      n1184 = Equal To 0?(x=w2006) -> (x = 0?=→"SLM connected":bool)
    }
    frame #1 {
      n1185 = dll-call lib="C:/Program Files/MetroCon-3.2/RepSend/R11CommLib-x64.dll" fn="R11_RpcRoGetCount"() -> ("roCount"=→"Order Count":u16)  [unwired: 5 in, 2 out]
    }
  }
  n1186 = while {
    stop <- FALSE stop-if-true
    n1187 = property on="Map" class="Pict"() -> ("Mouse"=→"Mouse":T1)  [unwired: 2 in, 2 out]
    n1188 = Wait (ms)(milliseconds to wait=u32 300) -> ()  [unwired: 1 out]
  }
  n1189 = global write "PVCamGlobalVariables.vi" "Histogram Enabled"(w23) -> ()
  n1190 = while {
    tunnel: w1 -> [w2013]
    stop <- FALSE stop-if-true
    n1191 = event shown="[1] \"Get1\": Mouse Down" {
      selector: _ -> [_ _ _ _]
      dyn-events: _ -> [_ _ _ _]
      timeout: _ -> [_ _ _ _]
      tunnel: w2013 -> [_ _ _ w2027]
      event Timeout {
        n1192 = event-data() -> ()  [unwired: 1 in, 3 out]
      }
      event "Get1": Mouse Down {
        n1193 = event-data() -> ()  [unwired: 1 in, 8 out]
        n1194 = local read "Current PositionX"() -> (w2016:string)
        n1195 = local read "Current PositionY"() -> (w2015:string)
        n1196 = Decimal String To Number(string=w2016) -> (number=→"StageX1":i32)  [unwired: 2 in, 1 out]
        n1197 = Decimal String To Number(string=w2015) -> (number=→"StageY1":i32)  [unwired: 2 in, 1 out]
      }
      event "Get2": Mouse Down {
        n1198 = event-data() -> ()  [unwired: 1 in, 8 out]
        n1199 = local read "Current PositionX"() -> (w2022:string)
        n1200 = local read "Current PositionY"() -> (w2020:string)
        n1201 = Decimal String To Number(string=w2020) -> (number=→"StageY2":i32)  [unwired: 2 in, 1 out]
        n1202 = Decimal String To Number(string=w2022) -> (number=→"StageX2":i32)  [unwired: 2 in, 1 out]
      }
      event "Map": Mouse Down {
        n1203 = event-data() -> ()  [unwired: 1 in, 8 out]
        n1204 = property on="Map" class="Pict"() -> ("Mouse"=w2023:T1)  [unwired: 2 in, 2 out]
        n1205 = Unbundle(w2023) -> ("Mouse Position"=w2024:cluster{"X":i32, "Y":i32})  [unwired: 1 out]
        n1206 = Unbundle(w2024) -> ("X"=w2026:i32, "Y"=w2025:i32)
        n1207 = case shown="False" "ScreenMove" {
          tunnel: w2027 -> [_ w2072]
          tunnel: w2026 -> [w2030 w2038]
          tunnel: w2025 -> [w2029 w2037]
          frame False {
            n1208 = case shown="True" "map1" {
              tunnel: w2030 -> [_ w2036]
              tunnel: w2029 -> [_ w2035]
              frame False {
              }
              frame True {
                "MapX1" <- w2036
                "MapY1" <- w2035
              }
            }
            n1209 = case shown="True" "map2" {
              tunnel: w2030 -> [_ w2034]
              tunnel: w2029 -> [_ w2033]
              frame False {
              }
              frame True {
                "MapY2" <- w2033
                "MapX2" <- w2034
              }
            }
          }
          frame True {
            w2063 = 10 ("y")
            n1210 = flat-sequence {
              tunnel: w2072 -> [w2078]
              tunnel: [w2078] -> w2071
              tunnel: [w2079] -> w2070
              tunnel: [w2080] -> w2069
              tunnel: w2040 -> [w2076]
              tunnel: w2039 -> [w2075]
              tunnel: w2071 -> [w2099]
              tunnel: [w2099] -> w2068
              tunnel: [w2097] -> w2067
              tunnel: w2070 -> [w2097]
              tunnel: [w2096] -> w2066
              tunnel: w2069 -> [w2096]
              tunnel: w2068 -> [w2111]
              tunnel: w2067 -> [w2105]
              tunnel: w2066 -> [w2104]
              frame #0 {
                n1211 = local read "Current PositionY"() -> (w2081:string)
                n1212 = To Long Integer(number=w2076) -> (32bit integer=w2073:i32)
                n1213 = local read "Current PositionX"() -> (w2082:string)
                n1214 = To Long Integer(number=w2075) -> (32bit integer=w2074:i32)
                n1215 = Decimal String To Number(string=w2081) -> (number=w2089:i32)  [unwired: 2 in, 1 out]
                n1216 = Decimal String To Number(string=w2082) -> (number=w2087:i32)  [unwired: 2 in, 1 out]
                n1217 = Subtract(x=w2087, y=w2073) -> (x-y=w2083:i32)
                n1218 = Subtract(x=w2089, y=w2074) -> (x-y=w2084:i32)
                n1219 = Negate(x=w2083) -> (-x=w2080:i32)
                n1220 = Negate(x=w2084) -> (-x=w2079:i32)
                n1221 = Number To Hexadecimal String(1:i16 8 ("width (-)"), 2:w2079) -> (0:w2086:string)
                n1222 = Number To Hexadecimal String(1:i16 8 ("width (-)"), 2:w2080) -> (0:w2085:string)
                n1223 = Concatenate Strings("AA010001" ("write buffer"), w2085, w2086, "00000000" ("write buffer"), "00000000" ("write buffer")) -> (w2094:string)
                n1224 = call "CRC-MODBUS.vi"("数据"=w2094) -> ("数据+CRC"=w2093:string)
                n1225 = call "Character-H16.vi"("string"=w2093) -> ("string 2"=w2092:string)
                n1226 = VISA Write(VISA resource name=w2078, write buffer=w2092) -> ()  [unwired: 1 in, 3 out]
              }
              frame #1 {
                n1227 = Wait (ms)(milliseconds to wait=u32 100) -> ()  [unwired: 1 out]
              }
              frame #2 {
                n1228 = local read "Current PositionX"() -> (w2101:string)
                n1229 = local read "Current PositionY"() -> (w2102:string)
                n1230 = Decimal String To Number(string=w2101) -> (number=w2106:i32)  [unwired: 2 in, 1 out]
                n1231 = Decimal String To Number(string=w2102) -> (number=w2108:i32)  [unwired: 2 in, 1 out]
                n1232 = Add(x=w2106, y=w2104) -> (x+y=w2107:i32)
                n1233 = Add(x=w2108, y=w2105) -> (x+y=w2109:i32)
                n1234 = Number To Decimal String(number=w2107) -> (decimal integer string=w2100:string)  [unwired: 1 in]
                n1235 = Number To Decimal String(number=w2109) -> (decimal integer string=w2103:string)  [unwired: 1 in]
                n1236 = local write "Current PositionY"(w2103) -> ()
                n1237 = local write "Current PositionX"(w2100) -> ()
                n1238 = VISA Write(VISA resource name=w2111, write buffer="ª\u0001\u0000\u0002\u0000\u0000\u0000\u0001\u0000\u0000\u0000\u0001\u0000\u0000\u0000\u0000\u0000\u0000\u0000\u0000·„") -> ()  [unwired: 1 in, 3 out]
              }
            }
            n1239 = local read "MapX1"() -> (w2053:i32)
            n1240 = local read "MapY1"() -> (w2052:i32)
            n1241 = Subtract(x=w2037, y=w2052) -> (x-y=w2049:i32)
            n1242 = Subtract(x=w2038, y=w2053) -> (x-y=w2051:i32)
            n1243 = local read "new picture"() -> (w2055:picture)
            n1244 = local read "Ratio"() -> (w2050:dbl)
            n1245 = local read "Angle"() -> (w2045:dbl)
            n1246 = Divide(x=w2049, y=w2050) -> (x/y=w2047:dbl)
            n1247 = Divide(x=w2051, y=w2050) -> (x/y=w2048:dbl)
            n1248 = expression code="(x/180.0)*pi" "degrees to radians"(w2045) -> (w2046:dbl)
            n1249 = Subtract(x=w2038, y=5.0 ("x")) -> (x-y=w2059:dbl)
            n1250 = Add(x=w2063, y=w2059) -> (x+y=w2064:dbl)
            n1251 = Subtract(x=w2037, y=5.0 ("x")) -> (x-y=w2058:dbl)
            n1252 = Add(x=w2063, y=w2058) -> (x+y=w2062:dbl)
            n1253 = Bundle(w2059, w2058, w2064, w2062) -> (w2065:cluster{dbl, dbl, dbl, dbl})  [unwired: 1 in]
            n1254 = call-poly <vilib>:"2D Cartesian Coordinate Rotation.vi"("theta"=w2046, "y"=w2047, "x"=w2048) -> ("y out"=w2043:dbl, "x out"=w2044:dbl)  [unwired: 6 in, 1 out]
            n1255 = local read "StageX1"() -> (w2042:i32)
            n1256 = local read "StageY1"() -> (w2041:i32)
            n1257 = call <vilib>:"Draw Oval.vi"("picture"=w2055, "rect"=w2065, "fill?(F)"=TRUE, "color(black)"=u32 6618880) -> ("new picture"=w2054:picture)  [unwired: 5 in]
            n1258 = Add(x=w2043, y=w2041) -> (x+y=w2039:dbl)
            n1259 = Add(x=w2042, y=w2044) -> (x+y=w2040:dbl)
            n1260 = local write "Map"(w2054) -> ()
          }
        }
      }
    }
  }
  n1261 = while {
    stop <- FALSE stop-if-true
    n1262 = event shown="[1] \"LoadMap\": Mouse Down" {
      selector: _ -> [_ _]
      dyn-events: _ -> [_ _]
      timeout: _ -> [_ _]
      event Timeout {
        n1263 = event-data() -> ()  [unwired: 1 in, 3 out]
      }
      event "LoadMap": Mouse Down {
        n1264 = event-data() -> ()  [unwired: 1 in, 8 out]
        n1265 = call <vilib>:"Read JPEG File.vi"("path to JPEG file"="Path") -> ("image data"=w2116:T5)  [unwired: 8 in, 2 out]
        n1266 = property on="Map" class="Pict"() -> ("Draw Area Size"=w2113:T8)  [unwired: 2 in, 2 out]
        n1267 = call <vilib>:"Unflatten Pixmap.vi"("image data"=w2116) -> ("24-bit pixmap"=w2119:u32[][])  [unwired: 4 in, 6 out]
        n1268 = Array Size(array=w2119) -> (size(s)=w2122:i32[])
        n1269 = Array Max & Min(array=w2122) -> (max value=w2121:i32)  [unwired: 3 out]
        n1270 = Unbundle(w2113) -> ("Height"=w2120:u32)  [unwired: 1 out]
        n1271 = Divide(x=w2120, y=w2121) -> (x/y=w2118:dbl)
        n1272 = for {
          N: w2120 -> [_]
          tunnel: w2120 -> [w2129]
          tunnel: w2119 -> [w2128]
          tunnel: w2118 -> [w2126]
          tunnel: [w2124] -> w2117 mode=indexing
          i -> [w2127]
          n1273 = Divide(x=w2127, y=w2126) -> (x/y=w2125:dbl)
          n1274 = for {
            N: w2129 -> [_]
            tunnel: w2128 -> [w2135]
            tunnel: w2126 -> [w2133]
            tunnel: w2125 -> [w2130]
            tunnel: [w2132] -> w2124 mode=indexing
            i -> [w2134]
            n1275 = Divide(x=w2134, y=w2133) -> (x/y=w2131:dbl)
            n1276 = Index Array(array=w2135, index (row)=w2130, index (col)=w2131) -> (element=w2132:u32)
          }
        }
        n1277 = call <vilib>:"Flatten Pixmap.vi"("24-bit pixmap"=w2117) -> ("image data"=w2115:T5)  [unwired: 10 in]
        n1278 = call <vilib>:"Draw Flattened Pixmap.vi"("image data"=w2115) -> ("new picture"=→"new picture" →"Map":picture)  [unwired: 8 in]
      }
    }
  }
  n1279 = property on="Exposure" class="DigNum (strict)"("Visible"=w27) -> ()  [unwired: 2 in, 2 out]
  n1280 = property on="YBinning" class="DigNum (strict)"("Visible"=w27) -> ()  [unwired: 2 in, 2 out]
  n1281 = property on="Y Binning" class="DigNum (strict)"("Visible"=w27) -> ()  [unwired: 2 in, 2 out]
  n1282 = property on="X Binning" class="DigNum (strict)"("Visible"=w27) -> ()  [unwired: 2 in, 2 out]
  n1283 = property on="CC Max" class="DigNum (strict)"("Visible"=w27) -> ()  [unwired: 2 in, 2 out]
  n1284 = property on="Full CCD Y" class="DigNum (strict)"("Visible"=w27) -> ()  [unwired: 2 in, 2 out]
  n1285 = property on="Clearing modes" class="DigNum (strict)"("Visible"=w27) -> ()  [unwired: 2 in, 2 out]
  n1286 = property on="CC Min" class="DigNum (strict)"("Visible"=w27) -> ()  [unwired: 2 in, 2 out]
  n1287 = property on="Full CCD Height" class="DigNum (strict)"("Visible"=w27) -> ()  [unwired: 2 in, 2 out]
  n1288 = property on="Exp. out" class="DigNum (strict)"("Visible"=w27) -> ()  [unwired: 2 in, 2 out]
  n1289 = property on="XBinning" class="DigNum (strict)"("Visible"=w27) -> ()  [unwired: 2 in, 2 out]
  n1290 = property on="Full CCD X" class="DigNum (strict)"("Visible"=w27) -> ()  [unwired: 2 in, 2 out]
  n1291 = property on="Full CCD Width" class="DigNum (strict)"("Visible"=w27) -> ()  [unwired: 2 in, 2 out]
  n1292 = property on="Trigger Mode" class="DigNum (strict)"("Visible"=w27) -> ()  [unwired: 2 in, 2 out]
  n1293 = while {
    stop <- FALSE stop-if-true
    n1294 = event shown="[1] \"Match\": Mouse Down" {
      selector: _ -> [_ _]
      dyn-events: _ -> [_ _]
      timeout: _ -> [_ _]
      event Timeout {
        n1295 = event-data() -> ()  [unwired: 1 in, 3 out]
      }
      event "Match": Mouse Down {
        n1296 = event-data() -> ()  [unwired: 1 in, 8 out]
        n1297 = local read "StageX2"() -> (w2155:i32)
        n1298 = local read "StageY2"() -> (w2153:i32)
        n1299 = local read "MapX2"() -> (w2151:i32)
        n1300 = local read "MapY2"() -> (w2149:i32)
        n1301 = local read "MapX1"() -> (w2150:i32)
        n1302 = local read "StageY1"() -> (w2152:i32)
        n1303 = local read "StageX1"() -> (w2154:i32)
        n1304 = local read "MapY1"() -> (w2148:i32)
        n1305 = Subtract(x=w2150, y=w2154) -> (x-y=→"Shift1":i32)
        n1306 = Subtract(x=w2148, y=w2152) -> (x-y=→"Shift2":i32)
        n1307 = Subtract(x=w2155, y=w2154) -> (x-y=w2146:i32)
        n1308 = Subtract(x=w2153, y=w2152) -> (x-y=w2147:i32)
        n1309 = Subtract(x=w2149, y=w2148) -> (x-y=w2138:i32)
        n1310 = Subtract(x=w2151, y=w2150) -> (x-y=w2137:i32)
        n1311 = Multiply(x=w2146, y=w2146) -> (x*y=w2161:i32)
        n1312 = Multiply(x=w2137, y=w2137) -> (x*y=w2164:i32)
        n1313 = Multiply(x=w2147, y=w2147) -> (x*y=w2160:i32)
        n1314 = Multiply(x=w2138, y=w2138) -> (x*y=w2163:i32)
        n1315 = Add(x=w2161, y=w2160) -> (x+y=w2159:i32)
        n1316 = Add(x=w2164, y=w2163) -> (x+y=w2162:i32)
        n1317 = Square Root(x=w2159) -> (sqrt(x)=w2158:dbl)
        n1318 = Square Root(x=w2162) -> (sqrt(x)=w2157:dbl)
        n1319 = Divide(x=w2157, y=w2158) -> (x/y=→"Ratio":dbl)
        n1320 = Divide(x=w2138, y=w2137) -> (x/y=w2143:dbl)
        n1321 = Divide(x=w2147, y=w2146) -> (x/y=w2145:dbl)
        n1322 = Inverse Tangent(1:w2143) -> (0:w2142:dbl)
        n1323 = Inverse Tangent(1:w2145) -> (0:w2144:dbl)
        n1324 = expression code="(x/pi)*180.0" "radians to degrees"(w2142) -> (w2141:dbl)
        n1325 = expression code="(x/pi)*180.0" "radians to degrees"(w2144) -> (w2140:dbl)
        n1326 = Subtract(x=w2141, y=w2140) -> (x-y=→"Angle":dbl)
      }
    }
  }
  "LabVIEW app version" <- "1.0"
  "8 Bit Histogram" <- i32[] [] ("8 Bit Histogram")
  "Capturing" <- FALSE ("Capturing")
  "Buffer Index" <- 0.0 ("Buffer Index")
  "Dropped Frame" <- 0.0 ("Dropped Frame")
